vi "TelemetryPRO-2_XCAN.vi"() -> ()   [LabVIEW 2017]
uses:
  <vilib>/Platform/TimedLoop/XDataNode/timing_clust.ctl
  <vilib>/Platform/TimedLoop/XDataNode/nitl_modes.ctl
  <vilib>/Platform/TimedLoop/XDataNode/wakeup.ctl
  <vilib>/nican/nican.llb/ncNetAttr.ctl
  <vilib>/Utility/file.llb/Read From Spreadsheet File (string).vi
  <vilib>/xnet/xnet.llb/XNET Create Session (Frame Input Stream).vi
  <vilib>/xnet/xnet.llb/XNET Read (Frame CAN).vi
  <vilib>/Utility/file.llb/Write To Spreadsheet File (string).vi
  <vilib>/Platform/TimedLoop/XDataNode/XDataNode.xnode
  <resource>/objmgr/xnet.rc
  <vilib>/Platform/TimedLoop/XDataNode/XDNodeRunTimeDep.lvlib
panel:
  out "GasPedal Heartbeat":dbl format="%.2f"
  out "Brake Force":u16(slide) scale=0.0..1500.0
  out "Brake Force":u16
  out "BP_rear":i16
  out "BP_front":i16
  out "Front / Rear Brake Pressure":cluster{u16, u16}
  out "Negative Torque Demand":u8
  out "Raw Negative Torque":u8
  out "BrakeForce":u8
  out "Cones3 2":T1(array[cluster])
  out "Cones2 2":T1(array[cluster])
  out "Cones1 2":T1(array[cluster])
  out "(hi.lo) 3":u64 format="%064b"
  out "Cones3":T1(array[cluster])
  out "(hi.lo) 2":u64 format="%064b"
  out "Cones2":T1(array[cluster])
  in  "ConeType":cluster{"Col":dbl, "X":dbl, "Y":dbl}
  out "(hi.lo)":u64 format="%064b"
  out "Cones1":T1(array[cluster])
  out "IGBT Temperature":T2(graph)
  out "XY Graph 4":cluster{"X":dbl, "Y":dbl}[](graph)
  out "Array":u8[](array[numeric])
  out "Numeric 2":u8
  out "SlipControl_Enabled":bool
  out "AMK_AV":bool
  out "Torque 2":bool
  out "BreakPoint":u8
  out "Slope":u16
  out "Damper Travel FR [mm]":dbl
  out "Damper Travel RR [mm]":dbl
  out "Damper Travel FL [mm]":dbl
  in  "Wheel Travel FR":dbl=1000.0
  in  "Wheel Travel FL Offset":dbl=1000.0
  in  "Wheel Travel RR Offset":dbl=1000.0
  out "Damper Travel RL [mm]":dbl
  in  "Wheel Travel RL Offset":dbl=1000.0
  out "HV Cell Voltage":u16(graph)
  out "accY 2":dbl
  out "accZ 2":dbl
  out "TorqRaw 2":u16
  in  "Brake Min 3":dbl=426.0
  out "BPRV":bool
  out "BPFV":bool
  out "BPFV":bool
  out "BPFSV":bool
  out "STA2":bool
  out "STA1":bool
  out "TPS2V":bool
  out "TPS1V":bool
  out "Apps2":dbl
  out "Apps1":dbl
  out "APPS1":u8(slide) scale=0.0..100.0
  out "APPS2":u8(slide) scale=0.0..100.0
  out "Brake Pedal Fore Supply":dbl
  out "Brake Pedal Force":dbl
  in  "CAN1 Enable 2":bool
  in  "CAN0 Enable 2":bool
  out "Status LEDs Red":bool[](array[boolean])
  out "Status LEDs Green":bool[](array[boolean])
  out "Numeric":dbl
  out "TCU speed":cluster{dbl, "AccelXRaw":dbl, dbl}(graph)
  out "AccelYRaw":dbl
  out "AccelXRaw":dbl
  in  "Acc Y offset":dbl
  in  "Acc X offset 2":dbl
  in  "OffsetFilter":dbl=0.01
  out "IsStopped":bool
  out "Acc Z 2":dbl
  out "Acc X 2":dbl
  out "Roll 2":dbl
  out "Acc Y 2":dbl
  out "Yaw 2":dbl
  in  "Acc Z offset":dbl
  out "Vel_acc":dbl=-0.0098098
  in  "New Lap":bool
  out "Energy":dbl[](array[numeric])
  out "Wheel Travel FL":u16
  out "Wheel Travel FR":u16
  out "Wheel Travel RL":u16
  out "Wheel Travel RR":u16
  out "Acc X":dbl
  out "Roll":dbl
  out "Yaw":dbl
  out "Acc Y":dbl
  out "Acc Z":dbl
  out "accY":dbl
  out "accZ":dbl
  out "Intensity Graph":dbl[][](graph)
  in  "Rollrate offset":dbl
  out "XY Graph 2":cluster{dbl[], dbl[]}(graph)
  out "Derate":bool[](array[boolean])
  out "Torq_sum":dbl
  in  "Play":bool
  in  "Timestep":u32
  in  "stop":bool
  in  "start":bool
  in  "pause":bool
  in  "Progress":i32(slide) min=0 step=60 scale=-1.0..61354011.0 scale format="%.0p"
  out "Time Stamp":string="2\r\n60"
  out "Charge Voltage":dbl
  out "Charge Curr":dbl
  in  "Tab Control":T3(tab)
  in  "Rows to read":i32=60
  in  "Data Path":path=path "D:/__BME-FRT/2016/2016-05-19/2016_05_19_tokol_endurance_00005_00001.csv"
  in  "CAN1 Enable":bool
  in  "CAN0 Enable":bool
  in  "Data Source":u16(ring) items=["Wi-Fi", "CAN-USB", "Log Analysis", "XCAN-USB"]
  in  "Port":u16=8998
  in  "Exit":bool
  in  "Log Path":path=path "D:/__BME-FRT/2016/test.txt"
  in  "Log Enable":bool
  out "WiFi Error":errorcluster
  in  "Length":u16=10
  out "CAN0 Error":errorcluster
  out "CAN1 Error":errorcluster
  out "Log Error":errorcluster
  out "CAN Message":u8[][](array[numeric])=[[2, 1, 128, 63, 0, 0, 129, 162, 129, 155], [2, 17, 23, 61, 0, 1, 0, 0, 0, 0], [3, 64, 252, 0, 0, 0, 27, 55, 27, 0], [2, 16, 115, 16, 37, 0, 203, 0, 0, 0], [4, 17, 23, 61, 0, 1, 0, 0, 0, 0], [2, 0, 128, 44, 0, 0, 136, 1, 7, 207], [2, 1, 128, 63, 0, 0, 129, 162, 129, 155], [2, 17, 23, 61, 0, 1, 0, 0, 0, 0], [4, 34, 0, 33, 0, 30, 0, 0, 0, 0], [4, 80, 148, 60, 128, 0, 0, 0, 0, 0], [1, 116, 84, 128, 0, 0, 190, 127, 8, 37], [2, 16, 116, 15, 111, 0, 203, 0, 0, 0], [1, 120, 211, 127, 0, 0, 193, 158, 8, 215], [1, 180, 84, 128, 0, 0, 223, 126, 2, 100], [1, 124, 0, 0, 0, 0, 189, 126, 8, 75], [1, 184, 62, 128, 2, 15, 59, 127, 2, 219], [4, 17, 23, 61, 0, 1, 0, 0, 0, 0], [1, 188, 0, 0, 0, 0, 136, 158, 2, 110], [2, 0, 128, 44, 0, 0, 136, 1, 7, 207], [2, 1, 128, 63, 0, 0, 129, 162, 129, 155], [2, 17, 23, 61, 0, 1, 0, 0, 0, 0], [3, 64, 252, 0, 0, 0, 27, 55, 27, 0], [4, 48, 10, 15, 219, 0, 96, 0, 0, 0], [3, 49, 128, 255, 0, 0, 0, 0, 0, 0], [2, 16, 117, 0, 0, 0, 203, 0, 0, 0], [4, 17, 23, 61, 0, 1, 0, 0, 0, 0], [2, 0, 128, 44, 0, 0, 136, 1, 7, 207], [2, 1, 128, 63, 0, 0, 129, 162, 129, 155], [2, 17, 23, 61, 0, 1, 0, 0, 0, 0], [3, 32, 112, 255, 0, 0, 0, 0, 0, 0], [4, 34, 0, 30, 0, 31, 0, 0, 0, 0], [1, 116, 87, 128, 0, 0, 184, 127, 9, 218], [1, 120, 203, 127, 1, 37, 194, 158, 9, 222], [2, 16, 118, 0, 0, 0, 205, 0, 0, 0], [1, 124, 0, 0, 0, 0, 176, 126, 9, 211], [1, 180, 90, 128, 0, 0, 215, 126, 3, 116], [1, 184, 50, 128, 3, 19, 44, 127, 3, 114], [4, 17, 23, 61, 0, 1, 0, 0, 0, 0], [1, 188, 0, 0, 0, 0, 147, 158, 3, 235], [2, 0, 128, 43, 0, 0, 136, 1, 7, 207], [2, 1, 128, 63, 0, 0, 129, 162, 129, 155], [2, 17, 23, 61, 0, 1, 0, 0, 0, 0], [3, 64, 252, 0, 0, 0, 38, 55, 38, 0], [2, 16, 119, 0, 0, 0, 202, 0, 0, 0], [4, 17, 23, 61, 0, 1, 0, 0, 0, 0], [2, 0, 128, 43, 0, 0, 136, 2, 7, 207], [2, 1, 128, 63, 0, 0, 129, 162, 129, 155], [2, 17, 23, 61, 0, 1, 0, 0, 0, 0], [4, 34, 0, 20, 0, 26, 0, 0, 0, 0], [1, 116, 78, 128, 0, 0, 179, 127, 10, 75], [1, 120, 206, 127, 2, 57, 194, 158, 10, 132], [2, 16, 120, 16, 37, 0, 200, 0, 210, 0], [1, 180, 90, 128, 0, 0, 206, 126, 4, 188], [1, 124, 0, 0, 0, 0, 157, 126, 10, 65], [1, 184, 39, 128, 4, 3, 33, 127, 4, 7], [4, 17, 23, 61, 0, 1, 0, 0, 0, 0], [1, 188, 0, 0, 0, 0, 153, 158, 4, 183], [2, 0, 128, 43, 0, 0, 136, 2, 7, 207], [2, 1, 128, 63, 0, 0, 129, 162, 129, 155], [2, 17, 23, 61, 0, 1, 0, 0, 0, 0]] format="%02x"
  out "CAN ID":u16[](array[numeric])=[513, 529, 832, 528, 1041, 512, 513, 529, 1058, 1104, 372, 528, 376, 436, 380, 440, 1041, 444, 512, 513, 529, 832, 1072, 817, 528, 1041, 512, 513, 529, 800, 1058, 372, 376, 528, 380, 436, 440, 1041, 444, 512, 513, 529, 832, 528, 1041, 512, 513, 529, 1058, 372, 376, 528, 436, 380, 440, 1041, 444, 512, 513, 529] format="%x"
  out "CAN Message 2":u8[][](array[numeric])=[[2, 1, 128, 63, 0, 0, 129, 162, 129, 155], [2, 17, 23, 61, 0, 1, 0, 0, 0, 0], [3, 64, 252, 0, 0, 0, 27, 55, 27, 0], [2, 16, 115, 16, 37, 0, 203, 0, 0, 0], [4, 17, 23, 61, 0, 1, 0, 0, 0, 0], [2, 0, 128, 44, 0, 0, 136, 1, 7, 207], [2, 1, 128, 63, 0, 0, 129, 162, 129, 155], [2, 17, 23, 61, 0, 1, 0, 0, 0, 0], [4, 34, 0, 33, 0, 30, 0, 0, 0, 0], [4, 80, 148, 60, 128, 0, 0, 0, 0, 0], [1, 116, 84, 128, 0, 0, 190, 127, 8, 37], [2, 16, 116, 15, 111, 0, 203, 0, 0, 0], [1, 120, 211, 127, 0, 0, 193, 158, 8, 215], [1, 180, 84, 128, 0, 0, 223, 126, 2, 100], [1, 124, 0, 0, 0, 0, 189, 126, 8, 75], [1, 184, 62, 128, 2, 15, 59, 127, 2, 219], [4, 17, 23, 61, 0, 1, 0, 0, 0, 0], [1, 188, 0, 0, 0, 0, 136, 158, 2, 110], [2, 0, 128, 44, 0, 0, 136, 1, 7, 207], [2, 1, 128, 63, 0, 0, 129, 162, 129, 155], [2, 17, 23, 61, 0, 1, 0, 0, 0, 0], [3, 64, 252, 0, 0, 0, 27, 55, 27, 0], [4, 48, 10, 15, 219, 0, 96, 0, 0, 0], [3, 49, 128, 255, 0, 0, 0, 0, 0, 0], [2, 16, 117, 0, 0, 0, 203, 0, 0, 0], [4, 17, 23, 61, 0, 1, 0, 0, 0, 0], [2, 0, 128, 44, 0, 0, 136, 1, 7, 207], [2, 1, 128, 63, 0, 0, 129, 162, 129, 155], [2, 17, 23, 61, 0, 1, 0, 0, 0, 0], [3, 32, 112, 255, 0, 0, 0, 0, 0, 0], [4, 34, 0, 30, 0, 31, 0, 0, 0, 0], [1, 116, 87, 128, 0, 0, 184, 127, 9, 218], [1, 120, 203, 127, 1, 37, 194, 158, 9, 222], [2, 16, 118, 0, 0, 0, 205, 0, 0, 0], [1, 124, 0, 0, 0, 0, 176, 126, 9, 211], [1, 180, 90, 128, 0, 0, 215, 126, 3, 116], [1, 184, 50, 128, 3, 19, 44, 127, 3, 114], [4, 17, 23, 61, 0, 1, 0, 0, 0, 0], [1, 188, 0, 0, 0, 0, 147, 158, 3, 235], [2, 0, 128, 43, 0, 0, 136, 1, 7, 207], [2, 1, 128, 63, 0, 0, 129, 162, 129, 155], [2, 17, 23, 61, 0, 1, 0, 0, 0, 0], [3, 64, 252, 0, 0, 0, 38, 55, 38, 0], [2, 16, 119, 0, 0, 0, 202, 0, 0, 0], [4, 17, 23, 61, 0, 1, 0, 0, 0, 0], [2, 0, 128, 43, 0, 0, 136, 2, 7, 207], [2, 1, 128, 63, 0, 0, 129, 162, 129, 155], [2, 17, 23, 61, 0, 1, 0, 0, 0, 0], [4, 34, 0, 20, 0, 26, 0, 0, 0, 0], [1, 116, 78, 128, 0, 0, 179, 127, 10, 75], [1, 120, 206, 127, 2, 57, 194, 158, 10, 132], [2, 16, 120, 16, 37, 0, 200, 0, 210, 0], [1, 180, 90, 128, 0, 0, 206, 126, 4, 188], [1, 124, 0, 0, 0, 0, 157, 126, 10, 65], [1, 184, 39, 128, 4, 3, 33, 127, 4, 7], [4, 17, 23, 61, 0, 1, 0, 0, 0, 0], [1, 188, 0, 0, 0, 0, 153, 158, 4, 183], [2, 0, 128, 43, 0, 0, 136, 2, 7, 207], [2, 1, 128, 63, 0, 0, 129, 162, 129, 155], [2, 17, 23, 61, 0, 1, 0, 0, 0, 0]] format="%02x"
  out "CAN ID 2":u16[](array[numeric])=[513, 529, 832, 528, 1041, 512, 513, 529, 1058, 1104, 372, 528, 376, 436, 380, 440, 1041, 444, 512, 513, 529, 832, 1072, 817, 528, 1041, 512, 513, 529, 800, 1058, 372, 376, 528, 380, 436, 440, 1041, 444, 512, 513, 529, 832, 528, 1041, 512, 513, 529, 1058, 372, 376, 528, 436, 380, 440, 1041, 444, 512, 513, 529] format="%x"
  out "CAN Message 3":u8[][](array[numeric])=[[2, 1, 128, 63, 0, 0, 129, 162, 129, 155], [2, 17, 23, 61, 0, 1, 0, 0, 0, 0], [3, 64, 252, 0, 0, 0, 27, 55, 27, 0], [2, 16, 115, 16, 37, 0, 203, 0, 0, 0], [4, 17, 23, 61, 0, 1, 0, 0, 0, 0], [2, 0, 128, 44, 0, 0, 136, 1, 7, 207], [2, 1, 128, 63, 0, 0, 129, 162, 129, 155], [2, 17, 23, 61, 0, 1, 0, 0, 0, 0], [4, 34, 0, 33, 0, 30, 0, 0, 0, 0], [4, 80, 148, 60, 128, 0, 0, 0, 0, 0], [1, 116, 84, 128, 0, 0, 190, 127, 8, 37], [2, 16, 116, 15, 111, 0, 203, 0, 0, 0], [1, 120, 211, 127, 0, 0, 193, 158, 8, 215], [1, 180, 84, 128, 0, 0, 223, 126, 2, 100], [1, 124, 0, 0, 0, 0, 189, 126, 8, 75], [1, 184, 62, 128, 2, 15, 59, 127, 2, 219], [4, 17, 23, 61, 0, 1, 0, 0, 0, 0], [1, 188, 0, 0, 0, 0, 136, 158, 2, 110], [2, 0, 128, 44, 0, 0, 136, 1, 7, 207], [2, 1, 128, 63, 0, 0, 129, 162, 129, 155], [2, 17, 23, 61, 0, 1, 0, 0, 0, 0], [3, 64, 252, 0, 0, 0, 27, 55, 27, 0], [4, 48, 10, 15, 219, 0, 96, 0, 0, 0], [3, 49, 128, 255, 0, 0, 0, 0, 0, 0], [2, 16, 117, 0, 0, 0, 203, 0, 0, 0], [4, 17, 23, 61, 0, 1, 0, 0, 0, 0], [2, 0, 128, 44, 0, 0, 136, 1, 7, 207], [2, 1, 128, 63, 0, 0, 129, 162, 129, 155], [2, 17, 23, 61, 0, 1, 0, 0, 0, 0], [3, 32, 112, 255, 0, 0, 0, 0, 0, 0], [4, 34, 0, 30, 0, 31, 0, 0, 0, 0], [1, 116, 87, 128, 0, 0, 184, 127, 9, 218], [1, 120, 203, 127, 1, 37, 194, 158, 9, 222], [2, 16, 118, 0, 0, 0, 205, 0, 0, 0], [1, 124, 0, 0, 0, 0, 176, 126, 9, 211], [1, 180, 90, 128, 0, 0, 215, 126, 3, 116], [1, 184, 50, 128, 3, 19, 44, 127, 3, 114], [4, 17, 23, 61, 0, 1, 0, 0, 0, 0], [1, 188, 0, 0, 0, 0, 147, 158, 3, 235], [2, 0, 128, 43, 0, 0, 136, 1, 7, 207], [2, 1, 128, 63, 0, 0, 129, 162, 129, 155], [2, 17, 23, 61, 0, 1, 0, 0, 0, 0], [3, 64, 252, 0, 0, 0, 38, 55, 38, 0], [2, 16, 119, 0, 0, 0, 202, 0, 0, 0], [4, 17, 23, 61, 0, 1, 0, 0, 0, 0], [2, 0, 128, 43, 0, 0, 136, 2, 7, 207], [2, 1, 128, 63, 0, 0, 129, 162, 129, 155], [2, 17, 23, 61, 0, 1, 0, 0, 0, 0], [4, 34, 0, 20, 0, 26, 0, 0, 0, 0], [1, 116, 78, 128, 0, 0, 179, 127, 10, 75], [1, 120, 206, 127, 2, 57, 194, 158, 10, 132], [2, 16, 120, 16, 37, 0, 200, 0, 210, 0], [1, 180, 90, 128, 0, 0, 206, 126, 4, 188], [1, 124, 0, 0, 0, 0, 157, 126, 10, 65], [1, 184, 39, 128, 4, 3, 33, 127, 4, 7], [4, 17, 23, 61, 0, 1, 0, 0, 0, 0], [1, 188, 0, 0, 0, 0, 153, 158, 4, 183], [2, 0, 128, 43, 0, 0, 136, 2, 7, 207], [2, 1, 128, 63, 0, 0, 129, 162, 129, 155], [2, 17, 23, 61, 0, 1, 0, 0, 0, 0]] format="%02x"
  out "CAN ID 3":u16[](array[numeric])=[513, 529, 832, 528, 1041, 512, 513, 529, 1058, 1104, 372, 528, 376, 436, 380, 440, 1041, 444, 512, 513, 529, 832, 1072, 817, 528, 1041, 512, 513, 529, 800, 1058, 372, 376, 528, 380, 436, 440, 1041, 444, 512, 513, 529, 832, 528, 1041, 512, 513, 529, 1058, 372, 376, 528, 436, 380, 440, 1041, 444, 512, 513, 529] format="%x"
  out "STA2":i16
  out "STA1":i16
  out "Max Power":u8
  out "TPS1_Raw":u16
  out "BPS1_Raw":u16
  out "K_Brake":dbl
  out "PD Error Info":u8
  out "Velocity [km/h]":dbl(knob) scale=0.0..120.0
  out "CAN Missing Message":u8[](array[numeric])
  out "Rear 2":dbl
  out "Front 2":dbl
  out "TCU FR":dbl(graph)
  out "TCU RR":dbl(graph)
  out "TCU FL":dbl(graph)
  out "Rear":dbl
  out "Front":dbl
  out "Torque":dbl(slide) scale=0.0..100.0
  out "Brake Encoder":dbl(slide) scale=0.0..2000.0
  out "FL":dbl(slide) scale=0.0..2330.0
  in  "Torque Min":dbl
  in  "Torque Max":dbl=1000.0
  in  "Brake Min":dbl
  in  "Brake Max":dbl=1000.0
  out "FL 2":dbl(slide)
  out "FR":dbl(slide) scale=0.0..2330.0
  out "FR 2":dbl(slide)
  out "RL":dbl(slide) scale=0.0..2330.0
  out "RL 2":dbl(slide)
  out "RR":dbl(slide) scale=0.0..2330.0
  out "RR 2":dbl(slide)
  out "Sensor Check":bool[](array[boolean])
  out "Brake Front":dbl(slide)=-0.5082592121982211 scale=0.0..100.0
  out "Brake Rear":dbl(slide)=-0.9529860228716646 scale=0.0..100.0
  in  "Brake Min 2":dbl=460.0
  in  "Brake Max 2":dbl=2000.0
  out "TorqRaw":u16
  out "BrakeRaw":u16
  out "BrakeRaw 2":u16
  out "Boolean":bool
  out "Boolean 2":bool
  out "Boolean 3":bool
  out "Boolean 4":bool
  out "Dial":dbl(knob)=3.0 scale=1.0..12.0
  out "Dial 2":dbl(knob)=11.0 scale=1.0..12.0
  out "Dial 3":dbl(knob)=9.0 scale=1.0..12.0
  out "Dial 4":dbl(knob)=1.0 scale=1.0..12.0
  out "Dial 5":dbl(knob)=1.0 scale=1.0..12.0
  out "Selector":u8
  out "Torque %":u8
  out "Speed RPM":i16
  out "LR Bias":dbl
  out "Regen %":u8
  out "BTC":u8
  out "TCU RR Status":bool[](array[boolean])
  out "TCU RL Status":bool[](array[boolean])
  out "TCU FR Status":bool[](array[boolean])
  out "TCU FL Status":bool[](array[boolean])
  out "Torque [Nm]":dbl(knob) scale=-500.0..1250.0
  out "XY Graph":cluster{dbl[], dbl[]}[](graph)
  out "TCU RL":dbl(graph)
  out "K_Throttle":dbl
  out "BPS2_Raw":u16
  out "BPF_Raw":u16
  out "BPR_Raw":u16
  out "TPS2_Raw":u16
  out "STA2_Raw":u16
  out "STA1_Raw":u16
  out "OFF":bool=TRUE
  out "START":bool
  out "ON":bool
  in  "Steering Null":dbl=1919.0
  in  "Steering Min":dbl=174.0
  in  "Steering Max":dbl=3565.0
  out "Steering Angle":dbl(slide)=-0.10285714285714287 scale=90.0..-90.0
  out "SteeringRaw":u16
  out "TCU Version":u16
  out "Safety Mode Enabled":bool
  out "Keylock Enable":bool
  out "PPS1":i16
  out "PPS2":i16
  out "Logging":bool
  out "Force based":bool
  out "Pressure based":bool
  out "Slip_TCU":cluster{dbl, dbl, dbl, dbl}(graph)
  out "TCU_acc":cluster{dbl[], dbl[]}[](graph)
  out "Slip":cluster{dbl, dbl, dbl, dbl}(graph)
  out "TCU_ay":dbl
  out "TCU_v":dbl
  out "TCU_ax":dbl
  out "TCU_yaw":dbl
  out "TCU_slipFL":dbl
  out "TCU_slipFR":dbl
  out "TCU_slipRL":dbl
  out "TCU_slipRR":dbl
  out "FL Velocity":dbl
  out "FL Torque Pos":dbl
  out "FL Torque Neg":dbl
  out "FR Velocity":dbl
  out "FR Torque Pos":dbl
  out "FR Torque Neg":dbl
  out "RL Velocity":dbl
  out "RL Torque Pos":dbl
  out "RL Torque Neg":dbl
  out "RR Velocity":dbl
  out "RR Torque Pos":dbl
  out "RR Torque Neg":dbl
  out "MCU RR":cluster{dbl, dbl}(graph)={-0.487060546875, 0.57037353515625}
  out "MCU RL":cluster{dbl, dbl}(graph)={0.743408203125, -0.384521484375}
  out "MCU FR":cluster{dbl, dbl}(graph)={-0.25634765625, -0.205078125}
  out "MCU FL":cluster{dbl, dbl}(graph)={-0.16021728515625, 0.50628662109375}
  out "Actual Velocity\nFL [RPM]":i16
  out "Id FL [A]":dbl
  out "Iq FL [A]":dbl
  out "T Motor FL [°C]":dbl
  out "Error Info FL":u16
  out "Actual Velocity\nFR [RPM]":i16
  out "Id FR [A]":dbl
  out "Iq FR [A]":dbl
  out "Actual Velocity\nRL [RPM]":i16
  out "Id RL [A]":dbl
  out "Iq RL [A]":dbl
  out "Actual Velocity \nRR [RPM]":i16
  out "Id RR [A]":dbl
  out "Iq RR [A]":dbl
  out "Error Info FR":u16
  out "T Motor FR [°C]":dbl
  out "Error Info RL":u16
  out "T Motor RL [°C]":dbl
  out "Error Info RR":u16
  out "T Motor RR [°C]":dbl
  out "Status FL":bool[](array[boolean])
  out "Status FR":bool[](array[boolean])
  out "Status RL":bool[](array[boolean])
  out "Status RR":bool[](array[boolean])
  out "T Inv. FL [°C]":dbl
  out "T Inv. FR [°C]":dbl
  out "T Inv. RR [°C]":dbl
  out "T Inv. RL [°C]":dbl
  out "IGBT FL TEMP":i16
  out "IGBT FR TEMP":dbl
  out "IGBT RL TEMP":dbl
  out "IGBT RR TEMP":dbl
  out "MCU SC Endline":bool
  out "HVD Interlock":bool
  out "Motor4 Interlock":bool
  out "Motor3 Interlock":bool
  out "Motor2 Interlock":bool
  out "Motor1 Interlock":bool
  out "SC LKS":bool
  out "SC RKS":bool
  out "SC MCU":bool
  out "SC 12V":bool
  out "SC IMD":bool
  out "SC AMS":bool
  out "SC AIR-":bool
  out "SC AIR+":bool
  out "SC BOTS &\nINS & CKS":bool
  out "SC Motor 3":bool
  out "SC Motor 1":bool
  out "SC Motor 4":bool
  out "SC Motor 2":bool
  out "HVDet":bool
  out "AIR-":bool
  out "AIR+":bool
  out "BOTS & INS & CKS":bool
  out "MCU Interlocks":bool
  out "LKS & RKS":bool
  out "HV_ACC in menu":bool
  out "AMS Relay":bool
  out "IMD Relay":bool
  out "SC Endline":bool
  out "Radiator Cooling":bool
  out "Battery Low":bool
  out "BMS IC Wake":bool
  out "BMS IC Fault":bool
  out "48V Out 5":bool
  out "Battery Full":bool
  out "48V Out 3":bool
  out "48V Out 4":bool
  out "Undervoltage 3":bool
  out "Overtemp. 3":bool
  out "Logging Status":bool
  out "Radio CS":bool
  out "12V Out 2":bool
  out "12V Out 3":bool
  out "SC State":bool
  out "12V Out 1":bool
  out "Main Switch":bool
  out "MP Switch":bool
  out "12V Out 5":bool
  out "12V Out 4":bool
  out "48V Out 2":bool
  out "48V Out 1":bool
  out "Discharge":bool[](array[boolean])
  out "LV Temp":dbl[](array[numeric])
  out "LV Battery":cluster{"CellSlide":u16, "CellVoltage":u16}[](array[cluster])=[{"CellSlide"=0, "CellVoltage"=0}, {"CellSlide"=0, "CellVoltage"=0}, {"CellSlide"=0, "CellVoltage"=0}, {"CellSlide"=0, "CellVoltage"=0}, {"CellSlide"=0, "CellVoltage"=0}, {"CellSlide"=0, "CellVoltage"=0}, {"CellSlide"=0, "CellVoltage"=0}, {"CellSlide"=0, "CellVoltage"=0}, {"CellSlide"=0, "CellVoltage"=0}, {"CellSlide"=2800, "CellVoltage"=0}, {"CellSlide"=0, "CellVoltage"=0}, {"CellSlide"=0, "CellVoltage"=0}, {"CellSlide"=0, "CellVoltage"=0}, {"CellSlide"=0, "CellVoltage"=0}] {"CellSlide" scale=2800.0..4200.0}
  out "LV Temp":dbl
  out "LV Max":u16
  out "LV Min":u16
  out "LV Cell Voltages":T4(graph)
  out "Overtemp Errors":u16
  out "Undervoltage Errrors":u16
  out "LV Current":cluster{dbl, dbl}(graph)
  out "LV Voltage [V]":dbl format="%#.2g"
  out "12V Current [A]":dbl format="%#.1g"
  out "48V Current [A]":dbl format="%#.1g"
  in  "LV Max Limit":u16=4150
  in  "LV Min Limit":u16=3700
  in  "Enable LV alert":bool
  out "Temp Max 2":dbl
  out "Cell Min 2":u16
  out "HVDet":bool
  out "Stack 1":cluster{"CellSlide":u16, "CellVoltage":u16}[](array[cluster]) {"CellSlide" scale=2800.0..4200.0}
  out "Temp 1":dbl[](array[numeric])
  out "Cell Min":u16
  out "Cell Max":u16
  out "Temp Max":dbl
  out "HV Before":dbl
  out "HV After":dbl
  out "HV Current":dbl
  out "SoC [mAh]":dbl
  out "Stack 2":cluster{"CellSlide":u16, "CellVoltage":u16}[](array[cluster]) {"CellSlide" scale=2800.0..4200.0}
  out "Stack 3":cluster{"CellSlide":u16, "CellVoltage":u16}[](array[cluster]) {"CellSlide" scale=2800.0..4200.0}
  out "Stack 4":cluster{"CellSlide":u16, "CellVoltage":u16}[](array[cluster])=[{"CellSlide"=0, "CellVoltage"=0}, {"CellSlide"=0, "CellVoltage"=0}, {"CellSlide"=0, "CellVoltage"=0}, {"CellSlide"=0, "CellVoltage"=0}, {"CellSlide"=0, "CellVoltage"=0}, {"CellSlide"=0, "CellVoltage"=0}, {"CellSlide"=0, "CellVoltage"=0}, {"CellSlide"=0, "CellVoltage"=0}, {"CellSlide"=0, "CellVoltage"=0}, {"CellSlide"=0, "CellVoltage"=0}, {"CellSlide"=0, "CellVoltage"=0}, {"CellSlide"=0, "CellVoltage"=0}, {"CellSlide"=0, "CellVoltage"=0}, {"CellSlide"=0, "CellVoltage"=0}, {"CellSlide"=0, "CellVoltage"=0}, {"CellSlide"=0, "CellVoltage"=0}, {"CellSlide"=0, "CellVoltage"=0}, {"CellSlide"=0, "CellVoltage"=0}, {"CellSlide"=0, "CellVoltage"=0}, {"CellSlide"=0, "CellVoltage"=0}, {"CellSlide"=0, "CellVoltage"=0}, {"CellSlide"=0, "CellVoltage"=0}, {"CellSlide"=2800, "CellVoltage"=0}, {"CellSlide"=2800, "CellVoltage"=0}] {"CellSlide" scale=2800.0..4200.0}
  out "Stack 5":cluster{"CellSlide":u16, "CellVoltage":u16}[](array[cluster])=[{"CellSlide"=2800, "CellVoltage"=0}, {"CellSlide"=0, "CellVoltage"=0}, {"CellSlide"=0, "CellVoltage"=0}, {"CellSlide"=0, "CellVoltage"=0}, {"CellSlide"=0, "CellVoltage"=0}, {"CellSlide"=0, "CellVoltage"=0}, {"CellSlide"=0, "CellVoltage"=0}, {"CellSlide"=0, "CellVoltage"=0}, {"CellSlide"=0, "CellVoltage"=0}, {"CellSlide"=0, "CellVoltage"=0}, {"CellSlide"=0, "CellVoltage"=0}, {"CellSlide"=0, "CellVoltage"=0}, {"CellSlide"=0, "CellVoltage"=0}, {"CellSlide"=0, "CellVoltage"=0}, {"CellSlide"=0, "CellVoltage"=0}, {"CellSlide"=0, "CellVoltage"=0}, {"CellSlide"=0, "CellVoltage"=0}, {"CellSlide"=0, "CellVoltage"=0}, {"CellSlide"=0, "CellVoltage"=0}, {"CellSlide"=0, "CellVoltage"=0}, {"CellSlide"=0, "CellVoltage"=0}, {"CellSlide"=0, "CellVoltage"=0}, {"CellSlide"=0, "CellVoltage"=0}, {"CellSlide"=0, "CellVoltage"=0}] {"CellSlide" scale=2800.0..4200.0}
  out "Stack 6":cluster{"CellSlide":u16, "CellVoltage":u16}[](array[cluster]) {"CellSlide" scale=2800.0..4200.0}
  out "Temp 2":dbl[](array[numeric])
  out "Temp 3":dbl[](array[numeric])
  out "Temp 4":dbl[](array[numeric])
  out "Temp 5":dbl[](array[numeric])
  out "Temp 6":dbl[](array[numeric])
  out "TSAL State":bool
  out "PC State":bool
  out "12V State":bool
  out "AMS error":bool
  out "IMD error":bool
  out "AMS Relay 2":bool
  out "IMD Relay":bool
  out "AIR+":bool
  out "AIR-":bool
  out "UV":bool
  out "OV":bool
  out "OT":bool
  out "TS-OV":bool
  out "Place of Error":u16
  out "Value":u16
  out "TSAL Green":bool
  out "TSAL Red":bool
  out "MCU HVDET":bool
  out "TSAL Error":bool
  out "TS-OC":bool
  out "PC":bool
  in  "Enable HV alert":bool
  in  "HV Max Limit":u16=4150
  in  "HV Min Limit":u16=3700
  out "Charger state":string
  out "?":T5(graph)
  out "Angular Speed":T6(graph)
  out "Pedal Signals":cluster{u16, "BrakeRaw":u16}(graph)
  out "Brake Pressure":T7(graph)
  out "XY Graph 3":cluster{dbl[], dbl[]}[](graph)
  out "HV Cell":cluster{"Cell Max":u16, "Cell Min":u16}(graph)
  out "Current":dbl(graph)
  out "Electric Power":cluster{dbl, dbl}(graph)
  out "HV Voltage":cluster{"HV Before":dbl, "HV After":dbl}(graph)={"HV Before"=594.9, "HV After"=0.1}
  out "HV Cell Temperature":cluster{dbl, dbl}(graph)
  out "Motor Temperature":cluster{dbl, dbl, dbl, dbl}(graph)={1.3, 1.3, 1.6, 1.5}
  out "Inverter Temperature":cluster{dbl, dbl, dbl, dbl}(graph)={1.3, 1.3, 1.6, 1.5}
  out "Radiator Temperature":cluster{dbl, dbl, dbl, dbl}(graph)={1.3, 1.3, 1.6, 1.5}
  out "Dash Heartbeat":dbl
  out "Overvoltage":bool
  out "MODE":bool
  out "XLAT":bool
  out "BLANK":bool
  out "MCU S SC Endl":u16
  out "SD CS":bool
  out "Radio CS":bool
  out "XBee CS":bool
  out "TSAL":bool
  out "Logging":bool
  out "OFF":bool
  out "START":bool
  out "24V rear DC/DC":bool
  out "OFF Button":bool
  out "START Button":bool
  out "ON Button":bool
  out "Power B Current":u32
  out "Power A Current":u32
  out "CAN2 Term.":bool
  out "CAN1 Term.":bool
  out "MCU TSAL":bool
  out "MCU SC Endline 2":bool
  out "MCU FL 4":bool
  out "MCU FL 3":bool
  out "MCU FL 2":bool
  out "Brake Heartbeat":bool
  out "MCU RF 4":bool
  out "MCU RF 3":bool
  out "MCU RF 2":bool
  out "MCU RF 1":bool
  out "MCU EF2 B":bool
  out "MCU EF2 A":bool
  out "MCU EF B":bool
  out "MCU EF A":bool
  out "24V Power B":bool
  out "Braking":bool
  out "STA2 ADC Null":u16
  out "STA1 ADC Null":u16
  out "Battery Low 2":bool
  out "BMS IC Awake":bool
  out "BMS IC Error":bool
  out "48V Out 5 2":bool
  out "Battery Full 2":bool
  out "48V Out 3 2":bool
  out "48V Out 4 2":bool
  out "Undervoltage 4":bool
  out "Overtemp. 4":bool
  out "Logging Status":bool
  out "Radio CS":bool
  out "12V Out 2 2":bool
  out "12V Out 3 2":bool
  out "SC State 2":bool
  out "12V Out 1 2":bool
  out "Main Switch 2":bool
  out "MP Switch 2":bool
  out "12V Out 5 2":bool
  out "12V Out 4 2":bool
  out "48V Out 2 2":bool
  out "48V Out 1 2":bool
  out "ON":bool
  out "24V front DC/DC":bool
  out "MCU Interlock":bool
  out "TCU Power":bool
  out "RTDS":bool
  out "LKS & RKS":bool
  out "Brake Light":bool
  out "STA2 ADC 90":u16
  out "STA1 ADC 90":u16
  out "BSE2 ADC Max":u16
  out "BSE2 ADC Min":u16
  out "BSE1 ADC Max":u16
  out "BSE1 ADC Min":u16
  out "APPS2 ADC Max":u16
  out "APPS2 ADC Min":u16
  out "APPS1 ADC Max":u16
  out "APPS1 ADC Min":u16
  out "MCU EF":bool
  out "MCU RF":bool
  out "Radiator Left IN":dbl
  out "Radiator Right OUT":dbl
  out "Radiator Right IN":dbl
  out "Radiator Left OUT":dbl
  out "TSAL State 2":bool
  out "PC State 2":bool
  out "Driver Protection":bool
  out "12V Current [mA]":dbl
  out "48V Current [mA]":dbl
  out "Pedal Heartbeat":dbl
  out "Message Arrived 14":bool
  out "Message Arrived 13":bool
  out "Message Arrived 12":bool
  out "Message Arrived 11":bool
  out "Other messages arrived":bool
  out "Message Arrived 2":bool
  out "Message Arrived":bool
  out "RR TargetVelo OverTresh":bool
  out "RR TorqueLimNeg UnderTresh":bool
  out "RR TorqueLimNeg OverTresh":bool
  out "RR TorqueLimPos UnderTresh":bool
  out "RR TorqueLimPos OverTresh":bool
  out "RR TargetVelo UnderTresh":bool
  out "RL TargetVelo OverTresh":bool
  out "RL TorqueLimNeg UnderTresh":bool
  out "RL TorqueLimNeg OverTresh":bool
  out "RL TorqueLimPos UnderTresh":bool
  out "RL TorqueLimPos OverTresh":bool
  out "RL TargetVelo UnderTresh":bool
  out "FR TargetVelo OverTresh":bool
  out "FR TorqueLimNeg UnderTresh":bool
  out "FR TorqueLimNeg OverTresh":bool
  out "FR TorqueLimPos UnderTresh":bool
  out "FR TorqueLimPos OverTresh":bool
  out "FR TargetVelo UnderTresh":bool
  out "FL TargetVelo OverTresh":bool
  out "FL TorqueLimNeg UnderTresh":bool
  out "FL TorqueLimNeg OverTresh":bool
  out "FL TorqueLimPos UnderTresh":bool
  out "FL TorqueLimPos OverTresh":bool
  out "FL TargetVelo UnderTresh":bool
  out "Error Throttle Plausability":bool
  out "Error Throttle Validity 2":bool
  out "Error Throttle Validity 1":bool
  out "Error Throttle Position 2":bool
  out "Error Throttle Position 1":bool
  out "Error Rot Switch 5":bool
  out "Error Rot Switch 4":bool
  out "Error Rot Switch 3":bool
  out "Error Rot Switch 2":bool
  out "Error Rot Switch 1":bool
  out "Error Pedalbox Heartbeat":bool
  out "Error Steering Heartbeat":bool
  out "Error Brake Plausability":bool
  out "Error Brake Validity 2":bool
  out "Error Brake Validity  1":bool
  out "Error Brake Position 2":bool
  out "Error Brake Position 1":bool
  out "Error_Button_4":bool
  out "Error_Button_3":bool
  out "Error_Button_2":bool
  out "Error_Button_1":bool
  out "Error Steering Plausability":bool
  out "Error Steering Validity 2":bool
  out "Error Steering Validity 1":bool
  out "Error Steering Angle 2":bool
  out "Error Steering Angle 1":bool
  out "Error Cell Temperature":bool
  out "Error Cell Voltage Sensor":bool
  out "Error Cell Voltage":bool
  out "Error HV Accu. Current":bool
  out "Error HV Accu. Voltage":bool
  out "Error Actual Velocity RR":bool
  out "Error Actual Velocity RL":bool
  out "Error Actual Velocity FR":bool
  out "Error Actual Velocity FL":bool
  out "Error_SteeringControl_Heartbeat_raw":bool
  out "Error_Pedalbox_Heartbeat_raw":bool
  out "Error_SteeringAngleValidity_2_raw":bool
  out "Error_SteeringAngleValidity_1_raw":bool
  out "Error_ThrottleValidity_2_raw":bool
  out "Error_ThrottleValidity_1_raw":bool
  out "Error_BrakeValidity_2_raw":bool
  out "Error_BrakeValidity_1_raw":bool
  out "Error_LVCellTemperature":bool
  out "Error_LVCellVoltage":bool
  out "Error BrPressure Rear Validity_raw":bool
  out "Error BrPressure Front Validity_raw":bool
  out "Error BrPressure Rear 2":bool
  out "Error BrPressure Front":bool
  out "Error BrPressure Rear Validity":bool
  out "Error BrPressure Front Validity":bool
  out "CriticalHVCell Heartbeat":bool
  out "CriticalHVCell Heartbeat raw":bool
  out "Error_BrakeValidity_1_raw  2":bool
  out "Error_BrakeValidity_2_raw 2":bool
  out "Error_ThrottleValidity_1_raw 2":bool
  out "Error_ThrottleValidity_2_raw 2":bool
  out "Error_SteeringAngleValidity_1_raw 2":bool
  out "Error_SteeringAngleValidity_2_raw 2":bool
  out "SensorBox_Rear_RangeCheck":bool
  out "Sensorbox_Plausibility_Check":bool
  out "SensorBox_Front_RangeCheck":bool
  out "Fx_Bias":u8
  out "PowerLimiter Approx":dbl
  out "Hardcoremode ON":bool
  out "Smooth_Transition_Enabled":bool
  out "Drop":u8
  out "Torque_Derate":bool
  out "Torque_Coeff":bool
  out "Throttle_Constant":bool
  out "Power Limiter Enabled":bool
  out "Yaw Rear":dbl(graph)
  out "Yaw Front":dbl(graph)
  out "Slip":dbl(graph)
  out "Characteristics Approx":u8
  out "Tune":dbl
  out "Wheel Travel":cluster{"y_":dbl, "y_":dbl, "y_":dbl, "y_":dbl}(graph)
  out "Fz_FR":i32
  out "Fz_RL":i32
  out "Fz_FL":i32
  out "Fz_RR":i32
  out "YawControlSelector":i32
  out "Weight":i32
  out "P tag":dbl
  out "Yaw_Control_ON":bool
  out "Fx_Divide_ON":bool
  out "Power_Control":bool
  out "M_COG_Limit":dbl format="%.2f"
  out "M_COG":i32
  out "LaunchControl_Mu":dbl
  out "Brake_Threshold":u8
  out "TC_Param":u8
  out "Rear_Reduction":u8
  out "LaunchControl_Active":bool
  out "Target pos [°]":ext
  out "ASSI":T8(ring)
  out "EBS":T9(ring)
  out "AMI":T10(ring)
  out "ASMS":u8
  out "RES EBS":bool
  out "RES GO":bool
  out "RES BUTTON":bool
  out "Steering Angle":T11(graph)
  out "Actual pos [°]":ext
  out "Voltage enabled":bool
  out "Fault present":bool
  out "Operation enable":bool
  out "Switched on":bool
  out "Ready to switch on":bool
  out "Warning present":bool
  out "Switch on disabled":bool
  out "In operational NMT state":bool
  out "Target reached":bool
  out "Following error":bool
  out "Setpoint ack":bool
  out "Position referenced to home position":bool
  out "Actual pos [°] Maxon":ext
  in  "Reset":bool
  in  "Laptrigger":bool
  out "Motor Temp":cluster{i32[], dbl[]}[](graph)
  out "Inverter Temp":cluster{i32[], dbl[]}[](graph)
  out "Lap                    Laptime                        SoC                 Current Avg |                             Motor Temperatures                            |                            Inverter Temperatures":T12(array[cluster]) {"Laptime" format="%<%M:%S%2u>T"}
  out "Voltage Limit":dbl
  out "Current Limit":dbl
  # "SlipControl"
  # "HV    LV BPSD IMD AMS  FL    FR    RL   RR"
  # "SystemReady : 1 ha van 24V és felállt a belsõ rendszer\nError : 1 ha valamilyen error van\nWarn : 1 ha warning van\nQuitDcOn : DcOn visszajelzõje, hogy ténylegesen engedélyezte-e a HV-t, és hogy van is HV\nDcOn : TCU küldi CAN-en, hogy engedélyezze a HV bemenetet, CAN-en beolvasott értéket írja itt ki\nQuitInverterOn : az inverterek tényleges állapota, 1 ha aktívak, azaz a fizikai engedélyezõ jelek is aktívak\nInverterOn : TCU küldi, inverter engedélyezõ jel, azt küldi amit CAN-rõl beolvasott\nDerating : valamilyen derating állapotban van"
  # "Wi-Fi"
  # "CAN-USB"
  # "Log Analysis"
  # "TPS1"
  # "STA1"
  # "TPS2"
  # "STA1"
  # "STA2"
  # "STA2"
  # "BPS1"
  # "Throttle Bias"
  # "STA1 raw"
  # "BPS2"
  # "BPF"
  # "Regen Bias"
  # "STA2 raw"
  # "BPR"
  # "InverterOn"
  # "InverterOn"
  # "InverterOn"
  # "InverterOn"
  # "DcOn"
  # "DcOn"
  # "DcOn"
  # "DcOn"
  # "Enable"
  # "Enable"
  # "Enable"
  # "Enable"
  # "ErrorReset"
  # "ErrorReset"
  # "ErrorReset"
  # "ErrorReset"
  # "SysReady"
  # "SysReady"
  # "SysReady"
  # "SysReady"
  # "Error"
  # "Error"
  # "Error"
  # "Error"
  # "Warn"
  # "Warn"
  # "Warn"
  # "Warn"
  # "QuitDcOn"
  # "QuitDcOn"
  # "QuitDcOn"
  # "QuitDcOn"
  # "DcOn"
  # "DcOn"
  # "DcOn"
  # "DcOn"
  # "QuitInvOn"
  # "QuitInvOn"
  # "QuitInvOn"
  # "QuitInvOn"
  # "InverterOn"
  # "InverterOn"
  # "InverterOn"
  # "InverterOn"
  # "Derating"
  # "Derating"
  # "Derating"
  # "Derating"
  # "HV Accumulator ECU"
  # "Pedalbox"
  # "LV Sys ECU"
  # "MCU Power ECU"
  # "MCU Support ECU"
  # "Dashboard"
  # "APPS Error"
  # "BPPS Error"
  # "Steering Error"
  # "HV Accumulator Error"
  # "Rotary Switch Error"
  # "MCU Error"
  # "Button Error"
  # "Noheartbeat Error"
  # "FR AMK Error"
  # "RL AMK Error"
  # "FL AMK Error"
  # "RR AMK Error"
  # "Sensorbox Error"
  # "LV Accumulator Error"
  # "Brake Pressure Error"
  # "Yaw Control"
  # "Powerlimiter"
  # "Characteristics Approx"
  # "Smooth Transition"
  # "ASSI State"
  # "EBS State"
  # "AMI State"
types:
  T1 = cluster{"Cluster":cluster{"Col":dbl, "X":dbl, "Y":dbl}}[]
  T2 = cluster{"IGBT FL TEMP":i16, "IGBT FR TEMP":dbl, "IGBT RL TEMP":dbl, "IGBT RR TEMP":dbl}
  T3 = enum32{"Config", "Raw Data", "Driver", "TCU", "MCUs", "SC", "LV Accu", "HV Accu", "Dynamics", "Tractive System", "Temperatures", "LV System", "Errors", "Test Settings", "AS", "Lap"}
  T4 = cluster{"[0]":u16, "[1]":u16, "[2]":u16, "[3]":u16, "[4]":u16, "[5]":u16, "[6]":u16, "[7]":u16, "[8]":u16}
  T5 = cluster{"Velocity [km/h]":dbl, "Torque":dbl, dbl, dbl}
  T6 = cluster{"Actual Velocity (RPM)":i16, "Actual Velocity (RPM) 2":i16, "Actual Velocity (RPM) 3":i16, "Actual Velocity (RPM) 4":i16}
  T7 = cluster{"BP_front":i16, "BP_rear":i16, "Brake_Threshold":u8, "TC_Param":u8}
  T8 = enum16{"Invalid", "Off", "Ready", "Driving", "Emergency brake", "Finish", ""}
  T9 = enum16{"Invalid", "Unavailable", "Armed", "Triggered", ""}
  T10 = enum16{"Invalid", "Acceleration", "Skidpad", "Trackdrive", "Braketest", "Inspection", ""}
  T11 = cluster{ext, "Steering Angle":dbl, "Actual pos [°] Maxon":ext}
  T12 = cluster{"SoC":i32, "MotorTemp_FL":dbl, "MotorTemp_FR":dbl, "MotorTemp_RL":dbl, "MotorTemp_RR":dbl, "InverterTemp_FL":dbl, "InverterTemp_FR":dbl, "InverterTemp_RL":dbl, "InverterTemp_RR":dbl, "Laptime":timestamp, "Lap":i32, "Curr Abs Avg":dbl}[]
  T13 = typedef "ncNetAttr.ctl" = cluster{"Start On Open":enum32{"FALSE", "TRUE"}, "Baud Rate":u32, "Read Queue Length":u32, "Write Queue Length":u32, "Standard Comparator":u32, "Standard Mask":u32, "Extended Comparator":u32, "Extended Mask":u32}
  T14 = typedef "xobjhandle.ctl" = u32
  T15 = typedef "XNET Frame CAN.ctl" = cluster{"timestamp":timestamp, "payload":u8[], "identifier":u32, "type":T16, "extended?":bool, "echo?":bool}
  T16 = typedef "XNET Frame Type CAN.ctl" = u8
  T17 = cluster{"ConeType":cluster{"Col":dbl, "X":dbl, "Y":dbl}}[]
  T18 = cluster{"Actual Velocity\nFL [RPM]":i16, "Actual Velocity\nFR [RPM]":i16, "Actual Velocity\nRL [RPM]":i16, "Actual Velocity \nRR [RPM]":i16}
  T19 = cluster{"T Motor FL [°C]":dbl, "T Motor FR [°C]":dbl, "T Motor RL [°C]":dbl, "T Motor RR [°C]":dbl}
  T20 = cluster{"T Inv. FL [°C]":dbl, "T Inv. FR [°C]":dbl, "T Inv. RL [°C]":dbl, "T Inv. RR [°C]":dbl}
  T21 = typedef "XDNodeRunTimeDep.lvlib/timing_clust.ctl" = cluster{"Expected End [f-1]":u64, "Actual End [f-1]":u64, "Finished Late? [f-1]":bool, "Expected End [i-1]":u64, "Actual End [i-1]":u64, "Finished Late? [i-1]":bool, "Expected Start [i]":u64, "Actual Start [i]":u64, "Expected Start [f]":u64, "Actual Start [f]":u64, "Source Name":string, "Structure Name":string, "Period":i64, "Deadline":i64, "Offset":i64, "Start":i64, "Priority":i32, "Timeout":i32, "Mode":T22, "Wakeup Reason":T23, "Error":errorcluster, "Source Type":string, "Secondary Source Type":string, "Global End Time":u64, "Global Start Time":u64, "Frame Duration":u64, "Iteration Duration":u64, "Assigned CPU":i32, "I/O Scan Engine Mode":u32}
  T22 = typedef "XDNodeRunTimeDep.lvlib/nitl_modes.ctl" = enum32{"No Change", "Process missed periods, maintain original phase", "Discard missed periods, maintain original phase", "Process missed periods, ignore original phase", "Discard missed periods, ignore original phase"}
  T23 = typedef "XDNodeRunTimeDep.lvlib/wakeup.ctl" = enum32{"Normal", "Aborted", "Asynchronous wakeup", "Timing source error", "Timed loop error", "Timeout"}
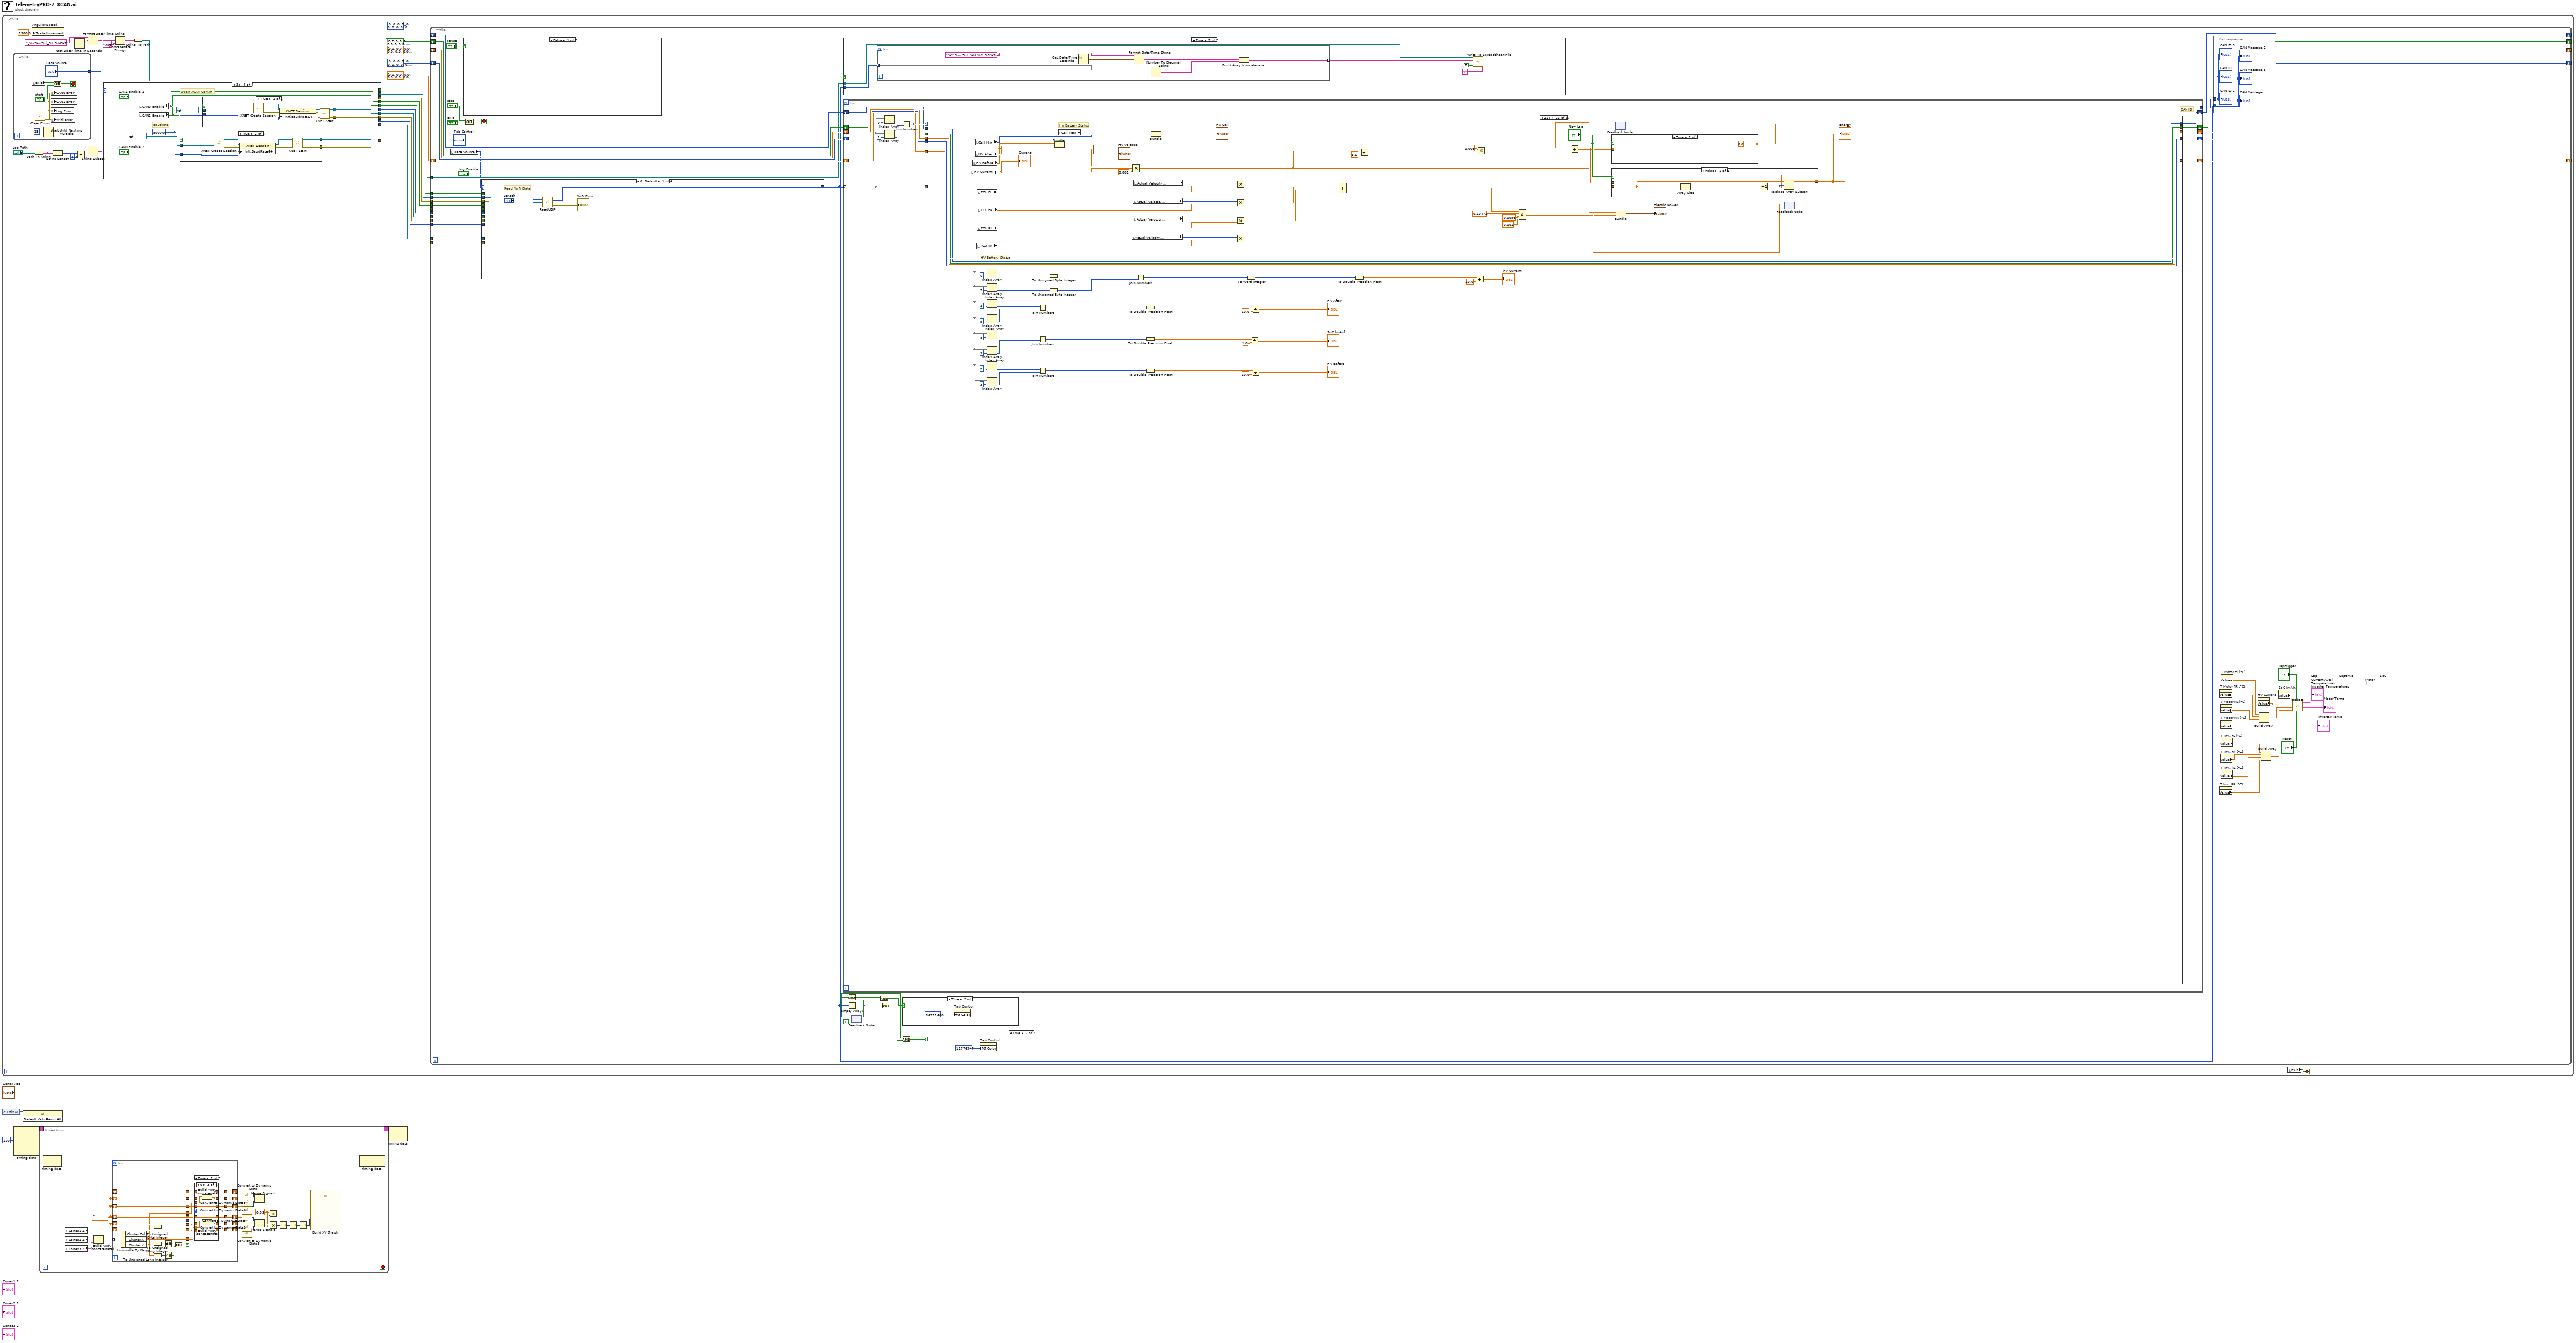
[diagram p0: block diagram]
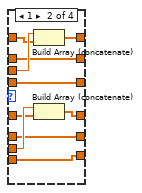
[diagram p4: hidden frame]
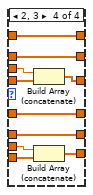
[diagram p5: hidden frame]
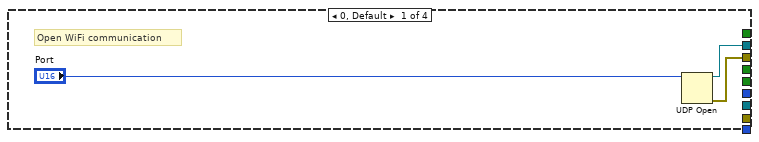
[diagram p6: hidden frame]
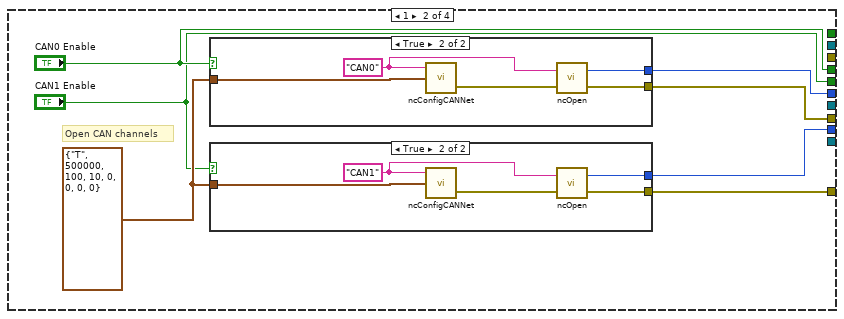
[diagram p7: hidden frame]
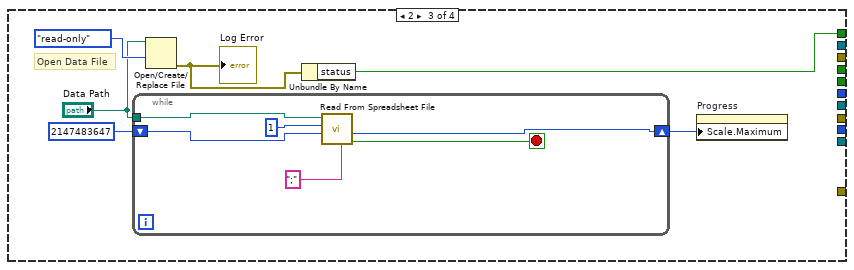
[diagram p10: hidden frame]
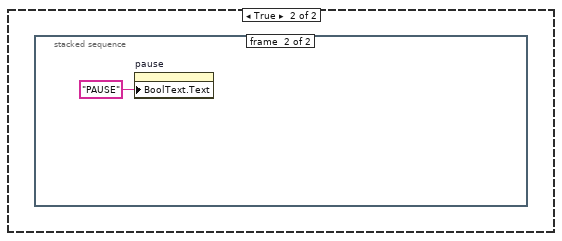
[diagram p13: hidden frame]
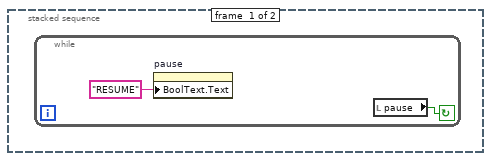
[diagram p14: hidden frame]
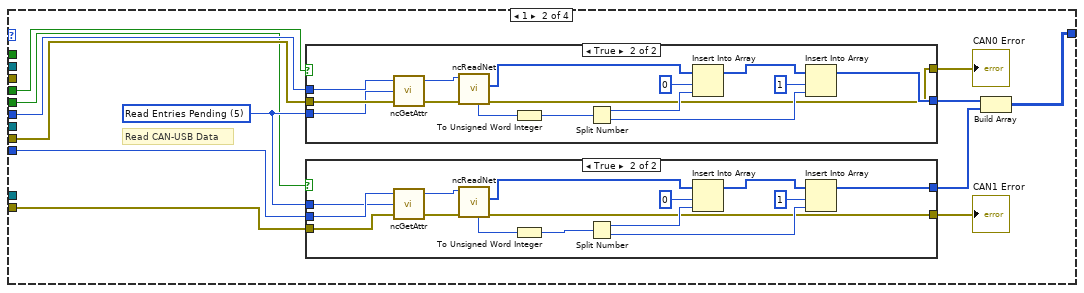
[diagram p17: hidden frame]
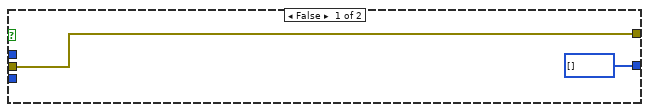
[diagram p18: hidden frame]
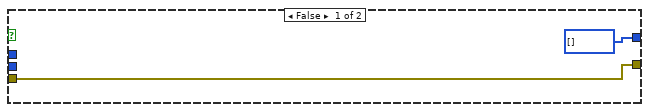
[diagram p19: hidden frame]
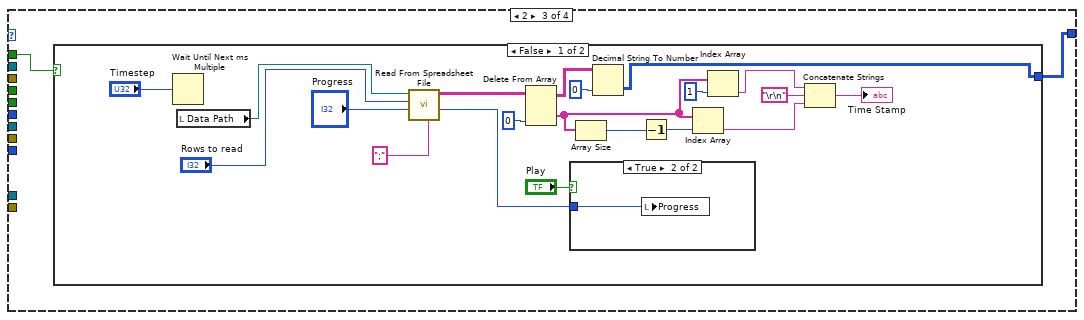
[diagram p20: hidden frame]
diagram:
  n1 = while {
    stop <- w8 stop-if-true
    n2 = while {
      tunnel: ["Data Source"] -> w9
      stop <- w37 stop-if-true
      n3 = local read "Exit"() -> (w38:bool)
      n4 = call <vilib>:"Clear Errors.vi"() -> ("error out"=w36:errorcluster)  [unwired: 6 in, 1 out]
      n5 = Wait Until Next ms Multiple(millisecond multiple=u32 25) -> ()  [unwired: 1 out]
      n6 = local write "CAN0 Error"(w36) -> ()
      n7 = local write "CAN1 Error"(w36) -> ()
      n8 = local write "Log Error"(w36) -> ()
      n9 = local write "WiFi Error"(w36) -> ()
      n10 = Compound Arithmetic op=OR(w38, "start") -> (w37:bool)
    }
    n11 = property on="Angular Speed" class="WFChart (strict)"("YScale.Increment"=1500.0 ("Y Scale.Range:Increment")) -> ()  [unwired: 2 in, 2 out]
    n12 = Path To String(path="Log Path") -> (string=w27:string)
    n13 = String Length(string=w27) -> (length=w26:i32)
    n14 = Get Date/Time In Seconds() -> (seconds since 1Jan1904=w29:timestamp)
    n15 = Subtract(x=w26, y=4) -> (x-y=w24:i32)
    n16 = Format Date/Time String(time format string (%c)="_%Y%m%d_%H%M%S", seconds (now)=w29) -> (date/time string=w20:string)  [unwired: 1 in]
    n17 = String Subset(string=w27, length (rest)=w24) -> (substring=w21:string)  [unwired: 1 in]
    n18 = case shown="3" w9 {
      tunnel: [_ w51 _ _] -> w13
      tunnel: [_ w50 _ w76] -> w14
      tunnel: [_ w49 _ _] -> w16
      tunnel: [_ w48 _ w75] -> w15
      tunnel: [w43 _ _ _] -> w18
      tunnel: [w42 _ _ _] -> w17
      tunnel: [_ "CAN0 Enable" _ w80] -> w12
      tunnel: [_ "CAN1 Enable" _ w79] -> w11
      tunnel: [_ _ w65 _] -> w10
      tunnel: [_ _ _ w78] -> w6
      tunnel: [_ _ _ w77] -> w5
      frame 0, Default {
        # "Open WiFi communication"
        n19 = UDP Open(11:"Port") -> (port=w43:refnum<k16>, 0:w42:errorcluster)  [unwired: 4 in, 1 out]
      }
      frame 1 {
        w47 = T13 {"Start On Open"=enum."TRUE", "Baud Rate"=500000, "Read Queue Length"=100, "Write Queue Length"=10, "Standard Comparator"=0, "Standard Mask"=0, "Extended Comparator"=0, "Extended Mask"=0} ("CAN Network Interface Config")
        # "Open CAN channels"
        n20 = case shown="True" "CAN0 Enable" {
          tunnel: w47 -> [_ w59]
          tunnel: [_ w58] -> w51
          tunnel: [_ w57] -> w50
          frame False {
          }
          frame True {
            w60 = "CAN0" ("ObjName")
            n21 = call <vilib>:"ncConfigCANNet.vi"("CAN Network Interface Config"=w59, "ObjName"=w60) -> ("Error out"=w61:errorcluster)  [unwired: 3 in]
            n22 = call <vilib>:"ncOpen.vi"("Error in"=w61, "ObjName"=w60) -> ("Error out"=w57:errorcluster, "ObjHandle out"=w58:T14)
          }
        }
        n23 = case shown="True" "CAN1 Enable" {
          tunnel: [_ w54] -> w49
          tunnel: [_ w53] -> w48
          tunnel: w47 -> [_ w52]
          frame False {
          }
          frame True {
            w56 = "CAN1" ("ObjName")
            n24 = call <vilib>:"ncConfigCANNet.vi"("CAN Network Interface Config"=w52, "ObjName"=w56) -> ("Error out"=w55:errorcluster)  [unwired: 3 in]
            n25 = call <vilib>:"ncOpen.vi"("Error in"=w55, "ObjName"=w56) -> ("Error out"=w53:errorcluster, "ObjHandle out"=w54:T14)
          }
        }
      }
      frame 2 {
        # "Open Data File"
        n26 = while {
          tunnel: "Data Path" -> [w73]
          shift-right: [w69] -> w63
          shift-left: 2147483647 ("mark after read (chars.)") -> [w70]
          stop <- w71 stop-if-true
          n27 = call-poly <vilib>:"Read From Spreadsheet File.vi"("delimiter (\\t)"=";" ("delimiter (\\t)"), "start of read offset (chars.:0)"=w70, "number of rows (all:-1)"=1, "file path (dialog if empty)"=w73) -> ("EOF?"=w71:bool, "mark after read (chars.)"=w69:i32)  [unwired: 3 in, 3 out]
        }
        n28 = Open/Create/Replace File(file path (use dialog)="Data Path", access (0:read/write)=enum16{"read/write", "read-only", "write-only"}."read-only") -> (error out=w66:errorcluster)  [unwired: 4 in, 2 out]
        "Log Error" <- w66
        n29 = Unbundle By Name(w66) -> ("status"=w65:bool)
        n30 = property on="Progress" class="Slide (strict)"("Scale.Maximum"=w63) -> ()  [unwired: 2 in, 2 out]
      }
      frame 3 {
        w74 = 500000
        # "Open XCAN Comm"
        # "Baudrate"
        n31 = local read "CAN0 Enable"() -> (w80:bool)
        n32 = local read "CAN1 Enable"() -> (w79:bool)
        n33 = case shown="True" w79 {
          tunnel: refnum<k21> "CAN3" ("XNET Interface") -> [_ w90]
          tunnel: w74 -> [_ w89]
          tunnel: [_ w84] -> w75
          tunnel: [_ w83] -> w77
          frame False {
          }
          frame True {
            n34 = call-poly <vilib>:"XNET Create Session.vi"("interface"=w90) -> ("session out"=w88:refnum<k21>, "error out"=w87:errorcluster)  [unwired: 13 in]
            n35 = property class="XNET Session"(reference=w88, error in=w87, "Intf.BaudRate64"=w89) -> (reference out=w86:refnum<k21>, error out=w85:errorcluster)
            n36 = call <vilib>:"XNET Start.vi"("session in"=w86, "error in (no error)"=w85) -> ("session out"=w83:refnum<k21>, "error out"=w84:errorcluster)  [unwired: 12 in]
          }
        }
        n37 = case shown="True" w80 {
          tunnel: w74 -> [_ w98]
          tunnel: refnum<k21> "CAN2" ("XNET Interface") -> [_ w97]
          tunnel: [_ w92] -> w76
          tunnel: [_ w91] -> w78
          frame False {
          }
          frame True {
            n38 = call-poly <vilib>:"XNET Create Session.vi"("interface"=w97) -> ("session out"=w95:refnum<k21>, "error out"=w96:errorcluster)  [unwired: 13 in]
            n39 = property class="XNET Session"(reference=w95, error in=w96, "Intf.BaudRate64"=w98) -> (reference out=w94:refnum<k21>, error out=w93:errorcluster)
            n40 = call <vilib>:"XNET Start.vi"("session in"=w94, "error in (no error)"=w93) -> ("session out"=w91:refnum<k21>, "error out"=w92:errorcluster)  [unwired: 12 in]
          }
        }
      }
    }
    n41 = Concatenate Strings(w21, w20, ".txt" ("string")) -> (w22:string)
    n42 = String To Path(string=w22) -> (path=w30:path)
    n43 = while {
      tunnel: w18 -> [w151]
      tunnel: w17 -> [w152]
      shift-right: [w149] -> _
      shift-left: u16[] [0, 0, 0, 0, 0, 0, 0, 0, 0, 0, 0, 0, 0, 0, 0, 0, 0, 0, 0, 0, 0, 0, 0, 0, 0, 0, 0, 0, 0, 0, 0, 0, 0, 0, 0, 0, 0, 0, 0, 0, 0, 0, 0, 0, 0, 0, 0, 0, 0, 0, 0, 0, 0, 0, 0, 0, 0, 0, 0, 0, 0, 0, 0, 0, 0, 0, 0, 0, 0, 0, 0, 0, 0, 0, 0, 0, 0, 0, 0, 0, 0, 0, 0, 0, 0, 0, 0, 0, 0, 0, 0, 0, 0, 0, 0, 0, 0, 0, 0, 0, 0, 0, 0, 0, 0, 0, 0, 0, 0, 0, 0, 0, 0, 0, 0, 0, 0, 0, 0, 0, 0, 0, 0, 0, 0, 0, 0, 0, 0, 0, 0, 0, 0, 0, 0, 0, 0, 0, 0, 0, 0, 0, 0, 0, 0, 0, 0, 0, 0, 0, 0, 0, 0, 0, 0, 0, 0, 0, 0, 0, 0, 0, 0, 0, 0, 0, 0, 0, 0, 0, 0, 0, 0, 0, 0, 0, 0, 0, 0, 0, 0] -> [w150]
      shift-right: [w148] -> _
      shift-left: dbl[] [0.0, 0.0, 0.0, 0.0, 0.0, 0.0, 0.0, 0.0, 0.0, 0.0, 0.0, 0.0, 0.0, 0.0, 0.0, 0.0, 0.0, 0.0, 0.0, 0.0, 0.0, 0.0, 0.0, 0.0, 0.0, 0.0, 0.0, 0.0, 0.0, 0.0, 0.0, 0.0, 0.0, 0.0, 0.0, 0.0, 0.0, 0.0, 0.0, 0.0, 0.0, 0.0, 0.0, 0.0, 0.0, 0.0, 0.0, 0.0, 0.0, 0.0, 0.0, 0.0, 0.0, 0.0, 0.0, 0.0, 0.0, 0.0, 0.0, 0.0, 0.0, 0.0, 0.0, 0.0, 0.0, 0.0, 0.0, 0.0, 0.0, 0.0, 0.0, 0.0, 0.0, 0.0, 0.0, 0.0, 0.0, 0.0, 0.0, 0.0, 0.0, 0.0, 0.0, 0.0, 0.0, 0.0, 0.0, 0.0, 0.0, 0.0, 0.0, 0.0, 0.0, 0.0, 0.0, 0.0, 0.0, 0.0, 0.0, 0.0, 0.0, 0.0, 0.0, 0.0, 0.0, 0.0, 0.0, 0.0, 0.0, 0.0, 0.0, 0.0, 0.0, 0.0, 0.0, 0.0, 0.0, 0.0, 0.0, 0.0, 0.0, 0.0, 0.0, 0.0, 0.0, 0.0, 0.0, 0.0, 0.0, 0.0, 0.0, 0.0, 0.0, 0.0, 0.0, 0.0, 0.0, 0.0, 0.0, 0.0, 0.0, 0.0, 0.0, 0.0, 0.0, 0.0, 0.0, 0.0, 0.0, 0.0, 0.0, 0.0, 0.0, 0.0, 0.0, 0.0, 0.0, 0.0, 0.0, 0.0, 0.0, 0.0, 0.0, 0.0, 0.0, 0.0, 0.0, 0.0, 0.0, 0.0, 0.0, 0.0, 0.0, 0.0, 0.0, 0.0, 0.0, 0.0, 0.0, 0.0, 0.0] -> [w147]
      shift-right: [w143] -> _
      shift-left: u16[] [0, 0, 0, 0, 0, 0, 0, 0, 0, 0, 0, 0, 0, 0] -> [w144]
      shift-right: [w142] -> _
      shift-left: bool[] [FALSE, FALSE, FALSE, FALSE, FALSE, FALSE, FALSE, FALSE, FALSE, FALSE, FALSE, FALSE, FALSE, FALSE] -> [w145]
      shift-right: [w141] -> _
      shift-left: dbl[] [0.0, 0.0, 0.0, 0.0, 0.0, 0.0, 0.0, 0.0, 0.0, 0.0, 0.0, 0.0, 0.0, 0.0] -> [w146]
      tunnel: w30 -> [w138]
      tunnel: w16 -> [w136]
      tunnel: w15 -> [w135]
      tunnel: w14 -> [w134]
      tunnel: w13 -> [w133]
      tunnel: w12 -> [w118]
      tunnel: w11 -> [w132]
      tunnel: w10 -> [w124]
      tunnel: w6 -> [w117]
      tunnel: w5 -> [w116]
      stop <- w120 stop-if-true
      n44 = local read "Data Source"() -> (w137:u16)
      n45 = case shown="False" "pause" {
        frame False {
        }
        frame True {
          n46 = stacked-sequence {
            frame #0 {
              n47 = while {
                stop <- w154 continue-if-true
                n48 = property on="pause" class="Bool (strict)"("BoolText.Text"="RESUME" ("Boolean Text.Text")) -> ()  [unwired: 2 in, 2 out]
                n49 = local read "pause"() -> (w154:bool)
              }
            }
            frame #1 {
              n50 = property on="pause" class="Bool (strict)"("BoolText.Text"="PAUSE" ("Boolean Text.Text")) -> ()  [unwired: 2 in, 2 out]
            }
          }
        }
      }
      n51 = Compound Arithmetic op=OR("stop", "Exit") -> (w120:bool)
      n52 = case shown="0, Default" w137 {
        tunnel: w152 -> [w160 _ _ _]
        tunnel: w151 -> [w161 _ _ _]
        tunnel: [w159 w169 w210 w235] -> w131
        tunnel: w136 -> [_ w174 _ _]
        tunnel: w135 -> [_ w167 _ w239]
        tunnel: w134 -> [_ w173 _ w238]
        tunnel: w133 -> [_ w172 _ _]
        tunnel: w118 -> [_ w164 _ w241]
        tunnel: w132 -> [_ w163 _ w240]
        tunnel: w124 -> [_ _ w209 _]
        tunnel: w117 -> [_ _ _ w237]
        tunnel: w116 -> [_ _ _ w236]
        frame 0, Default {
          # "Read WiFi Data"
          n53 = call "ReadUDP.vi"("error in (no error)"=w160, "connection ID"=w161, "Message length"="Length") -> ("error out"=→"WiFi Error":errorcluster, "Array"=w159:u8[][])
        }
        frame 1 {
          w166 = u32 5 items=["(reserved)", "Protocol Version", "Software Version", "Object State", "(reserved)", "Read Entries Pending", "Write Entries Pending", "ReadMult Size for Notification", "Listen Only?", "Self Reception?", "Transmit Error Counter", "Receive Error Counter", "Single Shot Transmit?", "Series 2 Filter Mode", "Series 2 Mask", "Series 2 Comparator", "Serial Number", "Form Factor", "Series", "Transceiver Type", "Interface Number", "Series 2 Error/Arb Capture", "Transceiver Mode", "Transceiver External Outputs", "Transceiver External Inputs", "Start Trigger Behavior", "Log Comm Warnings", "User RTSI Frame", "Transmit Mode", "Log Start Trigger?", "Timestamp Format", "Master Timebase Rate", "Virtual Bus Timing", "Write Entries Free", "Timeline Recovery", "Log Bus Errors", "Log Transceiver Faults", "Termination", "LIN Sleep", "LIN Checksum Type", "LIN Response Timeout", "LIN Enable DLC Check", "LIN Log Wakeup", "Baud Rate"] ("AttrId")
          # "Read CAN-USB Data"
          n54 = case shown="True" w164 {
            tunnel: w166 -> [_ w177]
            tunnel: w173 -> [w176 w190]
            tunnel: w172 -> [_ w178]
            tunnel: [u8[] [] ("Data") w180] -> w171
            tunnel: [w176 w179] -> w165
            frame False {
            }
            frame True {
              n55 = call <vilib>:"ncGetAttr.vi"("Error in"=w190, "AttrId"=w177, "ObjHandle in"=w178) -> ("Error out"=w189:errorcluster, "ObjHandle out"=w191:T14)  [unwired: 1 out]
              n56 = call <vilib>:"ncReadNet.vi"("ObjHandle in"=w191, "Error in"=w189) -> ("ArbitrationId"=w182:u32, "Data"=w188:u8[], "Error out"=w179:errorcluster)  [unwired: 2 in, 4 out]
              n57 = To Unsigned Word Integer(number=w182) -> (unsigned 16bit integer=w181:u16)
              n58 = Split Number(x=w181) -> (hi(x)=w184:u8, lo(x)=w183:u8)
              n59 = Insert Into Array(array=w188, index=0, new element=w184) -> (w186:u8[])
              n60 = Insert Into Array(array=w186, index=1, new element=w183) -> (w180:u8[])
            }
          }
          "CAN0 Error" <- w165
          n61 = case shown="True" w163 {
            tunnel: w174 -> [_ w207]
            tunnel: w166 -> [_ w206]
            tunnel: [u8[] [] ("Data") w196] -> w170
            tunnel: [w193 w195] -> w168
            tunnel: w167 -> [w193 w194]
            frame False {
            }
            frame True {
              n62 = call <vilib>:"ncGetAttr.vi"("Error in"=w194, "AttrId"=w206, "ObjHandle in"=w207) -> ("Error out"=w205:errorcluster, "ObjHandle out"=w208:T14)  [unwired: 1 out]
              n63 = call <vilib>:"ncReadNet.vi"("ObjHandle in"=w208, "Error in"=w205) -> ("ArbitrationId"=w204:u32, "Data"=w200:u8[], "Error out"=w195:errorcluster)  [unwired: 2 in, 4 out]
              n64 = To Unsigned Word Integer(number=w204) -> (unsigned 16bit integer=w203:u16)
              n65 = Split Number(x=w203) -> (hi(x)=w199:u8, lo(x)=w197:u8)
              n66 = Insert Into Array(array=w200, index=0, new element=w199) -> (w198:u8[])
              n67 = Insert Into Array(array=w198, index=1, new element=w197) -> (w196:u8[])
            }
          }
          "CAN1 Error" <- w168
          n68 = Build Array(w171, w170) -> (w169:u8[][])
        }
        frame 2 {
          n69 = case shown="False" w209 {
            tunnel: [w224 u8[][] []] -> w210
            frame False {
              n70 = Wait Until Next ms Multiple(millisecond multiple="Timestep") -> ()  [unwired: 1 out]
              n71 = local read "Data Path"() -> (w230:path)
              n72 = call-poly <vilib>:"Read From Spreadsheet File.vi"("delimiter (\\t)"=";" ("delimiter (\\t)"), "start of read offset (chars.:0)"="Progress", "number of rows (all:-1)"="Rows to read", "file path (dialog if empty)"=w230) -> ("mark after read (chars.)"=w221:i32, "all rows"=w228:string[][])  [unwired: 3 in, 3 out]
              n73 = Delete From Array(array=w228, index (col)=0 ("disabled index (col)")) -> (deleted portion=w215:string[], array with subset deleted=w226:string[][])  [unwired: 2 in]
              n74 = case shown="True" "Play" {
                tunnel: w221 -> [_ w231]
                frame False {
                }
                frame True {
                  n75 = local write "Progress"(w231) -> ()
                }
              }
              n76 = Array Size(array=w215) -> (size(s)=w217:i32)
              n77 = Decimal String To Number(string=w226, default (0L)=u8 0 ("default (0 I32)")) -> (number=w224:u8[][])  [unwired: 1 in, 1 out]
              n78 = Decrement(x=w217) -> (x-1=w216:i32)
              n79 = Index Array(array=w215, index=w216) -> (element=w212:string)
              n80 = Index Array(array=w215, index=1) -> (element=w214:string)
              n81 = Concatenate Strings(w214, "\r\n", w212) -> (→"Time Stamp":string)
            }
            frame True {
            }
          }
        }
        frame 3 {
          n82 = case shown="True" w241 {
            tunnel: w237 -> [_ w277]
            tunnel: w238 -> [w262 w276]
            tunnel: [u8[] [] ("Data") w264] -> w243
            tunnel: [w262 w263] -> w234
            frame False {
            }
            frame True {
              n83 = call-poly <vilib>:"XNET Read.vi"("session in"=w277, "number to read (-1)"=1, "error in (no error)"=w276) -> ("data"=w274:T15[], "error out"=w263:errorcluster)  [unwired: 9 in, 2 out]
              n84 = Index Array(array=w274) -> (element=w273:T15)  [unwired: 1 in]
              n85 = Unbundle By Name(w273) -> ("identifier"=w272:u32, "payload"=w270:u8[])
              n86 = To Unsigned Word Integer(number=w272) -> (unsigned 16bit integer=w271:u16)
              n87 = Split Number(x=w271) -> (hi(x)=w268:u8, lo(x)=w266:u8)
              n88 = Insert Into Array(array=w270, index=0, new element=w268) -> (w267:u8[])
              n89 = Insert Into Array(array=w267, index=1, new element=w266) -> (w264:u8[])
            }
          }
          n90 = case shown="True" w240 {
            tunnel: w239 -> [w245 w259]
            tunnel: w236 -> [_ w260]
            tunnel: [w245 w257] -> w233
            tunnel: [u8[] [] ("Data") w246] -> w242
            frame False {
            }
            frame True {
              n91 = call-poly <vilib>:"XNET Read.vi"("session in"=w260, "number to read (-1)"=1, "error in (no error)"=w259) -> ("data"=w256:T15[], "error out"=w257:errorcluster)  [unwired: 9 in, 2 out]
              n92 = Index Array(array=w256) -> (element=w255:T15)  [unwired: 1 in]
              n93 = Unbundle By Name(w255) -> ("payload"=w254:u8[], "identifier"=w252:u32)
              n94 = To Unsigned Word Integer(number=w252) -> (unsigned 16bit integer=w251:u16)
              n95 = Split Number(x=w251) -> (hi(x)=w250:u8, lo(x)=w249:u8)
              n96 = Insert Into Array(array=w254, index=0, new element=w250) -> (w253:u8[])
              n97 = Insert Into Array(array=w253, index=1, new element=w249) -> (w246:u8[])
            }
          }
          n98 = local write "CAN0 Error"(w234) -> ()
          n99 = Build Array(w243, w242) -> (w235:u8[][])
          n100 = local write "CAN1 Error"(w233) -> ()
        }
      }
      n101 = case shown="True" "Log Enable" {
        tunnel: w138 -> [_ w281]
        tunnel: w131 -> [_ w280]
        frame False {
        }
        frame True {
          n102 = for {
            tunnel: w280 -> [w288] mode=indexing
            tunnel: [w286] -> w279 mode=indexing
            n103 = Get Date/Time In Seconds() -> (seconds since 1Jan1904=w284:timestamp)
            n104 = Format Date/Time String(time format string (%c)="%Y.%m.%d. %H:%M:%S%3u", seconds (now)=w284) -> (date/time string=w287:string)  [unwired: 1 in]
            n105 = Number To Decimal String(number=w288) -> (decimal integer string=w285:string[])  [unwired: 1 in]
            n106 = Build Array (concatenate)(w287, w285) -> (w286:string[])
          }
          n107 = call-poly <vilib>:"Write To Spreadsheet File.vi"("delimiter (\\t)"=";" ("delimiter (\\t)"), "append to file? (new file:F)"=TRUE, "2D data"=w279, "file path (dialog if empty)"=w281) -> ()  [unwired: 4 in, 1 out]
        }
      }
      n108 = for {
        tunnel: w131 -> [w301] mode=indexing
        tunnel: [w302] -> w140 mode=indexing
        shift-right: [w292] -> w149
        shift-left: w150 -> [w300]
        shift-right: [w298] -> w148
        shift-left: w147 -> [w299]
        shift-right: [w296] -> w143
        shift-left: w144 -> [w297]
        shift-right: [w291] -> w142
        shift-left: w145 -> [w295]
        shift-right: [w293] -> w141
        shift-left: w146 -> [w294]
        # "CAN ID"
        n109 = Index Array(array=w301, index=0) -> (element=w304:u8)
        n110 = Index Array(array=w301, index=1) -> (element=w303:u8)
        n111 = Join Numbers(hi=w304, lo=w303) -> ((hi.lo)=w302:u16)
        n112 = case shown="214" w302 {
          tunnel: w301 -> [_ w317 w418 w518 w645 w699 w748 w769 w796 w827 w858 w903 w932 w1053 w1075 w1082 w1193 w1262 w1292 w1369 w1449 w1502 w1594 w1624 w1671 w1705 w1748 w1777 w1811 w1892 w1958 w1993 w2064 w2073 w2084 w2145 w2162 w2181 w2249 w2355 w2389 w2400 w2488 w2576 w2642 w2678 w2702 w2720 w2744 w2799 w2855 w2878 w2919 w2926 w2930 w2956 w2973 w3007 w3155 w3173 w3278 w3393 w3487 w3515 w3539 w3566 w3587]
          tunnel: w300 -> [w311 w312 w413 w513 w652 w706 w755 w784 w815 w846 w877 w910 w939 w1060 w1077 w1109 w1224 w1279 w1306 w1373 w1464 w1546 w1613 w1660 w1700 w1736 w1771 w1806 w1842 w1923 w1987 w2022 w2063 w2075 w2080 w2141 w2171 w2227 w2336 w2379 w2387 w2454 w2504 w2622 w2672 w2695 w2703 w2721 w2745 w2812 w2864 w2895 w2914 w2922 w2953 w2965 w2974 w3046 w3164 w3258 w3334 w3482 w3502 w3521 w3556 w3561 w3580]
          tunnel: [w311 w312 w413 w513 w652 w706 w755 w784 w815 w846 w877 w910 w939 w1060 w1077 w1109 w1224 w1279 w1306 w1343 w1464 w1546 w1613 w1660 w1700 w1736 w1771 w1806 w1842 w1923 w1987 w2022 w2063 w2075 w2080 w2141 w2171 w2227 w2336 w2379 w2387 w2454 w2504 w2622 w2672 w2695 w2703 w2721 w2745 w2812 w2864 w2895 w2914 w2922 w2953 w2965 w2974 w3046 w3164 w3258 w3334 w3482 w3502 w3521 w3556 w3561 w3580] -> w292
          tunnel: w299 -> [w310 w316 w412 w512 w651 w705 w754 w783 w814 w845 w876 w909 w938 w1059 w1076 w1108 w1223 w1278 w1305 w1366 w1463 w1545 w1617 w1664 w1699 w1735 w1770 w1805 w1841 w1922 w1986 w2021 w2062 w2074 w2079 w2140 w2175 w2226 w2340 w2383 w2388 w2457 w2503 w2621 w2668 w2699 w2715 w2725 w2749 w2816 w2868 w2888 w2913 w2921 w2952 w2969 w2978 w3050 w3168 w3262 w3337 w3486 w3506 w3520 w3555 w3565 w3579]
          tunnel: [w310 w316 w412 w512 w651 w705 w754 w783 w814 w845 w876 w909 w938 w1059 w1076 w1108 w1223 w1278 w1305 w1320 w1463 w1545 w1617 w1664 w1699 w1735 w1770 w1805 w1841 w1922 w1986 w2021 w2062 w2074 w2079 w2140 w2175 w2226 w2340 w2383 w2388 w2457 w2503 w2621 w2668 w2699 w2715 w2725 w2749 w2816 w2868 w2888 w2913 w2921 w2952 w2969 w2978 w3050 w3168 w3262 w3337 w3486 w3506 w3520 w3555 w3565 w3579] -> w298
          tunnel: w297 -> [w309 w315 w416 w516 w650 w704 w753 w782 w813 w844 w873 w908 w937 w1058 w1080 w1105 w1222 w1277 w1304 w1353 w1460 w1540 w1616 w1663 w1696 w1732 w1767 w1802 w1838 w1919 w1983 w2018 w2032 w2078 w2083 w2144 w2174 w2219 w2339 w2382 w2384 w2456 w2502 w2620 w2671 w2698 w2714 w2724 w2748 w2815 w2867 w2896 w2917 w2925 w2950 w2968 w2977 w3049 w3167 w3261 w3263 w3485 w3505 w3518 w3552 w3564 w3583]
          tunnel: [w309 w315 w416 w516 w650 w704 w753 w782 w813 w844 w873 w908 w937 w1058 w1080 w1105 w1222 w1277 w1304 w1353 w1460 w1540 w1616 w1663 w1696 w1732 w1767 w1802 w1838 w1919 w1983 w2018 w2032 w2078 w2083 w2144 w2174 w2219 w2339 w2382 w2384 w2456 w2502 w2620 w2671 w2698 w2714 w2724 w2748 w2815 w2867 w2880 w2917 w2925 w2950 w2968 w2977 w3049 w3167 w3261 w3263 w3485 w3505 w3518 w3552 w3564 w3583] -> w296
          tunnel: w295 -> [w308 w314 w415 w515 w649 w703 w752 w781 w812 w843 w872 w907 w936 w1057 w1079 w1106 w1221 w1276 w1303 w1351 w1461 w1539 w1615 w1662 w1697 w1733 w1768 w1803 w1839 w1920 w1984 w2019 w2031 w2077 w2082 w2143 w2173 w2218 w2338 w2381 w2385 w2455 w2501 w2619 w2670 w2697 w2713 w2723 w2747 w2814 w2866 w2892 w2916 w2924 w2949 w2967 w2976 w3048 w3166 w3260 w3336 w3484 w3504 w3517 w3553 w3563 w3582]
          tunnel: w294 -> [w307 w313 w414 w514 w648 w702 w751 w780 w811 w842 w871 w906 w935 w1056 w1078 w1107 w1220 w1275 w1302 w1352 w1462 w1544 w1614 w1661 w1698 w1734 w1769 w1804 w1840 w1921 w1985 w2020 w2061 w2076 w2081 w2142 w2172 w2225 w2337 w2380 w2386 w2453 w2500 w2618 w2669 w2696 w2712 w2722 w2746 w2813 w2865 w2889 w2915 w2923 w2951 w2966 w2975 w3047 w3165 w3259 w3335 w3483 w3503 w3519 w3554 w3562 w3581]
          tunnel: [w307 w313 w414 w514 w648 w702 w751 w780 w811 w842 w871 w906 w935 w1056 w1078 w1107 w1220 w1275 w1302 w1352 w1462 w1544 w1614 w1661 w1698 w1734 w1769 w1804 w1840 w1921 w1985 w2020 w2061 w2076 w2081 w2142 w2172 w2225 w2337 w2380 w2386 w2453 w2500 w2618 w2669 w2696 w2712 w2722 w2746 w2813 w2865 w2886 w2915 w2923 w2951 w2966 w2975 w3047 w3165 w3259 w3335 w3483 w3503 w3519 w3554 w3562 w3581] -> w293
          tunnel: [w308 w314 w415 w515 w649 w703 w752 w781 w812 w843 w872 w907 w936 w1057 w1079 w1106 w1221 w1276 w1303 w1351 w1461 w1539 w1615 w1662 w1697 w1733 w1768 w1803 w1839 w1920 w1984 w2019 w2031 w2077 w2082 w2143 w2173 w2218 w2338 w2381 w2385 w2455 w2501 w2619 w2670 w2697 w2713 w2723 w2747 w2814 w2866 w2890 w2916 w2924 w2949 w2967 w2976 w3048 w3166 w3260 w3336 w3484 w3504 w3517 w3553 w3563 w3582] -> w291
          frame 0, Default {
          }
          frame 272 {
            w405 = u64 511 ("y")
            w383 = -1.0 ("y")
            w370 = i16 -8 ("y")
            w369 = u64 511 ("y")
            w368 = u64 1023 ("y")
            w367 = u64 3 ("y")
            n113 = local read "ConeType"() -> (w344:cluster{"Col":dbl, "X":dbl, "Y":dbl})
            n114 = Array Subset(array=w317, index=2, length=8) -> (w347:u8[])
            n115 = Index Array(array=w347, index #1=7 ("index"), index #2=6 ("index"), index #3=5 ("index"), index #4=4 ("index"), index #5=3 ("index"), index #6=2 ("index"), index #7=1 ("index"), index #8=0 ("index")) -> (element #1=w326:u8, element #2=w327:u8, element #3=w328:u8, element #4=w329:u8, element #5=w330:u8, element #6=w331:u8, element #7=w332:u8, element #8=w333:u8)
            n116 = Join Numbers(hi=w326, lo=w327) -> ((hi.lo)=w334:u16)
            n117 = Join Numbers(hi=w328, lo=w329) -> ((hi.lo)=w335:u16)
            n118 = Join Numbers(hi=w330, lo=w331) -> ((hi.lo)=w336:u16)
            n119 = Join Numbers(hi=w332, lo=w333) -> ((hi.lo)=w337:u16)
            n120 = Join Numbers(hi=w334, lo=w335) -> ((hi.lo)=w338:u32)
            n121 = Join Numbers(hi=w336, lo=w337) -> ((hi.lo)=w339:u32)
            n122 = Join Numbers(hi=w338, lo=w339) -> ((hi.lo)=w348:u64)
            "(hi.lo)" <- w348
            n123 = Logical Shift(y=i16 0, x=w348) -> (x << y=w358:u64)
            n124 = Logical Shift(y=i16 -2, x=w348) -> (x << y=w359:u64)
            n125 = Logical Shift(y=i16 -12, x=w348) -> (x << y=w360:u64)
            n126 = Logical Shift(y=i16 -21, x=w348) -> (x << y=w361:u64)
            n127 = Logical Shift(y=i16 -23, x=w348) -> (x << y=w362:u64)
            n128 = Logical Shift(y=i16 -33, x=w348) -> (x << y=w363:u64)
            n129 = Logical Shift(y=i16 -42, x=w348) -> (x << y=w364:u64)
            n130 = Logical Shift(y=i16 -44, x=w348) -> (x << y=w365:u64)
            n131 = Logical Shift(y=i16 -54, x=w348) -> (x << y=w366:u64)
            n132 = And(x=w358, y=w367) -> (x .and. y?=w386:u64)
            n133 = And(x=w359, y=w368) -> (x .and. y?=w388:u64)
            n134 = And(x=w361, y=w367) -> (x .and. y?=w385:u64)
            n135 = And(x=w362, y=w368) -> (x .and. y?=w389:u64)
            n136 = And(x=w364, y=w367) -> (x .and. y?=w384:u64)
            n137 = And(x=w365, y=w368) -> (x .and. y?=w387:u64)
            n138 = And(x=w360, y=w369) -> (x .and. y?=w397:u64)
            n139 = And(x=w363, y=w369) -> (x .and. y?=w393:u64)
            n140 = And(x=w366, y=w369) -> (x .and. y?=w395:u64)
            n141 = Logical Shift(y=w370, x=w397) -> (x << y=w371:u64)
            n142 = Logical Shift(y=w370, x=w393) -> (x << y=w372:u64)
            n143 = Logical Shift(y=w370, x=w395) -> (x << y=w373:u64)
            n144 = To Unsigned Byte Integer(number=w386) -> (unsigned 8bit integer=w411:u8)
            n145 = To Unsigned Word Integer(number=w388) -> (unsigned 16bit integer=w410:u16)
            n146 = Decrement(x=w397) -> (x-1=w377:u64)
            n147 = To Unsigned Byte Integer(number=w385) -> (unsigned 8bit integer=w409:u8)
            n148 = To Unsigned Word Integer(number=w389) -> (unsigned 16bit integer=w408:u16)
            n149 = Decrement(x=w393) -> (x-1=w378:u64)
            n150 = To Unsigned Byte Integer(number=w384) -> (unsigned 8bit integer=w406:u8)
            n151 = To Unsigned Word Integer(number=w387) -> (unsigned 16bit integer=w407:u16)
            n152 = Decrement(x=w395) -> (x-1=w379:u64)
            n153 = Not(x=w377) -> (.not. x?=w400:u64)
            n154 = Not Equal To 0?(x=w371) -> (x != 0?=w375:bool)
            n155 = Not(x=w378) -> (.not. x?=w401:u64)
            n156 = Not Equal To 0?(x=w372) -> (x != 0?=w376:bool)
            n157 = Not(x=w379) -> (.not. x?=w403:u64)
            n158 = Not Equal To 0?(x=w373) -> (x != 0?=w374:bool)
            n159 = And(x=w405, y=w400) -> (x .and. y?=w399:u64)
            n160 = And(x=w405, y=w401) -> (x .and. y?=w402:u64)
            n161 = And(x=w405, y=w403) -> (x .and. y?=w404:u64)
            n162 = To Double Precision Float(number=w393) -> (double precision float=w394:dbl)
            n163 = Multiply(x=w383, y=w399) -> (x*y=w380:dbl)
            n164 = Multiply(x=w383, y=w402) -> (x*y=w382:dbl)
            n165 = Multiply(x=w383, y=w404) -> (x*y=w381:dbl)
            n166 = To Double Precision Float(number=w397) -> (double precision float=w398:dbl)
            n167 = To Double Precision Float(number=w395) -> (double precision float=w396:dbl)
            n168 = Select(t=w380, s=w375, f=w398) -> (s? t:f=w390:dbl)
            n169 = Select(t=w382, s=w376, f=w394) -> (s? t:f=w392:dbl)
            n170 = Select(t=w381, s=w374, f=w396) -> (s? t:f=w391:dbl)
            n171 = Bundle By Name(cluster=w344, "Col"=w411, "X"=w410, "Y"=w390) -> (w340:cluster{"Col":dbl, "X":dbl, "Y":dbl})
            n172 = Bundle By Name(cluster=w344, "Col"=w409, "X"=w408, "Y"=w392) -> (w341:cluster{"Col":dbl, "X":dbl, "Y":dbl})
            n173 = Bundle By Name(cluster=w344, "Col"=w406, "X"=w407, "Y"=w391) -> (w342:cluster{"Col":dbl, "X":dbl, "Y":dbl})
            n174 = Build Cluster Array(w340, w341, w342) -> (→"Cones1":T17)
          }
          frame 273 {
            w505 = u64 511 ("y")
            w483 = -1.0 ("y")
            w470 = i16 -8 ("y")
            w469 = u64 511 ("y")
            w468 = u64 1023 ("y")
            w467 = u64 3 ("y")
            n175 = local read "ConeType"() -> (w417:cluster{"Col":dbl, "X":dbl, "Y":dbl})
            n176 = Array Subset(array=w418, index=2, length=8) -> (w447:u8[])
            n177 = Index Array(array=w447, index #1=7 ("index"), index #2=6 ("index"), index #3=5 ("index"), index #4=4 ("index"), index #5=3 ("index"), index #6=2 ("index"), index #7=1 ("index"), index #8=0 ("index")) -> (element #1=w427:u8, element #2=w428:u8, element #3=w429:u8, element #4=w430:u8, element #5=w431:u8, element #6=w432:u8, element #7=w433:u8, element #8=w434:u8)
            n178 = Join Numbers(hi=w427, lo=w428) -> ((hi.lo)=w435:u16)
            n179 = Join Numbers(hi=w429, lo=w430) -> ((hi.lo)=w436:u16)
            n180 = Join Numbers(hi=w431, lo=w432) -> ((hi.lo)=w437:u16)
            n181 = Join Numbers(hi=w433, lo=w434) -> ((hi.lo)=w438:u16)
            n182 = Join Numbers(hi=w435, lo=w436) -> ((hi.lo)=w439:u32)
            n183 = Join Numbers(hi=w437, lo=w438) -> ((hi.lo)=w440:u32)
            n184 = Join Numbers(hi=w439, lo=w440) -> ((hi.lo)=w448:u64)
            "(hi.lo) 2" <- w448
            n185 = Logical Shift(y=i16 0, x=w448) -> (x << y=w458:u64)
            n186 = Logical Shift(y=i16 -2, x=w448) -> (x << y=w459:u64)
            n187 = Logical Shift(y=i16 -12, x=w448) -> (x << y=w460:u64)
            n188 = Logical Shift(y=i16 -21, x=w448) -> (x << y=w461:u64)
            n189 = Logical Shift(y=i16 -23, x=w448) -> (x << y=w462:u64)
            n190 = Logical Shift(y=i16 -33, x=w448) -> (x << y=w463:u64)
            n191 = Logical Shift(y=i16 -42, x=w448) -> (x << y=w464:u64)
            n192 = Logical Shift(y=i16 -44, x=w448) -> (x << y=w465:u64)
            n193 = Logical Shift(y=i16 -54, x=w448) -> (x << y=w466:u64)
            n194 = And(x=w458, y=w467) -> (x .and. y?=w486:u64)
            n195 = And(x=w459, y=w468) -> (x .and. y?=w488:u64)
            n196 = And(x=w461, y=w467) -> (x .and. y?=w485:u64)
            n197 = And(x=w462, y=w468) -> (x .and. y?=w489:u64)
            n198 = And(x=w464, y=w467) -> (x .and. y?=w484:u64)
            n199 = And(x=w465, y=w468) -> (x .and. y?=w487:u64)
            n200 = And(x=w460, y=w469) -> (x .and. y?=w497:u64)
            n201 = And(x=w463, y=w469) -> (x .and. y?=w493:u64)
            n202 = And(x=w466, y=w469) -> (x .and. y?=w495:u64)
            n203 = Logical Shift(y=w470, x=w497) -> (x << y=w471:u64)
            n204 = Logical Shift(y=w470, x=w493) -> (x << y=w472:u64)
            n205 = Logical Shift(y=w470, x=w495) -> (x << y=w473:u64)
            n206 = To Unsigned Byte Integer(number=w486) -> (unsigned 8bit integer=w511:u8)
            n207 = To Unsigned Word Integer(number=w488) -> (unsigned 16bit integer=w510:u16)
            n208 = Decrement(x=w497) -> (x-1=w477:u64)
            n209 = To Unsigned Byte Integer(number=w485) -> (unsigned 8bit integer=w509:u8)
            n210 = To Unsigned Word Integer(number=w489) -> (unsigned 16bit integer=w508:u16)
            n211 = Decrement(x=w493) -> (x-1=w478:u64)
            n212 = To Unsigned Byte Integer(number=w484) -> (unsigned 8bit integer=w506:u8)
            n213 = To Unsigned Word Integer(number=w487) -> (unsigned 16bit integer=w507:u16)
            n214 = Decrement(x=w495) -> (x-1=w479:u64)
            n215 = Not(x=w477) -> (.not. x?=w500:u64)
            n216 = Not Equal To 0?(x=w471) -> (x != 0?=w475:bool)
            n217 = Not(x=w478) -> (.not. x?=w501:u64)
            n218 = Not Equal To 0?(x=w472) -> (x != 0?=w476:bool)
            n219 = Not(x=w479) -> (.not. x?=w503:u64)
            n220 = Not Equal To 0?(x=w473) -> (x != 0?=w474:bool)
            n221 = And(x=w505, y=w500) -> (x .and. y?=w499:u64)
            n222 = And(x=w505, y=w501) -> (x .and. y?=w502:u64)
            n223 = And(x=w505, y=w503) -> (x .and. y?=w504:u64)
            n224 = To Double Precision Float(number=w493) -> (double precision float=w494:dbl)
            n225 = Multiply(x=w483, y=w499) -> (x*y=w480:dbl)
            n226 = Multiply(x=w483, y=w502) -> (x*y=w482:dbl)
            n227 = Multiply(x=w483, y=w504) -> (x*y=w481:dbl)
            n228 = To Double Precision Float(number=w497) -> (double precision float=w498:dbl)
            n229 = To Double Precision Float(number=w495) -> (double precision float=w496:dbl)
            n230 = Select(t=w480, s=w475, f=w498) -> (s? t:f=w490:dbl)
            n231 = Select(t=w482, s=w476, f=w494) -> (s? t:f=w492:dbl)
            n232 = Select(t=w481, s=w474, f=w496) -> (s? t:f=w491:dbl)
            n233 = Bundle By Name(cluster=w417, "Col"=w511, "X"=w510, "Y"=w490) -> (w441:cluster{"Col":dbl, "X":dbl, "Y":dbl})
            n234 = Bundle By Name(cluster=w417, "Col"=w509, "X"=w508, "Y"=w492) -> (w442:cluster{"Col":dbl, "X":dbl, "Y":dbl})
            n235 = Bundle By Name(cluster=w417, "Col"=w506, "X"=w507, "Y"=w491) -> (w443:cluster{"Col":dbl, "X":dbl, "Y":dbl})
            n236 = Build Cluster Array(w441, w442, w443) -> (→"Cones2":T17)
          }
          frame 274 {
            w605 = u64 511 ("y")
            w583 = -1.0 ("y")
            w570 = i16 -8 ("y")
            w569 = u64 511 ("y")
            w568 = u64 1023 ("y")
            w567 = u64 3 ("y")
            n237 = local read "ConeType"() -> (w517:cluster{"Col":dbl, "X":dbl, "Y":dbl})
            n238 = Array Subset(array=w518, index=2, length=8) -> (w547:u8[])
            n239 = Index Array(array=w547, index #1=7 ("index"), index #2=6 ("index"), index #3=5 ("index"), index #4=4 ("index"), index #5=3 ("index"), index #6=2 ("index"), index #7=1 ("index"), index #8=0 ("index")) -> (element #1=w527:u8, element #2=w528:u8, element #3=w529:u8, element #4=w530:u8, element #5=w531:u8, element #6=w532:u8, element #7=w533:u8, element #8=w534:u8)
            n240 = Join Numbers(hi=w527, lo=w528) -> ((hi.lo)=w535:u16)
            n241 = Join Numbers(hi=w529, lo=w530) -> ((hi.lo)=w536:u16)
            n242 = Join Numbers(hi=w531, lo=w532) -> ((hi.lo)=w537:u16)
            n243 = Join Numbers(hi=w533, lo=w534) -> ((hi.lo)=w538:u16)
            n244 = Join Numbers(hi=w535, lo=w536) -> ((hi.lo)=w539:u32)
            n245 = Join Numbers(hi=w537, lo=w538) -> ((hi.lo)=w540:u32)
            n246 = Join Numbers(hi=w539, lo=w540) -> ((hi.lo)=w548:u64)
            "(hi.lo) 3" <- w548
            n247 = Logical Shift(y=i16 0, x=w548) -> (x << y=w558:u64)
            n248 = Logical Shift(y=i16 -2, x=w548) -> (x << y=w559:u64)
            n249 = Logical Shift(y=i16 -12, x=w548) -> (x << y=w560:u64)
            n250 = Logical Shift(y=i16 -21, x=w548) -> (x << y=w561:u64)
            n251 = Logical Shift(y=i16 -23, x=w548) -> (x << y=w562:u64)
            n252 = Logical Shift(y=i16 -33, x=w548) -> (x << y=w563:u64)
            n253 = Logical Shift(y=i16 -42, x=w548) -> (x << y=w564:u64)
            n254 = Logical Shift(y=i16 -44, x=w548) -> (x << y=w565:u64)
            n255 = Logical Shift(y=i16 -54, x=w548) -> (x << y=w566:u64)
            n256 = And(x=w558, y=w567) -> (x .and. y?=w586:u64)
            n257 = And(x=w559, y=w568) -> (x .and. y?=w588:u64)
            n258 = And(x=w561, y=w567) -> (x .and. y?=w585:u64)
            n259 = And(x=w562, y=w568) -> (x .and. y?=w589:u64)
            n260 = And(x=w564, y=w567) -> (x .and. y?=w584:u64)
            n261 = And(x=w565, y=w568) -> (x .and. y?=w587:u64)
            n262 = And(x=w560, y=w569) -> (x .and. y?=w597:u64)
            n263 = And(x=w563, y=w569) -> (x .and. y?=w593:u64)
            n264 = And(x=w566, y=w569) -> (x .and. y?=w595:u64)
            n265 = Logical Shift(y=w570, x=w597) -> (x << y=w571:u64)
            n266 = Logical Shift(y=w570, x=w593) -> (x << y=w572:u64)
            n267 = Logical Shift(y=w570, x=w595) -> (x << y=w573:u64)
            n268 = To Unsigned Byte Integer(number=w586) -> (unsigned 8bit integer=w611:u8)
            n269 = To Unsigned Word Integer(number=w588) -> (unsigned 16bit integer=w610:u16)
            n270 = Decrement(x=w597) -> (x-1=w577:u64)
            n271 = To Unsigned Byte Integer(number=w585) -> (unsigned 8bit integer=w609:u8)
            n272 = To Unsigned Word Integer(number=w589) -> (unsigned 16bit integer=w608:u16)
            n273 = Decrement(x=w593) -> (x-1=w578:u64)
            n274 = To Unsigned Byte Integer(number=w584) -> (unsigned 8bit integer=w606:u8)
            n275 = To Unsigned Word Integer(number=w587) -> (unsigned 16bit integer=w607:u16)
            n276 = Decrement(x=w595) -> (x-1=w579:u64)
            n277 = Not(x=w577) -> (.not. x?=w600:u64)
            n278 = Not Equal To 0?(x=w571) -> (x != 0?=w575:bool)
            n279 = Not(x=w578) -> (.not. x?=w601:u64)
            n280 = Not Equal To 0?(x=w572) -> (x != 0?=w576:bool)
            n281 = Not(x=w579) -> (.not. x?=w603:u64)
            n282 = Not Equal To 0?(x=w573) -> (x != 0?=w574:bool)
            n283 = And(x=w605, y=w600) -> (x .and. y?=w599:u64)
            n284 = And(x=w605, y=w601) -> (x .and. y?=w602:u64)
            n285 = And(x=w605, y=w603) -> (x .and. y?=w604:u64)
            n286 = To Double Precision Float(number=w593) -> (double precision float=w594:dbl)
            n287 = Multiply(x=w583, y=w599) -> (x*y=w580:dbl)
            n288 = Multiply(x=w583, y=w602) -> (x*y=w582:dbl)
            n289 = Multiply(x=w583, y=w604) -> (x*y=w581:dbl)
            n290 = To Double Precision Float(number=w597) -> (double precision float=w598:dbl)
            n291 = To Double Precision Float(number=w595) -> (double precision float=w596:dbl)
            n292 = Select(t=w580, s=w575, f=w598) -> (s? t:f=w590:dbl)
            n293 = Select(t=w582, s=w576, f=w594) -> (s? t:f=w592:dbl)
            n294 = Select(t=w581, s=w574, f=w596) -> (s? t:f=w591:dbl)
            n295 = Bundle By Name(cluster=w517, "Col"=w611, "X"=w610, "Y"=w590) -> (w541:cluster{"Col":dbl, "X":dbl, "Y":dbl})
            n296 = Bundle By Name(cluster=w517, "Col"=w609, "X"=w608, "Y"=w592) -> (w542:cluster{"Col":dbl, "X":dbl, "Y":dbl})
            n297 = Bundle By Name(cluster=w517, "Col"=w606, "X"=w607, "Y"=w591) -> (w543:cluster{"Col":dbl, "X":dbl, "Y":dbl})
            n298 = Build Cluster Array(w541, w542, w543) -> (→"Cones3":T17)
          }
          frame 372 {
            w640 = i16 -32768
            # "Acceleration Y & Yaw"
            n299 = local read "IsStopped"() -> (w628:bool)
            n300 = Index Array(array=w645, index=7) -> (element=w644:u8)
            n301 = Index Array(array=w645, index=6) -> (element=w641:u8)
            n302 = Index Array(array=w645, index=3) -> (element=w643:u8)
            n303 = Index Array(array=w645, index=2) -> (element=w642:u8)
            n304 = case shown="True" w628 {
              frame False {
              }
              frame True {
                n305 = feedback #1() -> (w657:dbl)  [unwired: 1 in]
                n306 = local read "OffsetFilter"() -> (w655:dbl)
                n307 = local read "Acc Y"() -> (w658:dbl)
                n308 = formula code="y_=a*x+(1-a)*y;"("x"=w658, "y"=w657, "a"=w655) -> ("y_"=w656:dbl)
                n309 = feedback-in #1(w656) -> ()
                n310 = local write "Acc Y offset"(w656) -> ()
              }
            }
            n311 = Join Numbers(hi=w644, lo=w641) -> ((hi.lo)=w638:u16)
            n312 = Join Numbers(hi=w643, lo=w642) -> ((hi.lo)=w636:u16)
            n313 = local read "Actual Velocity \nRR [RPM]"() -> (w621:i16)
            n314 = local read "Actual Velocity\nFR [RPM]"() -> (w620:i16)
            n315 = local read "Actual Velocity\nRL [RPM]"() -> (w622:i16)
            n316 = local read "Actual Velocity\nFL [RPM]"() -> (w617:i16)
            n317 = To Word Integer(number=w638) -> (16bit integer=w639:i16)
            n318 = To Word Integer(number=w636) -> (16bit integer=w637:i16)
            n319 = Subtract(x=w639, y=w640) -> (x-y=w635:i16)
            n320 = Subtract(x=w637, y=w640) -> (x-y=w634:i16)
            n321 = Build Array(w617, w620, w621, w622) -> (w623:i16[])
            n322 = To Double Precision Float(number=w617) -> (double precision float=w618:dbl)
            n323 = Array Max & Min(array=w623) -> (min value=w619:i16)  [unwired: 3 out]
            n324 = To Double Precision Float(number=w635) -> (double precision float=w633:dbl)
            n325 = To Double Precision Float(number=w634) -> (double precision float=w632:dbl)
            n326 = Divide(x=w618, y=148.96908) -> (x/y=w613:dbl)
            n327 = To Double Precision Float(number=w619) -> (double precision float=w615:dbl)
            n328 = Multiply(x=w632, y=0.005) -> (x*y=→"Yaw" →"Yaw Rear":dbl)
            n329 = Multiply(x=w633, y=0.0001274) -> (x*y=→"Acc Y":dbl)
            n330 = Multiply(x=w613, y=0.227) -> (x*y=w612:dbl)
            n331 = Divide(x=w615, y=677.4732) -> ()  [unwired: 1 out]
            n332 = Subtract(x=w612, y=w615) -> (x-y=w614:dbl)
            n333 = Divide(x=w614, y=w612) -> (x/y=→"Slip":dbl)
          }
          frame 376 {
            w694 = i16 -32768
            # "Acceleration X & Roll"
            n334 = local read "IsStopped"() -> (w660:bool)
            n335 = Index Array(array=w699, index=7) -> (element=w698:u8)
            n336 = Index Array(array=w699, index=6) -> (element=w695:u8)
            n337 = Index Array(array=w699, index=3) -> (element=w697:u8)
            n338 = Index Array(array=w699, index=2) -> (element=w696:u8)
            n339 = case shown="True" w660 {
              frame False {
              }
              frame True {
                n340 = feedback #2() -> (w711:dbl)  [unwired: 1 in]
                n341 = local read "OffsetFilter"() -> (w709:dbl)
                n342 = local read "Roll"() -> (w712:dbl)
                n343 = formula code="y_=a*x+(1-a)*y;"("x"=w712, "y"=w711, "a"=w709) -> ("y_"=w710:dbl)
                n344 = feedback-in #2(w710) -> ()
                n345 = local write "Rollrate offset"(w710) -> ()
              }
            }
            n346 = Join Numbers(hi=w698, lo=w695) -> ((hi.lo)=w692:u16)
            n347 = Join Numbers(hi=w697, lo=w696) -> ((hi.lo)=w690:u16)
            n348 = feedback #3() -> (w665:dbl)  [unwired: 1 in]
            n349 = feedback #4() -> (w682:dbl[])  [unwired: 1 in]
            n350 = feedback #5() -> (w668:dbl)  [unwired: 1 in]
            n351 = feedback #6() -> (w675:dbl[])  [unwired: 1 in]
            n352 = local read "Acc Y"() -> (w663:dbl)
            n353 = local read "Acc Z"() -> (w667:dbl)
            n354 = formula code="y_=a*x+(1-a)*y;"("x"=w663, "y"=w665, "a"=0.02 ("input variable")) -> ("y_"=w662:dbl)
            "accY" <- w662
            n355 = feedback-in #3(w662) -> ()
            n356 = formula code="y_=a*x+(1-a)*y;"("x"=w667, "y"=w668, "a"=0.02 ("input variable")) -> ("y_"=w661:dbl)
            "accZ" <- w661
            n357 = feedback-in #5(w661) -> ()
            n358 = To Word Integer(number=w692) -> (16bit integer=w693:i16)
            n359 = To Word Integer(number=w690) -> (16bit integer=w691:i16)
            n360 = Subtract(x=w693, y=w694) -> (x-y=w689:i16)
            n361 = Subtract(x=w691, y=w694) -> (x-y=w688:i16)
            n362 = To Double Precision Float(number=w689) -> (double precision float=w687:dbl)
            n363 = To Double Precision Float(number=w688) -> (double precision float=w686:dbl)
            n364 = Build Array (concatenate)(w675, w661) -> (w676:dbl[])
            n365 = Build Array (concatenate)(w682, w662) -> (w680:dbl[])
            n366 = Build Array(w662) -> (w673:dbl[])
            n367 = Build Array(w661) -> (w672:dbl[])
            n368 = Multiply(x=w686, y=0.005) -> (x*y=→"Roll":dbl)
            n369 = Multiply(x=w687, y=0.0001274) -> (x*y=→"Acc X":dbl)
            n370 = Array Size(array=w680) -> (size(s)=w679:i32)
            n371 = Bundle(w673, w672) -> (w669:cluster{dbl[], dbl[]})  [unwired: 1 in]
            n372 = Less?(x=w679, y=1000) -> (x < y?=w677:bool)
            n373 = case shown="False" w677 {
              tunnel: [w713 w722] -> w674
              tunnel: w676 -> [w714 w722]
              tunnel: [w717 w721] -> w681
              tunnel: w680 -> [w720 w721]
              frame False {
                n374 = Delete From Array(array=w720, length=1, index=0) -> (array with subset deleted=w717:dbl[])  [unwired: 1 out]
                n375 = Delete From Array(array=w714, length=1, index=0) -> (array with subset deleted=w713:dbl[])  [unwired: 1 out]
              }
              frame True {
              }
            }
            n376 = feedback-in #4(w681) -> ()
            n377 = feedback-in #6(w674) -> ()
            n378 = Bundle(w681, w674) -> (w670:cluster{dbl[], dbl[]})  [unwired: 1 in]
            n379 = Build Array(w669, w670) -> (→"XY Graph":cluster{dbl[], dbl[]}[])
          }
          frame 380 {
            w727 = u16 200 ("y")
            # "Acceleration Z"
            n380 = local read "AccelXRaw"() -> (w732:dbl)
            n381 = local read "IsStopped"() -> (w733:bool)
            n382 = local read "BrakeRaw"() -> (w728:u16)
            n383 = local read "TorqRaw"() -> (w729:u16)
            n384 = Index Array(array=w748, index=7) -> (element=w747:u8)
            n385 = Index Array(array=w748, index=6) -> (element=w746:u8)
            n386 = case shown="True" w733 {
              frame False {
              }
              frame True {
                n387 = feedback #7() -> (w760:dbl)  [unwired: 1 in]
                n388 = local read "OffsetFilter"() -> (w758:dbl)
                n389 = local read "Acc Z"() -> (w761:dbl)
                n390 = formula code="y_=a*x+(1-a)*y;"("x"=w761, "y"=w760, "a"=w758) -> ("y_"=w759:dbl)
                n391 = feedback-in #7(w759) -> ()
                n392 = local write "Acc Z offset"(w759) -> ()
              }
            }
            n393 = Less?(x=w729, y=w727) -> (x < y?=w725:bool)
            n394 = Less?(x=w728, y=w727) -> (x < y?=w726:bool)
            n395 = Join Numbers(hi=w747, lo=w746) -> ((hi.lo)=w743:u16)
            n396 = Multiply(x=0.01, y=w732) -> (x*y=w738:dbl)
            n397 = local read "Velocity [km/h]"() -> (w735:dbl)
            n398 = And(x=w725, y=w726) -> (x .and. y?=w724:bool)
            n399 = To Word Integer(number=w743) -> (16bit integer=w744:i16)
            n400 = Divide(x=w735, y=3.6) -> (x/y=w723:dbl)
            n401 = Subtract(x=w744, y=i16 -32768) -> (x-y=w742:i16)
            n402 = feedback #8(w723) -> (w739:dbl)
            n403 = Add(x=w739, y=w738) -> (x+y=w731:dbl)
            n404 = case shown="False" w724 {
              tunnel: w731 -> [w756 _]
              tunnel: [w756 w757] -> w730
              tunnel: w723 -> [_ w757]
              frame False {
              }
              frame True {
              }
            }
            "Vel_acc" <- w730
            n405 = feedback-in #8(w730) -> ()
            n406 = To Double Precision Float(number=w742) -> (double precision float=w741:dbl)
            n407 = Multiply(x=w741, y=0.0001274) -> (x*y=→"Acc Z":dbl)
          }
          frame 389 {
            # "TCU FL"
            n408 = Index Array(array=w769, index=7) -> (element=w790:u8)
            n409 = Index Array(array=w769, index=6) -> (element=w789:u8)
            n410 = Index Array(array=w769, index=9) -> (element=w786:u8)
            n411 = Index Array(array=w769, index=8) -> (element=w785:u8)
            n412 = Index Array(array=w769, index=5) -> (element=w768:u8)
            n413 = Index Array(array=w769, index=4) -> (element=w767:u8)
            n414 = Index Array(array=w769, index=3) -> (element=w774:u8)
            n415 = Join Numbers(hi=w790, lo=w789) -> ((hi.lo)=w776:u16)
            n416 = Join Numbers(hi=w786, lo=w785) -> ((hi.lo)=w778:u16)
            n417 = Join Numbers(hi=w768, lo=w767) -> ((hi.lo)=w766:u16)
            n418 = Number To Boolean Array(number=w774) -> (Boolean array=→"TCU FL Status":bool[])
            n419 = To Word Integer(number=w776) -> (16bit integer=w779:i16)
            n420 = To Word Integer(number=w778) -> (16bit integer=w777:i16)
            n421 = To Word Integer(number=w766) -> (16bit integer=w765:i16)
            n422 = To Double Precision Float(number=w765) -> (double precision float=→"FL Velocity":dbl)
            n423 = To Double Precision Float(number=w779) -> (double precision float=w763:dbl)
            "FL" <- w763
            "FL Torque Pos" <- w763
            n424 = To Double Precision Float(number=w777) -> (double precision float=w762:dbl)
            "FL 2" <- w762
            "FL Torque Neg" <- w762
            n425 = Add(x=w763, y=w762) -> (x+y=→"TCU FL":dbl)
          }
          frame 390 {
            # "TCU FR"
            n426 = Index Array(array=w796, index=7) -> (element=w821:u8)
            n427 = Index Array(array=w796, index=6) -> (element=w820:u8)
            n428 = Index Array(array=w796, index=9) -> (element=w817:u8)
            n429 = Index Array(array=w796, index=8) -> (element=w816:u8)
            n430 = Index Array(array=w796, index=5) -> (element=w800:u8)
            n431 = Index Array(array=w796, index=4) -> (element=w799:u8)
            n432 = Index Array(array=w796, index=3) -> (element=w805:u8)
            n433 = Join Numbers(hi=w821, lo=w820) -> ((hi.lo)=w809:u16)
            n434 = Join Numbers(hi=w817, lo=w816) -> ((hi.lo)=w807:u16)
            n435 = Join Numbers(hi=w800, lo=w799) -> ((hi.lo)=w798:u16)
            n436 = Number To Boolean Array(number=w805) -> (Boolean array=→"TCU FR Status":bool[])
            n437 = To Word Integer(number=w809) -> (16bit integer=w810:i16)
            n438 = To Word Integer(number=w807) -> (16bit integer=w808:i16)
            n439 = To Word Integer(number=w798) -> (16bit integer=w797:i16)
            n440 = To Double Precision Float(number=w797) -> (double precision float=→"FR Velocity":dbl)
            n441 = To Double Precision Float(number=w810) -> (double precision float=w794:dbl)
            "FR" <- w794
            "FR Torque Pos" <- w794
            n442 = To Double Precision Float(number=w808) -> (double precision float=w793:dbl)
            "FR 2" <- w793
            "FR Torque Neg" <- w793
            n443 = Add(x=w794, y=w793) -> (x+y=→"TCU FR":dbl)
          }
          frame 393 {
            # "TCU RL"
            n444 = Index Array(array=w827, index=7) -> (element=w852:u8)
            n445 = Index Array(array=w827, index=6) -> (element=w851:u8)
            n446 = Index Array(array=w827, index=9) -> (element=w848:u8)
            n447 = Index Array(array=w827, index=8) -> (element=w847:u8)
            n448 = Index Array(array=w827, index=5) -> (element=w831:u8)
            n449 = Index Array(array=w827, index=4) -> (element=w830:u8)
            n450 = Index Array(array=w827, index=3) -> (element=w836:u8)
            n451 = Join Numbers(hi=w852, lo=w851) -> ((hi.lo)=w839:u16)
            n452 = Join Numbers(hi=w848, lo=w847) -> ((hi.lo)=w838:u16)
            n453 = Join Numbers(hi=w831, lo=w830) -> ((hi.lo)=w829:u16)
            n454 = Number To Boolean Array(number=w836) -> (Boolean array=→"TCU RL Status":bool[])
            n455 = To Word Integer(number=w839) -> (16bit integer=w841:i16)
            n456 = To Word Integer(number=w838) -> (16bit integer=w840:i16)
            n457 = To Word Integer(number=w829) -> (16bit integer=w828:i16)
            n458 = To Double Precision Float(number=w828) -> (double precision float=→"RL Velocity":dbl)
            n459 = To Double Precision Float(number=w841) -> (double precision float=w825:dbl)
            "RL" <- w825
            "RL Torque Pos" <- w825
            n460 = To Double Precision Float(number=w840) -> (double precision float=w824:dbl)
            "RL 2" <- w824
            "RL Torque Neg" <- w824
            n461 = Add(x=w825, y=w824) -> (x+y=→"TCU RL":dbl)
          }
          frame 394 {
            # "TCU RR"
            n462 = Index Array(array=w858, index=7) -> (element=w883:u8)
            n463 = Index Array(array=w858, index=6) -> (element=w882:u8)
            n464 = Index Array(array=w858, index=9) -> (element=w879:u8)
            n465 = Index Array(array=w858, index=8) -> (element=w878:u8)
            n466 = Index Array(array=w858, index=5) -> (element=w862:u8)
            n467 = Index Array(array=w858, index=4) -> (element=w861:u8)
            n468 = Index Array(array=w858, index=3) -> (element=w867:u8)
            n469 = Join Numbers(hi=w883, lo=w882) -> ((hi.lo)=w869:u16)
            n470 = Join Numbers(hi=w879, lo=w878) -> ((hi.lo)=w875:u16)
            n471 = Join Numbers(hi=w862, lo=w861) -> ((hi.lo)=w860:u16)
            n472 = Number To Boolean Array(number=w867) -> (Boolean array=→"TCU RR Status":bool[])
            n473 = To Word Integer(number=w869) -> (16bit integer=w870:i16)
            n474 = To Word Integer(number=w875) -> (16bit integer=w874:i16)
            n475 = To Word Integer(number=w860) -> (16bit integer=w859:i16)
            n476 = To Double Precision Float(number=w859) -> (double precision float=→"RR Velocity":dbl)
            n477 = To Double Precision Float(number=w870) -> (double precision float=w856:dbl)
            "RR" <- w856
            "RR Torque Pos" <- w856
            n478 = To Double Precision Float(number=w874) -> (double precision float=w855:dbl)
            "RR 2" <- w855
            "RR Torque Neg" <- w855
            n479 = Add(x=w856, y=w855) -> (x+y=→"TCU RR":dbl)
          }
          frame 436 {
            w898 = i16 -32768
            # "Acceleration Y & Yaw"
            n480 = Index Array(array=w903, index=7) -> (element=w902:u8)
            n481 = Index Array(array=w903, index=6) -> (element=w899:u8)
            n482 = Index Array(array=w903, index=3) -> (element=w901:u8)
            n483 = Index Array(array=w903, index=2) -> (element=w900:u8)
            n484 = Join Numbers(hi=w902, lo=w899) -> ((hi.lo)=w896:u16)
            n485 = Join Numbers(hi=w901, lo=w900) -> ((hi.lo)=w894:u16)
            n486 = To Word Integer(number=w896) -> (16bit integer=w897:i16)
            n487 = To Word Integer(number=w894) -> (16bit integer=w895:i16)
            n488 = Subtract(x=w897, y=w898) -> (x-y=w893:i16)
            n489 = Subtract(x=w895, y=w898) -> (x-y=w892:i16)
            n490 = To Double Precision Float(number=w893) -> (double precision float=w891:dbl)
            n491 = To Double Precision Float(number=w892) -> (double precision float=w890:dbl)
            n492 = Multiply(x=w890, y=0.005) -> (x*y=→"Yaw 2" →"Yaw Front":dbl)
            n493 = Multiply(x=w891, y=0.0001274) -> (x*y=→"Acc Y 2":dbl)
          }
          frame 440 {
            w927 = i16 -32768
            # "Acceleration X & Roll"
            n494 = local read "Data Source"() -> (w914:u16)
            n495 = local read "IsStopped"() -> (w915:bool)
            n496 = Index Array(array=w932, index=7) -> (element=w931:u8)
            n497 = Index Array(array=w932, index=6) -> (element=w928:u8)
            n498 = Index Array(array=w932, index=3) -> (element=w930:u8)
            n499 = Index Array(array=w932, index=2) -> (element=w929:u8)
            n500 = case shown="True" w915 {
              frame False {
              }
              frame True {
                n501 = feedback #9() -> (w1042:dbl)  [unwired: 1 in]
                n502 = local read "OffsetFilter"() -> (w1040:dbl)
                n503 = local read "Acc X 2"() -> (w1043:dbl)
                n504 = formula code="y_=a*x+(1-a)*y;"("x"=w1043, "y"=w1042, "a"=w1040) -> ("y_"=w1041:dbl)
                n505 = feedback-in #9(w1041) -> ()
                n506 = local write "Acc X offset 2"(w1041) -> ()
              }
            }
            n507 = case shown="2" w914 {
              frame 0, Default {
              }
              frame 2 {
                (unwired) cluster{dbl, u32}[] [{-1.5, 255}, {0.0, 61192}, {1.5, 16711680}] ("Z Scale.Marker Values[]")
                w945 = 500 ("dimension size")
                n508 = feedback #10() -> (w975:dbl)  [unwired: 1 in]
                n509 = feedback #11(0.0) -> (w967:dbl)
                n510 = Greater?(x=w967, y=200.0) -> (0:w971:bool)
                n511 = local read "Acc Z 2"() -> (w949:dbl)
                n512 = local read "Roll 2"() -> (w973:dbl)
                n513 = Initialize Array(-100.0 ("element"), w945, w945) -> (w944:dbl[][])
                n514 = formula code="y_=a*x+(1-a)*y;"("x"=w973, "y"=w975, "a"=0.5 ("input variable")) -> ("y_"=w972:dbl)
                n515 = feedback-in #10(w972) -> ()
                n516 = feedback #12(dbl[] []) -> (w989:dbl[])
                n517 = feedback #13(dbl[] []) -> (w988:dbl[])
                n518 = feedback #14(dbl[] []) -> (w950:dbl[])
                n519 = local read "Velocity [km/h]"() -> (w981:dbl)
                n520 = Build Array (concatenate)(w950, w949) -> (w942:dbl[])
                n521 = feedback-in #14(w942) -> ()
                n522 = Divide(x=w981, y=3.6) -> (x/y=w983:dbl)
                n523 = Subtract(x=w972, y="Rollrate offset") -> (x-y=w974:dbl)
                n524 = feedback #15() -> (w994:dbl)  [unwired: 1 in]
                n525 = feedback #16() -> (w992:dbl)  [unwired: 1 in]
                n526 = Divide(x=w974, y=180.0 ("Yaw")) -> (x/y=w980:dbl)
                n527 = feedback #17() -> (w995:dbl)  [unwired: 1 in]
                n528 = Multiply(x=3.141592653589793, y=w980) -> (x*y=w978:dbl)
                n529 = formula code="ve=v*cos(phi);\nvn=v*sin(phi);\nse=sx+ve*ts;\nsn=sy+vn*ts;\nphi_=phi+yaw*ts;"("phi"=w992, "yaw"=w978, "ts"=0.01 ("input variable"), "sx"=w995, "sy"=w994, "v"=w983) -> ("se"=w990:dbl, "sn"=w987:dbl, "phi_"=w993:dbl)  [unwired: 4 out]
                n530 = feedback-in #15(w987) -> ()
                n531 = feedback-in #16(w993) -> ()
                n532 = feedback-in #17(w990) -> ()
                n533 = Build Array (concatenate)(w989, w990) -> (w965:dbl[])
                n534 = feedback-in #12(w965) -> ()
                n535 = Build Array (concatenate)(w988, w987) -> (w964:dbl[])
                n536 = feedback-in #13(w964) -> ()
                n537 = Bundle(w965, w964) -> (→"XY Graph 2":cluster{dbl[], dbl[]})  [unwired: 1 in]
                n538 = feedback #18() -> (w958:dbl)  [unwired: 1 in]
                n539 = feedback #19() -> (w954:dbl)  [unwired: 1 in]
                n540 = feedback #20() -> (w956:dbl)  [unwired: 1 in]
                n541 = case shown="True" w971 {
                  tunnel: w965 -> [_ w1039]
                  tunnel: w964 -> [_ w1038]
                  tunnel: [w1004 0.0] -> w969
                  tunnel: w967 -> [w1005 _]
                  tunnel: [w1003 w1019] -> w959
                  tunnel: [w1001 w1018] -> w955
                  tunnel: [w1002 w1017] -> w957
                  tunnel: w958 -> [w1003 _]
                  tunnel: w956 -> [w1002 _]
                  tunnel: w954 -> [w1001 _]
                  tunnel: w942 -> [_ w1006]
                  frame False {
                    n542 = Increment(x=w1005) -> (x+1=w1004:dbl)
                  }
                  frame True {
                    n543 = Array Max & Min(array=w1006) -> (max value=w1016:dbl, min value=w1015:dbl)  [unwired: 2 out]
                    n544 = Array Max & Min(array=w1039) -> (max value=w1033:dbl, min value=w1034:dbl)  [unwired: 2 out]
                    n545 = Array Max & Min(array=w1038) -> (max value=w1025:dbl, min value=w1024:dbl)  [unwired: 2 out]
                    n546 = Add(x=w1033, y=w1034) -> (x+y=w1032:dbl)
                    n547 = Subtract(x=w1033, y=w1034) -> (x-y=w1037:dbl)
                    n548 = Subtract(x=w1025, y=w1024) -> (x-y=w1036:dbl)
                    n549 = Add(x=w1025, y=w1024) -> (x+y=w1026:dbl)
                    n550 = Bundle(w1016, u32 16711680) -> (w1014:cluster{dbl, u32})  [unwired: 1 in]
                    n551 = Bundle(w1015, u32 255) -> (w1012:cluster{dbl, u32})  [unwired: 1 in]
                    n552 = Build Array(w1037, w1036) -> (w1035:dbl[])
                    n553 = Divide(x=w1032, y=2.0) -> (x/y=w1029:dbl)
                    n554 = Divide(x=w1026, y=2.0) -> (x/y=w1022:dbl)
                    n555 = Bundle("y"=0.0, u32 6618880) -> (w1013:cluster{"y":dbl, u32})  [unwired: 1 in]
                    n556 = Build Array(w1012, w1013, w1014) -> (w1007:cluster{"y":dbl, u32}[])
                    n557 = Array Max & Min(array=w1035) -> (max value=w1017:dbl)  [unwired: 3 out]
                    n558 = property on="Intensity Graph" class="IntGraph (strict)"("ZScale.MarkerVals[]"=w1007) -> ()  [unwired: 2 in, 2 out]
                    n559 = Divide(x=w1017, y=2.0) -> (x/y=w1021:dbl)
                    n560 = Add(x=w1029, y=w1021) -> (x+y=w1028:dbl)
                    n561 = Add(x=w1022, y=w1021) -> (x+y=w1023:dbl)
                    n562 = Subtract(x=w1029, y=w1021) -> (x-y=w1019:dbl)
                    n563 = Subtract(x=w1022, y=w1021) -> (x-y=w1018:dbl)
                    n564 = property on="XY Graph 2" class="XYGraph (strict)"("XScale.Maximum"=w1028) -> ()  [unwired: 2 in, 2 out]
                    n565 = property on="XY Graph 2" class="XYGraph (strict)"("XScale.Minimum"=w1019) -> ()  [unwired: 2 in, 2 out]
                    n566 = property on="XY Graph 2" class="XYGraph (strict)"("YScale.Maximum"=w1023) -> ()  [unwired: 2 in, 2 out]
                    n567 = property on="XY Graph 2" class="XYGraph (strict)"("YScale.Minimum"=w1018) -> ()  [unwired: 2 in, 2 out]
                  }
                }
                n568 = feedback-in #11(w969) -> ()
                n569 = feedback-in #18(w959) -> ()
                n570 = feedback-in #19(w955) -> ()
                n571 = feedback-in #20(w957) -> ()
                n572 = Subtract(x=w965, y=w959) -> (x-y=w963:dbl[])
                n573 = Subtract(x=w964, y=w955) -> (x-y=w962:dbl[])
                n574 = Divide(x=w957, y=500.0) -> (x/y=w960:dbl)
                n575 = Divide(x=w963, y=w960) -> (x/y=w953:dbl[])
                n576 = Divide(x=w962, y=w960) -> (x/y=w952:dbl[])
                n577 = Round To Nearest(number=w953) -> (nearest integer value=w948:dbl[])
                n578 = Round To Nearest(number=w952) -> (nearest integer value=w947:dbl[])
                n579 = for {
                  tunnel: w948 -> [w1000] mode=indexing
                  tunnel: w947 -> [w999] mode=indexing
                  tunnel: w942 -> [w998] mode=indexing
                  shift-right: [w996] -> w943
                  shift-left: w944 -> [w997]
                  n580 = Replace Array Subset(array=w997, new element=w998, index (row)=w1000, index (col)=w999) -> (w996:dbl[][])
                }
                "Intensity Graph" <- w943
              }
            }
            n581 = Join Numbers(hi=w931, lo=w928) -> ((hi.lo)=w925:u16)
            n582 = Join Numbers(hi=w930, lo=w929) -> ((hi.lo)=w923:u16)
            n583 = To Word Integer(number=w925) -> (16bit integer=w926:i16)
            n584 = To Word Integer(number=w923) -> (16bit integer=w924:i16)
            n585 = Subtract(x=w926, y=w927) -> (x-y=w922:i16)
            n586 = Subtract(x=w924, y=w927) -> (x-y=w921:i16)
            n587 = To Double Precision Float(number=w922) -> (double precision float=w920:dbl)
            n588 = To Double Precision Float(number=w921) -> (double precision float=w919:dbl)
            n589 = Multiply(x=w919, y=0.005) -> (x*y=→"Roll 2":dbl)
            n590 = Multiply(x=w920, y=0.0001274) -> (x*y=→"Acc X 2":dbl)
          }
          frame 444 {
            # "Acceleration Z"
            n591 = Index Array(array=w1053, index=7) -> (element=w1052:u8)
            n592 = Index Array(array=w1053, index=6) -> (element=w1051:u8)
            n593 = Join Numbers(hi=w1052, lo=w1051) -> ((hi.lo)=w1048:u16)
            n594 = To Word Integer(number=w1048) -> (16bit integer=w1049:i16)
            n595 = Subtract(x=w1049, y=i16 -32768) -> (x-y=w1047:i16)
            n596 = To Double Precision Float(number=w1047) -> (double precision float=w1046:dbl)
            n597 = Multiply(x=w1046, y=0.0001274) -> (x*y=→"Acc Z 2":dbl)
          }
          frame 402 {
            n598 = Index Array(array=w1075, index=2) -> (element=w1064:u8)
            n599 = Number To Boolean Array(number=w1064) -> (Boolean array=w1073:bool[])
            n600 = Index Array(array=w1073, index #1=7 ("index"), index #2=6 ("index"), index #3=5 ("index"), index #4=4 ("index"), index #5=3 ("index"), index #6=2 ("index"), index #7=1 ("index"), index #8=0 ("index")) -> (element #6=→"RES BUTTON":bool, element #7=→"RES GO":bool, element #8=→"RES EBS":bool)  [unwired: 5 out]
          }
          frame 512 {
            # "Torque signal"
            # "Pedalbox Throttle Steering"
            n601 = local read "TCU Version"() -> (w1101:u16)
            n602 = Index Array(array=w1082, index=6) -> (element=w1089:u8)
            n603 = Index Array(array=w1082, index=7) -> (element=w1088:u8)
            n604 = Index Array(array=w1082, index=4) -> (element=w1103:u8)
            n605 = Index Array(array=w1082, index=5) -> (element=w1102:u8)
            n606 = Index Array(array=w1082, index=2) -> (element=w1095:u8)
            n607 = Index Array(array=w1082, index=3) -> (element=w1094:u8)
            n608 = formula code="out = (in1 << 8) | in2;"("in1"=w1089, "in2"=w1088) -> ("out"=→"STA1":dbl)
            n609 = formula code="out = (in1 << 8) | in2;"("in1"=w1103, "in2"=w1102) -> ("out"=→"TPS2_Raw":dbl)
            n610 = formula code="out = (in1 << 8) | in2;"("in1"=w1095, "in2"=w1094) -> ("out"=→"TorqRaw 2" →"TPS1_Raw":dbl)
            n611 = Subtract(x=w1101, y=u16 2016) -> (x-y=w1099:u16)
            n612 = Subtract(x="Torque Max", y="Torque Min") -> (x-y=w1114:dbl)
            n613 = Join Numbers(hi=w1103, lo=w1102) -> ((hi.lo)=w1104:u16)
            n614 = Subtract(x=w1104, y="Torque Min") -> (x-y=w1115:dbl)
            n615 = Index Array(array=w1082, index=8) -> (element=w1084:u8)
            n616 = Index Array(array=w1082, index=9) -> (element=w1083:u8)
            n617 = case shown="1" w1099 {
              tunnel: w1082 -> [w1122 w1145]
              tunnel: [i16 0 ("STA1") w1140] -> _
              tunnel: [i16 0 ("STA1") w1135] -> _
              tunnel: [w1119 w1136] -> _
              tunnel: [w1118 i16 0 ("STA1")] -> w1098
              frame 0, Default {
                # "TCU 2016"
                n618 = Index Array(array=w1122, index=8) -> (element=w1125:u8)
                n619 = Index Array(array=w1122, index=9) -> (element=w1126:u8)
                n620 = Join Numbers(hi=w1125, lo=w1126) -> ((hi.lo)=w1118:u16)
                n621 = Subtract(x="Steering Max", y="Steering Min") -> (x-y=w1132:dbl)
                n622 = Subtract(x=w1118, y="Steering Null") -> (x-y=w1127:dbl)
                n623 = Divide(x=w1127, y=w1132) -> (x/y=w1128:dbl)
                n624 = Multiply(x=360.0, y=w1128) -> (x*y=w1119:dbl)
              }
              frame 1 {
                # "TCU 2017"
                n625 = Index Array(array=w1145, index=6) -> (element=w1151:u8)
                n626 = Index Array(array=w1145, index=7) -> (element=w1148:u8)
                n627 = Index Array(array=w1145, index=8) -> (element=w1144:u8)
                n628 = Index Array(array=w1145, index=9) -> (element=w1143:u8)
                n629 = Join Numbers(hi=w1144, lo=w1143) -> ((hi.lo)=w1141:u16)
                n630 = And(x=w1151, y=u8 127) -> (x .and. y?=w1150:u8)
                n631 = Subtract(x=w1141, y=i16 3600) -> (x-y=w1135:u16)
                n632 = Join Numbers(hi=w1150, lo=w1148) -> ((hi.lo)=w1149:u16)
                n633 = Subtract(x=w1149, y=i16 3600) -> (x-y=w1140:u16)
                n634 = To Word Integer(number=w1135) -> (16bit integer=w1138:i16)
                n635 = To Double Precision Float(number=w1138) -> (double precision float=w1137:dbl)
                n636 = Divide(x=w1137, y=10.0) -> (x/y=w1136:dbl)
              }
            }
            "SteeringRaw" <- w1098
            n637 = formula code="out = (in1 << 8) | in2;"("in1"=w1084, "in2"=w1083) -> ("out"=→"STA2":dbl)
            n638 = Divide(x=w1115, y=w1114) -> (x/y=w1111:dbl)
            n639 = Multiply(x=100.0, y=w1111) -> ()  [unwired: 1 out]
          }
          frame 513 {
            w1197 = 16.375 ("y")
            # "Pedalbox Brake"
            n640 = local read "Brake_Threshold"() -> (w1161:u8)
            n641 = local read "TC_Param"() -> (w1160:u8)
            n642 = Subtract(x="Brake Max", y="Brake Min") -> (x-y=w1227:dbl)
            n643 = Index Array(array=w1193, index=2) -> (element=w1188:u8)
            n644 = Index Array(array=w1193, index=4) -> (element=w1192:u8)
            n645 = Index Array(array=w1193, index=6) -> (element=w1218:u8)
            n646 = Index Array(array=w1193, index=8) -> (element=w1208:u8)
            n647 = Subtract(x="Brake Max 2", y="Brake Min 2") -> (x-y=w1216:dbl)
            n648 = Subtract(x="Brake Max 2", y="Brake Min 2") -> (x-y=w1206:dbl)
            n649 = Index Array(array=w1193, index=3) -> (element=w1186:u8)
            n650 = Index Array(array=w1193, index=5) -> (element=w1231:u8)
            n651 = Index Array(array=w1193, index=7) -> (element=w1211:u8)
            n652 = Index Array(array=w1193, index=9) -> (element=w1201:u8)
            n653 = feedback #21() -> (w1180:dbl[])  [unwired: 1 in]
            n654 = feedback #22() -> (w1173:dbl[])  [unwired: 1 in]
            n655 = And(x=w1188, y=u8 15) -> (x .and. y?=w1187:u8)
            n656 = And(x=w1192, y=u8 15) -> (x .and. y?=w1191:u8)
            n657 = And(x=w1218, y=u8 15) -> (x .and. y?=w1212:u8)
            n658 = And(x=w1208, y=u8 15) -> (x .and. y?=w1202:u8)
            n659 = Join Numbers(hi=w1187, lo=w1186) -> ((hi.lo)=→"BPS1_Raw":u16)
            n660 = feedback #23() -> (w1166:dbl)  [unwired: 1 in]
            n661 = Join Numbers(hi=w1191, lo=w1231) -> ((hi.lo)=w1184:u16)
            "BPS2_Raw" <- w1184
            n662 = Join Numbers(hi=w1212, lo=w1211) -> ((hi.lo)=w1182:u16)
            "BPR_Raw" <- w1182
            n663 = Join Numbers(hi=w1202, lo=w1201) -> ((hi.lo)=w1181:u16)
            "BrakeRaw 2" <- w1181
            "BPF_Raw" <- w1181
            n664 = feedback #24() -> (w1168:dbl)  [unwired: 1 in]
            n665 = Subtract(x=w1184, y="Brake Min") -> (x-y=w1228:dbl)
            n666 = Subtract(x=w1182, y="Brake Min 2") -> (x-y=w1196:dbl)
            n667 = Subtract(x=w1181, y="Brake Min 2") -> (x-y=w1183:dbl)
            n668 = local read "BP_front"() -> (w1157:i16)
            n669 = local read "BP_rear"() -> (w1156:i16)
            n670 = Divide(x=w1228, y=w1227) -> (x/y=w1226:dbl)
            n671 = Divide(x=w1196, y=w1216) -> (x/y=w1215:dbl)
            n672 = Divide(x=w1183, y=w1206) -> (x/y=w1205:dbl)
            n673 = Divide(x=w1196, y=w1197) -> ()  [unwired: 1 out]
            n674 = Divide(x=w1183, y=w1197) -> ()  [unwired: 1 out]
            n675 = Multiply(x=100.0, y=w1226) -> ()  [unwired: 1 out]
            n676 = formula code="y_=a*x+(1-a)*y;"("x"=w1157, "y"=w1166, "a"=0.02 ("input variable")) -> ("y_"=w1164:dbl)
            n677 = feedback-in #23(w1164) -> ()
            n678 = formula code="y_=a*x+(1-a)*y;"("x"=w1156, "y"=w1168, "a"=0.02 ("input variable")) -> ("y_"=w1163:dbl)
            "accZ 2" <- w1163
            n679 = feedback-in #24(w1163) -> ()
            n680 = Bundle("BP_front"=w1157, "BP_rear"=w1156, "Brake_Threshold"=w1161, "TC_Param"=w1160) -> (→"Brake Pressure":T7)  [unwired: 1 in]
            n681 = Multiply(x=100.0, y=w1215) -> (x*y=→"Brake Front":dbl)
            n682 = Multiply(x=100.0, y=w1205) -> (x*y=→"Brake Rear":dbl)
            n683 = Build Array (concatenate)(w1180, w1164) -> (w1178:dbl[])
            n684 = Build Array(w1164) -> (w1171:dbl[])
            n685 = Array Size(array=w1178) -> (size(s)=w1177:i32)
            n686 = Build Array (concatenate)(w1173, w1163) -> (w1174:dbl[])
            n687 = Build Array(w1163) -> (w1170:dbl[])
            n688 = Bundle(w1171, w1170) -> (w1158:cluster{dbl[], dbl[]})  [unwired: 1 in]
            n689 = Less?(x=w1177, y=1000) -> (x < y?=w1175:bool)
            n690 = case shown="False" w1175 {
              tunnel: [w1234 w1243] -> w1172
              tunnel: w1174 -> [w1235 w1243]
              tunnel: [w1238 w1242] -> w1179
              tunnel: w1178 -> [w1241 w1242]
              frame False {
                n691 = Delete From Array(array=w1241, length=1, index=0) -> (array with subset deleted=w1238:dbl[])  [unwired: 1 out]
                n692 = Delete From Array(array=w1235, length=1, index=0) -> (array with subset deleted=w1234:dbl[])  [unwired: 1 out]
              }
              frame True {
              }
            }
            n693 = feedback-in #21(w1179) -> ()
            n694 = feedback-in #22(w1172) -> ()
            n695 = Bundle(w1179, w1172) -> (w1169:cluster{dbl[], dbl[]})  [unwired: 1 in]
            n696 = Build Array(w1158, w1169) -> (→"XY Graph 3":cluster{dbl[], dbl[]}[])
          }
          frame 1026 {
            # "Pedalbox Brake"
            n697 = local read "BPS1_Raw"() -> (w1258:u16)
            n698 = local read "BPS2_Raw"() -> (w1257:u16)
            n699 = Index Array(array=w1262, index=2) -> (element=w1254:u8)
            n700 = Index Array(array=w1262, index=4) -> (element=w1248:u8)
            n701 = Index Array(array=w1262, index=6) -> (element=w1245:u8)
            n702 = Index Array(array=w1262, index=8) -> (element=w1251:u8)
            n703 = Index Array(array=w1262, index=3) -> (element=w1272:u8)
            n704 = Index Array(array=w1262, index=5) -> (element=w1265:u8)
            n705 = Index Array(array=w1262, index=7) -> (element=w1268:u8)
            n706 = Index Array(array=w1262, index=9) -> (element=w1271:u8)
            n707 = And(x=w1254, y=u8 15) -> (x .and. y?=w1253:u8)
            n708 = And(x=w1248, y=u8 15) -> (x .and. y?=w1247:u8)
            n709 = And(x=w1245, y=u8 15) -> (x .and. y?=w1244:u8)
            n710 = And(x=w1251, y=u8 15) -> (x .and. y?=w1250:u8)
            n711 = Join Numbers(hi=w1253, lo=w1272) -> ((hi.lo)=w1261:u16)
            n712 = Join Numbers(hi=w1247, lo=w1265) -> ((hi.lo)=w1260:u16)
            n713 = Join Numbers(hi=w1244, lo=w1268) -> ((hi.lo)=w1256:u16)
            n714 = Join Numbers(hi=w1250, lo=w1271) -> ((hi.lo)=w1259:u16)
            n715 = Bundle(w1261, w1260, "BPS1_Raw"=w1258, "BPS2_Raw"=w1257, w1256, w1259) -> ()  [unwired: 1 in, 1 out]
          }
          frame 1027 {
            # "Pedalbox Brake"
            n716 = Index Array(array=w1292, index=6) -> (element=w1290:u8)
            n717 = Index Array(array=w1292, index=7) -> (element=w1299:u8)
            n718 = Index Array(array=w1292, index=4) -> (element=w1287:u8)
            n719 = Index Array(array=w1292, index=5) -> (element=w1307:u8)
            n720 = Index Array(array=w1292, index=8) -> (element=w1284:u8)
            n721 = Index Array(array=w1292, index=9) -> (element=w1296:u8)
            n722 = Index Array(array=w1292, index=2) -> (element=w1281:u8)
            n723 = Index Array(array=w1292, index=3) -> (element=w1295:u8)
            n724 = And(x=w1290, y=u8 15) -> (x .and. y?=w1289:u8)
            n725 = And(x=w1287, y=u8 15) -> (x .and. y?=w1286:u8)
            n726 = And(x=w1284, y=u8 15) -> (x .and. y?=w1283:u8)
            n727 = And(x=w1281, y=u8 15) -> (x .and. y?=w1280:u8)
            n728 = Join Numbers(hi=w1289, lo=w1299) -> ()  [unwired: 1 out]
            n729 = Join Numbers(hi=w1286, lo=w1307) -> ()  [unwired: 1 out]
            n730 = Join Numbers(hi=w1283, lo=w1296) -> ()  [unwired: 1 out]
            n731 = Join Numbers(hi=w1280, lo=w1295) -> ()  [unwired: 1 out]
          }
          frame 528 {
            # "HV Cell Values"
            # "HV Accumulator"
            n732 = Index Array(array=w1369, index=5) -> (element=w1368:u8)
            n733 = Index Array(array=w1369, index=6) -> (element=w1367:u8)
            n734 = Index Array(array=w1369, index=3) -> (element=w1349:u8)
            n735 = Join Numbers(hi=w1368, lo=w1367) -> ((hi.lo)=w1345:u16)
            n736 = Index Array(array=w1369, index=4) -> (element=w1375:u8)
            n737 = And(x=w1349, y=u8 127) -> (x .and. y?=w1347:u8)
            n738 = Join Numbers(hi=w1347, lo=w1375) -> ((hi.lo)=w1374:u16)
            n739 = Index Array(array=w1369, index=2) -> (element=w1350:u8)
            n740 = Divide(x=w1345, y=10.0) -> (x/y=w1346:dbl)
            n741 = Replace Array Subset(array=w1373, new element=w1374, index=w1350) -> (w1343:u16[])
            n742 = Replace Array Subset(array=w1366, new element=w1346, index=w1350) -> (w1320:dbl[])
            n743 = Array Subset(array=w1320, index=0, length=28) -> (→"Temp 1":dbl[])
            n744 = Array Subset(array=w1320, index=84, length=28) -> (→"Temp 4":dbl[])
            n745 = Array Subset(array=w1320, index=56, length=28) -> (→"Temp 3":dbl[])
            n746 = Array Subset(array=w1320, index=28, length=28) -> (→"Temp 2":dbl[])
            n747 = Array Subset(array=w1320, index=0, length=180) -> (w1323:dbl[])
            n748 = Array Subset(array=w1320, index=140, length=28) -> (→"Temp 6":dbl[])
            n749 = Array Subset(array=w1320, index=112, length=28) -> (→"Temp 5":dbl[])
            n750 = call "Stack.vi"("Array"=w1343) -> ("Min"=w1310:u16, "Max"=w1312:u16, "appended array"=w1342:u16[], "appended array 2"=w1339:u16[], "appended array 3"=w1338:u16[], "appended array 4"=w1337:u16[], "appended array 5"=w1340:u16[], "appended array 6"=w1341:u16[])  [unwired: 11 in]
            "Cell Min" <- w1310
            "Cell Max" <- w1312
            "HV Cell Voltage" <- w1310
            n751 = Greater?(x=w1312, y="HV Max Limit") -> (0:w1318:bool)
            n752 = Greater?(x="HV Min Limit", y=w1310) -> (0:w1316:bool)
            n753 = Or(x=w1318, y=w1316) -> (x .or. y?=w1315:bool)
            n754 = And(x=w1315, y="Enable HV alert") -> (x .and. y?=w1313:bool)
            n755 = call "alert.vi"("Turn on"=w1313) -> ()  [unwired: 3 in, 1 out]
            n756 = for {
              tunnel: [w1390] -> w1372 mode=indexing
              tunnel: w1342 -> [w1389] mode=indexing
              tunnel: w1339 -> [w1387] mode=indexing
              tunnel: [w1388] -> w1336 mode=indexing
              tunnel: w1338 -> [w1386] mode=indexing
              tunnel: [w1385] -> w1335 mode=indexing
              tunnel: w1337 -> [w1384] mode=indexing
              tunnel: w1340 -> [w1383] mode=indexing
              tunnel: w1341 -> [w1382] mode=indexing
              tunnel: [w1381] -> w1334 mode=indexing
              tunnel: [w1380] -> w1333 mode=indexing
              tunnel: [w1379] -> w1332 mode=indexing
              n757 = Bundle(w1389, w1389) -> (w1390:cluster{u16, u16})  [unwired: 1 in]
              n758 = Bundle(w1387, w1387) -> (w1388:cluster{u16, u16})  [unwired: 1 in]
              n759 = Bundle(w1386, w1386) -> (w1385:cluster{u16, u16})  [unwired: 1 in]
              n760 = Bundle(w1384, w1384) -> (w1381:cluster{u16, u16})  [unwired: 1 in]
              n761 = Bundle(w1383, w1383) -> (w1380:cluster{u16, u16})  [unwired: 1 in]
              n762 = Bundle(w1382, w1382) -> (w1379:cluster{u16, u16})  [unwired: 1 in]
            }
            "Stack 1" <- w1372
            "Stack 2" <- w1336
            "Stack 3" <- w1335
            "Stack 4" <- w1334
            "Stack 5" <- w1333
            "Stack 6" <- w1332
            n763 = Array Max & Min(array=w1323) -> (max value=w1325:dbl, min value=w1326:dbl)  [unwired: 2 out]
            "Temp Max" <- w1325
            n764 = Bundle(w1325, w1326) -> (→"HV Cell Temperature":cluster{dbl, dbl})  [unwired: 1 in]
          }
          frame 532 {
            # "HV Battery Status"
            # "HV Battery Status"
            n765 = local read "HV Current"() -> (w1424:dbl)
            "Current" <- w1424
            n766 = local read "HV Before"() -> (w1425:dbl)
            n767 = local read "Cell Min"() -> (w1420:u16)
            n768 = local read "HV After"() -> (w1426:dbl)
            n769 = local read "TCU RR"() -> (w1408:dbl)
            n770 = local read "TCU FL"() -> (w1415:dbl)
            n771 = local read "TCU FR"() -> (w1412:dbl)
            n772 = local read "TCU RL"() -> (w1410:dbl)
            n773 = Index Array(array=w1449, index=6) -> (element=w1431:u8)
            n774 = Index Array(array=w1449, index=7) -> (element=w1430:u8)
            n775 = Index Array(array=w1449, index=4) -> (element=w1457:u8)
            n776 = Index Array(array=w1449, index=5) -> (element=w1456:u8)
            n777 = Index Array(array=w1449, index=8) -> (element=w1451:u8)
            n778 = Index Array(array=w1449, index=9) -> (element=w1450:u8)
            n779 = Index Array(array=w1449, index=2) -> (element=w1466:u8)
            n780 = Index Array(array=w1449, index=3) -> (element=w1465:u8)
            n781 = Join Numbers(hi=w1457, lo=w1456) -> ((hi.lo)=w1443:u16)
            n782 = Join Numbers(hi=w1451, lo=w1450) -> ((hi.lo)=w1438:u16)
            n783 = Join Numbers(hi=w1466, lo=w1465) -> ((hi.lo)=w1446:u16)
            n784 = To Unsigned Byte Integer(number=w1431) -> (unsigned 8bit integer=w1432:u8)
            n785 = To Unsigned Byte Integer(number=w1430) -> (unsigned 8bit integer=w1433:u8)
            n786 = Bundle("HV Before"=w1425, "HV After"=w1426) -> (→"HV Voltage":cluster{"HV Before":dbl, "HV After":dbl})  [unwired: 1 in]
            n787 = local read "Cell Max"() -> (w1421:u16)
            n788 = local read "Actual Velocity \nRR [RPM]"() -> (w1409:i16)
            n789 = Compound Arithmetic op=MULTIPLY(w1425, w1424, 0.001 ("value")) -> (w1401:dbl)
            n790 = local read "Actual Velocity\nFR [RPM]"() -> (w1413:i16)
            n791 = local read "Actual Velocity\nRL [RPM]"() -> (w1411:i16)
            n792 = local read "Actual Velocity\nFL [RPM]"() -> (w1414:i16)
            n793 = Join Numbers(hi=w1432, lo=w1433) -> ((hi.lo)=w1429:u16)
            n794 = To Double Precision Float(number=w1443) -> (double precision float=w1444:dbl)
            n795 = To Double Precision Float(number=w1438) -> (double precision float=w1439:dbl)
            n796 = To Double Precision Float(number=w1446) -> (double precision float=w1447:dbl)
            n797 = Bundle("Cell Max"=w1421, "Cell Min"=w1420) -> (→"HV Cell":cluster{"Cell Max":u16, "Cell Min":u16})  [unwired: 1 in]
            n798 = Multiply(x=w1414, y=w1415) -> (x*y=w1419:dbl)
            n799 = Multiply(x=w1413, y=w1412) -> (x*y=w1418:dbl)
            n800 = Multiply(x=w1411, y=w1410) -> (x*y=w1417:dbl)
            n801 = Multiply(x=w1409, y=w1408) -> (x*y=w1416:dbl)
            n802 = To Word Integer(number=w1429) -> (16bit integer=w1428:i16)
            n803 = Divide(x=w1439, y=1.0) -> (x/y=→"SoC [mAh]":dbl)
            n804 = Divide(x=w1444, y=10.0) -> (x/y=→"HV After":dbl)
            n805 = Divide(x=w1447, y=10.0) -> (x/y=→"HV Before":dbl)
            n806 = Compound Arithmetic op=ADD(w1419, w1418, w1417, w1416) -> (w1407:dbl)
            n807 = To Double Precision Float(number=w1428) -> (double precision float=w1441:dbl)
            n808 = Divide(x=w1401, y=3.6) -> (x/y=w1393:dbl)
            n809 = Divide(x=w1441, y=10.0) -> (x/y=→"HV Current":dbl)
            n810 = Multiply(x=0.005, y=w1393) -> (x*y=w1402:dbl)
            n811 = Compound Arithmetic op=MULTIPLY(w1407, 0.10472 ("x"), 0.0098 ("y"), 0.001 ("value")) -> (w1391:dbl)
            n812 = feedback #25() -> (w1397:dbl)  [unwired: 1 in]
            n813 = Add(x=w1397, y=w1402) -> (x+y=w1395:dbl)
            n814 = case shown="True" "New Lap" {
              tunnel: w1395 -> [w1469 _]
              tunnel: [w1469 0.0] -> w1394
              frame False {
              }
              frame True {
              }
            }
            n815 = feedback-in #25(w1394) -> ()
            n816 = Bundle(w1401, w1391) -> (→"Electric Power":cluster{dbl, dbl})  [unwired: 1 in]
            n817 = feedback #26() -> (w1398:dbl[])  [unwired: 1 in]
            n818 = case shown="False" "New Lap" {
              tunnel: w1395 -> [w1473 w1478]
              tunnel: [w1472 w1477] -> w1399
              tunnel: w1398 -> [w1471 w1476]
              frame False {
                n819 = Array Size(array=w1471) -> (size(s)=w1475:i32)
                n820 = Decrement(x=w1475) -> (x-1=w1474:i32)
                n821 = Replace Array Subset(array=w1471, new element=w1473, index=w1474) -> (w1472:dbl[])
              }
              frame True {
                n822 = Build Array (concatenate)(w1476, w1478) -> (w1477:dbl[])
              }
            }
            "Energy" <- w1399
            n823 = feedback-in #26(w1399) -> ()
          }
          frame 530 {
            # "ilyen nincs 18ban"
            # "ilyen nincs 18ban"
            # "ilyen nincs 18-ban"
            # "HV Accumulator Status"
            # "Accumulator Status"
            n824 = Index Array(array=w1502, index=3) -> (element=w1538:u8)
            n825 = Index Array(array=w1502, index=4) -> (element=w1528:u8)
            n826 = Index Array(array=w1502, index=5) -> (element=w1534:u8)
            n827 = Number To Boolean Array(number=w1538) -> (Boolean array=w1543:bool[])
            n828 = Number To Boolean Array(number=w1528) -> (Boolean array=w1527:bool[])
            n829 = Number To Boolean Array(number=w1534) -> (Boolean array=w1533:bool[])
            n830 = Index Array(array=w1543, index #1=7 ("index"), index #2=6 ("index"), index #3=5 ("index"), index #4=4 ("index"), index #5=3 ("index"), index #6=2 ("index"), index #7=1 ("index"), index #8=0 ("index")) -> (element #1=→"AMS error":bool, element #2=→"IMD error":bool, element #3=→"HVDet" →"HVDet":bool, element #4=→"AIR+" →"SC AIR+" →"AIR+":bool, element #5=→"AIR-" →"SC AIR-" →"AIR-":bool, element #6=→"SC Endline":bool, element #7=→"PC State" →"PC State 2":bool, element #8=→"TSAL State" →"TSAL State 2":bool)
            n831 = Index Array(array=w1527, index #1=7 ("index"), index #2=6 ("index"), index #3=5 ("index"), index #4=4 ("index"), index #5=3 ("index"), index #6=2 ("index"), index #7=1 ("index"), index #8=0 ("index")) -> (element #1=→"12V State" →"Driver Protection" →"SC 12V":bool, element #2=→"HV_ACC in menu":bool, element #3=→"TSAL Green":bool, element #4=→"AMS Relay" →"SC AMS" →"AMS Relay 2":bool, element #5=→"IMD Relay" →"SC IMD" →"IMD Relay":bool, element #6=→"TSAL Red":bool, element #7=w1483:bool, element #8=→"MCU HVDET":bool)
            n832 = Index Array(array=w1533, index #1=7 ("index"), index #2=6 ("index"), index #3=5 ("index"), index #4=4 ("index"), index #5=3 ("index"), index #6=2 ("index"), index #7=1 ("index"), index #8=0 ("index")) -> (element #1=→"TS-OC":bool, element #2=→"PC":bool, element #5=→"TS-OV":bool, element #6=→"OT":bool, element #7=→"OV":bool, element #8=→"UV":bool)  [unwired: 2 out]
            n833 = Not(x=w1483) -> (.not. x?=→"TSAL Error":bool)
            n834 = Index Array(array=w1502, index=7) -> (element=w1518:u8)
            n835 = Index Array(array=w1502, index=8) -> (element=w1517:u8)
            n836 = Index Array(array=w1502, index=6) -> (element=→"Place of Error":u8)
            n837 = Join Numbers(hi=w1518, lo=w1517) -> ((hi.lo)=→"Value":u16)
          }
          frame 560 {
            n838 = local read "BrakeRaw"() -> (w1576:u16)
            n839 = local read "BPFV"() -> (w1561:bool)
            n840 = local read "BPFSV"() -> (w1560:bool)
            n841 = Index Array(array=w1594, index=4) -> (element=w1567:u8)
            n842 = Index Array(array=w1594, index=2) -> (element=w1579:u8)
            n843 = Index Array(array=w1594, index=6) -> (element=w1585:u8)
            n844 = Index Array(array=w1594, index=8) -> (element=w1574:u8)
            n845 = Index Array(array=w1594, index=9) -> (element=w1593:u8)
            n846 = And(x=w1567, y=u8 15) -> (x .and. y?=w1568:u8)
            n847 = And(x=w1579, y=u8 15) -> (x .and. y?=w1582:u8)
            n848 = And(x=w1585, y=u8 15) -> (x .and. y?=w1584:u8)
            n849 = And(x=w1574, y=u8 15) -> (x .and. y?=w1573:u8)
            n850 = And(x=w1567, y=u8 240) -> (x .and. y?=w1570:u8)
            n851 = And(x=w1579, y=u8 240) -> (x .and. y?=w1580:u8)
            n852 = Join Numbers(hi=w1573, lo=w1593) -> ((hi.lo)=w1549:u16)
            "STA2_Raw" <- w1549
            n853 = Index Array(array=w1594, index=5) -> (element=w1603:u8)
            n854 = Index Array(array=w1594, index=7) -> (element=w1598:u8)
            n855 = Index Array(array=w1594, index=3) -> (element=w1610:u8)
            n856 = To Unsigned Byte Integer(number=w1568) -> (unsigned 8bit integer=w1604:u8)
            n857 = To Unsigned Byte Integer(number=w1582) -> (unsigned 8bit integer=w1609:u8)
            n858 = To Unsigned Byte Integer(number=w1584) -> (unsigned 8bit integer=w1599:u8)
            n859 = Number To Boolean Array(number=w1570) -> (Boolean array=w1587:bool[])
            n860 = Number To Boolean Array(number=w1580) -> (Boolean array=w1592:bool[])
            n861 = Join Numbers(hi=w1599, lo=w1598) -> ((hi.lo)=w1572:u16)
            n862 = Join Numbers(hi=w1604, lo=w1603) -> ((hi.lo)=→"APPS2" →"Apps2":u16)
            n863 = Join Numbers(hi=w1609, lo=w1610) -> ((hi.lo)=w1577:u16)
            "APPS1" <- w1577
            "Apps1" <- w1577
            "TorqRaw" <- w1577
            n864 = Index Array(array=w1587, index #1=7, index #2=6) -> (element #1=w1563:bool, element #2=w1562:bool)
            "STA1" <- w1563
            "STA2" <- w1562
            n865 = Index Array(array=w1592, index #1=6, index #2=7) -> (element #1=w1565:bool, element #2=w1564:bool)
            "TPS1V" <- w1565
            "TPS2V" <- w1564
            n866 = To Double Precision Float(number=w1572) -> (double precision float=w1548:dbl)
            "STA1_Raw" <- w1548
            n867 = local read "BPFV"() -> (w1559:bool)
            n868 = local read "BPRV"() -> (w1558:bool)
            n869 = Subtract(x=w1548, y=w1549) -> (x-y=w1557:dbl)
            n870 = Build Array(w1565, w1564, w1563, w1562, w1561, w1560, w1559, w1558) -> (→"Sensor Check":bool[])
            n871 = To Double Precision Float(number=w1577) -> (double precision float=w1607:dbl)
            n872 = Bundle(w1577, "BrakeRaw"=w1576) -> (→"Pedal Signals":cluster{u16, "BrakeRaw":u16})  [unwired: 1 in]
            n873 = feedback-in #27(w1557) -> ()
            n874 = feedback #27() -> (w1556:dbl)  [unwired: 1 in]
            n875 = feedback #28() -> (w1555:dbl)  [unwired: 1 in]
            n876 = feedback-in #28(w1556) -> ()
            n877 = feedback #29() -> (w1554:dbl)  [unwired: 1 in]
            n878 = feedback-in #29(w1555) -> ()
            n879 = feedback #30() -> (w1553:dbl)  [unwired: 1 in]
            n880 = feedback-in #30(w1554) -> ()
            n881 = Compound Arithmetic op=ADD(w1557, w1556, w1555, w1554, w1553) -> (w1552:dbl)
            n882 = Multiply(x=0.1, y=w1607) -> (x*y=→"Torque":dbl)
            n883 = Divide(x=w1552, y=10.0) -> (x/y=→"Steering Angle":dbl)
          }
          frame 561 {
            w1652 = 0
            w1655 = 4
            w1643 = 5
            w1642 = 6
            w1639 = 7
            n884 = Index Array(array=w1624, index=w1655) -> (element=w1654:u8)
            n885 = Index Array(array=w1624, index=w1639) -> ()  [unwired: 1 out]
            n886 = Index Array(array=w1624, index=w1642) -> (element=w1645:u8)
            n887 = Index Array(array=w1624, index=2) -> (element=w1636:u8)
            n888 = Index Array(array=w1624, index=6) -> (element=w1618:u8)
            n889 = Index Array(array=w1624, index=8) -> (element=w1619:u8)
            n890 = Index Array(array=w1624, index=3) -> (element=w1658:u8)
            n891 = Index Array(array=w1624, index=7) -> (element=w1630:u8)
            n892 = Index Array(array=w1624, index=9) -> (element=w1625:u8)
            n893 = Split Number(x=w1636) -> (lo(x)=w1657:u8)  [unwired: 1 out]
            n894 = Split Number(x=w1654) -> (lo(x)=w1653:u8)  [unwired: 1 out]
            n895 = And(x=w1636, y=u8 15) -> (x .and. y?=w1635:u8)
            n896 = And(x=w1618, y=u8 15) -> (x .and. y?=w1631:u8)
            n897 = And(x=w1619, y=u8 15) -> (x .and. y?=w1626:u8)
            n898 = Number To Boolean Array(number=w1636) -> (Boolean array=w1667:bool[])
            n899 = Number To Boolean Array(number=w1619) -> (Boolean array=w1640:bool[])
            n900 = Number To Boolean Array(number=w1645) -> (Boolean array=w1644:bool[])
            n901 = Index Array(array=w1640, index=w1639) -> (element=→"BPRV":bool)
            n902 = Index Array(array=w1644, index=w1639) -> (element=→"BPFV":bool)
            n903 = Join Numbers(hi=w1652, lo=w1657) -> ((hi.lo)=w1656:u64)
            n904 = Join Numbers(hi=w1652, lo=w1653) -> ((hi.lo)=w1651:u64)
            n905 = Join Numbers(hi=w1631, lo=w1630) -> ((hi.lo)=w1623:u16)
            "BP_front" <- w1623
            n906 = Join Numbers(hi=w1626, lo=w1625) -> ((hi.lo)=w1622:u16)
            "BP_rear" <- w1622
            n907 = Index Array(array=w1667, index #1=w1639, index #2=w1642, index #3=w1643, index #4=w1655) -> (element #1=→"Brake Heartbeat":bool, element #2=→"BPFV":bool, element #3=→"BPFSV":bool, element #4=→"Braking":bool)
            n908 = Join Numbers(hi=w1635, lo=w1658) -> ((hi.lo)=→"Brake Encoder" →"Brake Pedal Force" →"BrakeRaw":u16)
            n909 = To Unsigned Byte Integer(number=w1656) -> ()  [unwired: 1 out]
            n910 = Index Array(array=w1624, index=w1643) -> (element=w1649:u8)
            n911 = Bundle(w1623, w1622) -> (→"Front / Rear Brake Pressure":cluster{u16, u16})  [unwired: 1 in]
            n912 = To Unsigned Byte Integer(number=w1651) -> (unsigned 8bit integer=w1650:u8)
            n913 = Join Numbers(hi=w1650, lo=w1649) -> ((hi.lo)=→"Brake Pedal Fore Supply":u16)
          }
          frame 644 {
            # "MCU FL"
            n914 = Index Array(array=w1671, index=5) -> (element=w1702:u8)
            n915 = Index Array(array=w1671, index=4) -> (element=w1701:u8)
            n916 = Index Array(array=w1671, index=7) -> (element=w1687:u8)
            n917 = Index Array(array=w1671, index=6) -> (element=w1686:u8)
            n918 = Index Array(array=w1671, index=9) -> (element=w1693:u8)
            n919 = Index Array(array=w1671, index=8) -> (element=w1692:u8)
            n920 = Index Array(array=w1671, index=3) -> (element=w1670:u8)
            n921 = Join Numbers(hi=w1702, lo=w1701) -> ((hi.lo)=w1691:u16)
            n922 = Join Numbers(hi=w1687, lo=w1686) -> ((hi.lo)=w1679:u16)
            n923 = Join Numbers(hi=w1693, lo=w1692) -> ((hi.lo)=w1677:u16)
            n924 = Number To Boolean Array(number=w1670) -> (Boolean array=→"Status FL":bool[])
            n925 = To Word Integer(number=w1691) -> (16bit integer=→"Actual Velocity\nFL [RPM]":i16)
            n926 = To Word Integer(number=w1679) -> (16bit integer=w1678:i16)
            n927 = To Word Integer(number=w1677) -> (16bit integer=w1676:i16)
            n928 = Multiply(x=w1678, y=105.0) -> (x*y=w1685:dbl)
            n929 = Multiply(x=w1676, y=105.0) -> (x*y=w1680:dbl)
            n930 = Divide(x=w1685, y=16384.0) -> (x/y=w1675:dbl)
            "Id FL [A]" <- w1675
            n931 = Divide(x=w1680, y=16384.0) -> (x/y=w1674:dbl)
            "Iq FL [A]" <- w1674
            n932 = Bundle(w1675, w1674) -> (→"MCU FL":cluster{dbl, dbl})  [unwired: 1 in]
          }
          frame 645 {
            # "MCU FR"
            n933 = Index Array(array=w1705, index=5) -> (element=w1738:u8)
            n934 = Index Array(array=w1705, index=4) -> (element=w1737:u8)
            n935 = Index Array(array=w1705, index=7) -> (element=w1723:u8)
            n936 = Index Array(array=w1705, index=6) -> (element=w1722:u8)
            n937 = Index Array(array=w1705, index=3) -> (element=w1707:u8)
            n938 = Index Array(array=w1705, index=9) -> (element=w1729:u8)
            n939 = Index Array(array=w1705, index=8) -> (element=w1728:u8)
            n940 = Join Numbers(hi=w1738, lo=w1737) -> ((hi.lo)=w1727:u16)
            n941 = Join Numbers(hi=w1723, lo=w1722) -> ((hi.lo)=w1715:u16)
            n942 = Join Numbers(hi=w1729, lo=w1728) -> ((hi.lo)=w1713:u16)
            n943 = Number To Boolean Array(number=w1707) -> (Boolean array=→"Status FR":bool[])
            n944 = To Word Integer(number=w1727) -> (16bit integer=→"Actual Velocity\nFR [RPM]":i16)
            n945 = To Word Integer(number=w1715) -> (16bit integer=w1714:i16)
            n946 = To Word Integer(number=w1713) -> (16bit integer=w1712:i16)
            n947 = Multiply(x=w1714, y=105.0) -> (x*y=w1721:dbl)
            n948 = Multiply(x=w1712, y=105.0) -> (x*y=w1716:dbl)
            n949 = Divide(x=w1721, y=16384.0) -> (x/y=w1711:dbl)
            "Id FR [A]" <- w1711
            n950 = Divide(x=w1716, y=16384.0) -> (x/y=w1710:dbl)
            "Iq FR [A]" <- w1710
            n951 = Bundle(w1711, w1710) -> (→"MCU FR":cluster{dbl, dbl})  [unwired: 1 in]
          }
          frame 646 {
            # "MCU FL"
            n952 = Index Array(array=w1748, index=5) -> (element=w1759:u8)
            n953 = Index Array(array=w1748, index=4) -> (element=w1758:u8)
            n954 = Index Array(array=w1748, index=7) -> (element=w1764:u8)
            n955 = Index Array(array=w1748, index=6) -> (element=w1763:u8)
            n956 = Index Array(array=w1748, index=9) -> (element=w1745:u8)
            n957 = Index Array(array=w1748, index=8) -> (element=w1744:u8)
            n958 = Index Array(array=w1748, index=3) -> (element=w1773:u8)
            n959 = Index Array(array=w1748, index=2) -> (element=w1772:u8)
            n960 = Join Numbers(hi=w1759, lo=w1758) -> ((hi.lo)=w1757:u16)
            n961 = Join Numbers(hi=w1764, lo=w1763) -> ((hi.lo)=w1750:u16)
            n962 = Join Numbers(hi=w1745, lo=w1744) -> ((hi.lo)=w1743:u16)
            n963 = Join Numbers(hi=w1773, lo=w1772) -> ((hi.lo)=w1762:u16)
            n964 = To Word Integer(number=w1757) -> (16bit integer=w1752:i16)
            n965 = To Unsigned Word Integer(number=w1750) -> (unsigned 16bit integer=→"Error Info FL":u16)
            n966 = To Word Integer(number=w1762) -> (16bit integer=w1755:i16)
            n967 = Divide(x=w1743, y=10.0) -> (x/y=→"IGBT FL TEMP":dbl)
            n968 = Divide(x=w1752, y=10.0) -> (x/y=→"T Inv. FL [°C]":dbl)
            n969 = Divide(x=w1755, y=10.0) -> (x/y=→"T Motor FL [°C]":dbl)
          }
          frame 647 {
            # "MCU FR"
            n970 = Index Array(array=w1777, index=5) -> (element=w1794:u8)
            n971 = Index Array(array=w1777, index=4) -> (element=w1793:u8)
            n972 = Index Array(array=w1777, index=7) -> (element=w1799:u8)
            n973 = Index Array(array=w1777, index=6) -> (element=w1798:u8)
            n974 = Index Array(array=w1777, index=9) -> (element=w1781:u8)
            n975 = Index Array(array=w1777, index=8) -> (element=w1780:u8)
            n976 = Index Array(array=w1777, index=3) -> (element=w1808:u8)
            n977 = Index Array(array=w1777, index=2) -> (element=w1807:u8)
            n978 = Join Numbers(hi=w1794, lo=w1793) -> ((hi.lo)=w1792:u16)
            n979 = Join Numbers(hi=w1799, lo=w1798) -> ((hi.lo)=w1785:u16)
            n980 = Join Numbers(hi=w1781, lo=w1780) -> ((hi.lo)=w1779:u16)
            n981 = Join Numbers(hi=w1808, lo=w1807) -> ((hi.lo)=w1797:u16)
            n982 = To Word Integer(number=w1792) -> (16bit integer=w1787:i16)
            n983 = To Unsigned Word Integer(number=w1785) -> (unsigned 16bit integer=→"Error Info FR":u16)
            n984 = To Word Integer(number=w1797) -> (16bit integer=w1790:i16)
            n985 = Divide(x=w1779, y=10.0) -> (x/y=→"IGBT FR TEMP":dbl)
            n986 = Divide(x=w1787, y=10.0) -> (x/y=→"T Inv. FR [°C]":dbl)
            n987 = Divide(x=w1790, y=10.0) -> (x/y=→"T Motor FR [°C]":dbl)
          }
          frame 648 {
            # "MCU RL"
            n988 = Index Array(array=w1811, index=5) -> (element=w1844:u8)
            n989 = Index Array(array=w1811, index=4) -> (element=w1843:u8)
            n990 = Index Array(array=w1811, index=7) -> (element=w1829:u8)
            n991 = Index Array(array=w1811, index=6) -> (element=w1828:u8)
            n992 = Index Array(array=w1811, index=3) -> (element=w1813:u8)
            n993 = Index Array(array=w1811, index=9) -> (element=w1835:u8)
            n994 = Index Array(array=w1811, index=8) -> (element=w1834:u8)
            n995 = Join Numbers(hi=w1844, lo=w1843) -> ((hi.lo)=w1833:u16)
            n996 = Join Numbers(hi=w1829, lo=w1828) -> ((hi.lo)=w1821:u16)
            n997 = Join Numbers(hi=w1835, lo=w1834) -> ((hi.lo)=w1819:u16)
            n998 = Number To Boolean Array(number=w1813) -> (Boolean array=→"Status RL":bool[])
            n999 = To Word Integer(number=w1833) -> (16bit integer=→"Actual Velocity\nRL [RPM]":i16)
            n1000 = To Word Integer(number=w1821) -> (16bit integer=w1820:i16)
            n1001 = To Word Integer(number=w1819) -> (16bit integer=w1818:i16)
            n1002 = Multiply(x=w1820, y=105.0) -> (x*y=w1827:dbl)
            n1003 = Multiply(x=w1818, y=105.0) -> (x*y=w1822:dbl)
            n1004 = Divide(x=w1827, y=16384.0) -> (x/y=w1816:dbl)
            "Id RL [A]" <- w1816
            n1005 = Divide(x=w1822, y=16384.0) -> (x/y=w1815:dbl)
            "Iq RL [A]" <- w1815
            n1006 = Bundle(w1816, w1815) -> (→"MCU RL":cluster{dbl, dbl})  [unwired: 1 in]
          }
          frame 649 {
            w1848 = 3.6 ("y")
            # "MCU RR"
            n1007 = local read "TCU_v"() -> (w1849:dbl)
            n1008 = local read "Id RR [A]"() -> (w1883:dbl)
            n1009 = local read "Id FL [A]"() -> (w1886:dbl)
            n1010 = local read "Id FR [A]"() -> (w1885:dbl)
            n1011 = local read "Id RL [A]"() -> (w1884:dbl)
            n1012 = local read "Vel_acc"() -> (w1876:dbl)
            n1013 = local read "Vel_acc"() -> (w1867:dbl)
            n1014 = flat-sequence {
              frame #0 {
                w1930 = i16 10 ("y")
                w1952 = 15.6 ("y")
                n1015 = local read "Torq_sum"() -> (w1950:dbl)
                n1016 = Multiply(x=w1950, y=w1952) -> (x*y=→"Torque [Nm]":dbl)
                n1017 = local read "Actual Velocity \nRR [RPM]"() -> (w1931:i16)
                n1018 = local read "Actual Velocity\nRL [RPM]"() -> (w1932:i16)
                n1019 = local read "Actual Velocity\nFR [RPM]"() -> (w1933:i16)
                n1020 = local read "Actual Velocity\nFL [RPM]"() -> (w1934:i16)
                n1021 = Less?(x=w1932, y=w1930) -> (x < y?=w1936:bool)
                n1022 = Less?(x=w1931, y=w1930) -> (x < y?=w1935:bool)
                n1023 = Less?(x=w1934, y=w1930) -> (x < y?=w1938:bool)
                n1024 = Less?(x=w1933, y=w1930) -> (x < y?=w1937:bool)
                n1025 = To Double Precision Float(number=w1932) -> (double precision float=w1945:dbl)
                n1026 = To Double Precision Float(number=w1931) -> (double precision float=w1944:dbl)
                n1027 = Add(x=w1945, y=w1944) -> (x+y=w1947:dbl)
                n1028 = feedback #31() -> (w1942:dbl)  [unwired: 1 in]
                n1029 = local read "START"() -> (w1928:bool)
                n1030 = Compound Arithmetic op=AND(w1928, w1938, w1937, w1936, w1935) -> (→"IsStopped":bool)
                n1031 = Divide(x=w1947, y=2.0) -> (x/y=w1941:dbl)
                n1032 = formula code="y_=a*x+(1-a)*y;"("x"=w1941, "y"=w1942, "a"=0.1 ("input variable")) -> ("y_"=w1940:dbl)
                n1033 = feedback-in #31(w1940) -> ()
                n1034 = Multiply(x=w1940, y=0.104719755) -> (x*y=w1955:dbl)
                n1035 = Multiply(x=w1955, y=0.227) -> (x*y=w1949:dbl)
                n1036 = Divide(x=w1949, y=w1952) -> (x/y=w1948:dbl)
                n1037 = Multiply(x=w1948, y=3.6) -> (x*y=→"Velocity [km/h]":dbl)
              }
            }
            n1038 = Multiply(x=w1848, y=w1849) -> (x*y=w1847:dbl)
            n1039 = Index Array(array=w1892, index=5) -> (element=w1925:u8)
            n1040 = Index Array(array=w1892, index=4) -> (element=w1924:u8)
            n1041 = Index Array(array=w1892, index=7) -> (element=w1910:u8)
            n1042 = Index Array(array=w1892, index=6) -> (element=w1909:u8)
            n1043 = Index Array(array=w1892, index=3) -> (element=w1894:u8)
            n1044 = Index Array(array=w1892, index=9) -> (element=w1916:u8)
            n1045 = Index Array(array=w1892, index=8) -> (element=w1915:u8)
            n1046 = Divide(x=w1867, y=0.227) -> (x/y=w1865:dbl)
            n1047 = Multiply(x=w1876, y=w1848) -> (x*y=w1877:dbl)
            n1048 = Join Numbers(hi=w1925, lo=w1924) -> ((hi.lo)=w1914:u16)
            n1049 = Join Numbers(hi=w1910, lo=w1909) -> ((hi.lo)=w1902:u16)
            n1050 = Join Numbers(hi=w1916, lo=w1915) -> ((hi.lo)=w1900:u16)
            n1051 = Build Array(w1886, w1885, w1884, w1883) -> (w1882:dbl[])
            n1052 = local read "Velocity [km/h]"() -> (w1879:dbl)
            n1053 = Number To Boolean Array(number=w1894) -> (Boolean array=→"Status RR":bool[])
            n1054 = local read "Actual Velocity \nRR [RPM]"() -> (w1888:i16)
            n1055 = local read "Actual Velocity \nRR [RPM]"() -> (w1875:i16)
            n1056 = local read "Actual Velocity\nFR [RPM]"() -> (w1890:i16)
            n1057 = local read "Actual Velocity\nRL [RPM]"() -> (w1889:i16)
            n1058 = local read "Actual Velocity\nFR [RPM]"() -> (w1873:i16)
            n1059 = local read "Actual Velocity\nRL [RPM]"() -> (w1874:i16)
            n1060 = local read "Actual Velocity\nFL [RPM]"() -> (w1891:i16)
            n1061 = local read "Actual Velocity\nFL [RPM]"() -> (w1872:i16)
            n1062 = To Word Integer(number=w1914) -> (16bit integer=→"Actual Velocity \nRR [RPM]":i16)
            n1063 = To Word Integer(number=w1902) -> (16bit integer=w1901:i16)
            n1064 = To Word Integer(number=w1900) -> (16bit integer=w1899:i16)
            n1065 = call "Curr2Torq.vi"("Current"=w1882) -> ("Torque"=w1881:dbl[])
            n1066 = Bundle("Actual Velocity\nFL [RPM]"=w1891, "Actual Velocity\nFR [RPM]"=w1890, "Actual Velocity\nRL [RPM]"=w1889, "Actual Velocity \nRR [RPM]"=w1888) -> (→"Angular Speed":T18)  [unwired: 1 in]
            n1067 = Add Array Elements(numeric array=w1881) -> (sum=w1880:dbl)
            "Torq_sum" <- w1880
            n1068 = To Double Precision Float(number=w1872) -> (double precision float=w1871:dbl)
            n1069 = To Double Precision Float(number=w1873) -> (double precision float=w1870:dbl)
            n1070 = To Double Precision Float(number=w1874) -> (double precision float=w1869:dbl)
            n1071 = To Double Precision Float(number=w1875) -> (double precision float=w1868:dbl)
            n1072 = Multiply(x=w1901, y=105.0) -> (x*y=w1908:dbl)
            n1073 = Multiply(x=w1899, y=105.0) -> (x*y=w1903:dbl)
            n1074 = Multiply(x=15.6, y=w1865) -> (x*y=w1851:dbl)
            n1075 = Divide(x=w1908, y=16384.0) -> (x/y=w1898:dbl)
            "Id RR [A]" <- w1898
            n1076 = Divide(x=w1903, y=16384.0) -> (x/y=w1897:dbl)
            "Iq RR [A]" <- w1897
            n1077 = Multiply(x=30.0, y=w1851) -> (x*y=w1863:dbl)
            n1078 = Bundle("Velocity [km/h]"=w1879, "Torque"=w1880, w1877, w1847) -> (→"?":T5)  [unwired: 1 in]
            n1079 = Divide(x=w1863, y=3.141592653589793) -> (x/y=w1857:dbl)
            n1080 = Subtract(x=w1871, y=w1857) -> (x-y=w1861:dbl)
            n1081 = Subtract(x=w1870, y=w1857) -> (x-y=w1860:dbl)
            n1082 = Subtract(x=w1869, y=w1857) -> (x-y=w1859:dbl)
            n1083 = Subtract(x=w1868, y=w1857) -> (x-y=w1858:dbl)
            n1084 = Divide(x=w1861, y=w1857) -> (x/y=w1856:dbl)
            n1085 = Divide(x=w1860, y=w1857) -> (x/y=w1855:dbl)
            n1086 = Divide(x=w1859, y=w1857) -> (x/y=w1854:dbl)
            n1087 = Divide(x=w1858, y=w1857) -> (x/y=w1853:dbl)
            n1088 = Bundle(w1898, w1897) -> (→"MCU RR":cluster{dbl, dbl})  [unwired: 1 in]
            n1089 = Bundle(w1856, w1855, w1854, w1853) -> (→"Slip":cluster{dbl, dbl, dbl, dbl})  [unwired: 1 in]
          }
          frame 650 {
            # "MCU RL"
            n1090 = Index Array(array=w1958, index=5) -> (element=w1975:u8)
            n1091 = Index Array(array=w1958, index=4) -> (element=w1974:u8)
            n1092 = Index Array(array=w1958, index=7) -> (element=w1980:u8)
            n1093 = Index Array(array=w1958, index=6) -> (element=w1979:u8)
            n1094 = Index Array(array=w1958, index=9) -> (element=w1962:u8)
            n1095 = Index Array(array=w1958, index=8) -> (element=w1961:u8)
            n1096 = Index Array(array=w1958, index=3) -> (element=w1989:u8)
            n1097 = Index Array(array=w1958, index=2) -> (element=w1988:u8)
            n1098 = Join Numbers(hi=w1975, lo=w1974) -> ((hi.lo)=w1973:u16)
            n1099 = Join Numbers(hi=w1980, lo=w1979) -> ((hi.lo)=w1966:u16)
            n1100 = Join Numbers(hi=w1962, lo=w1961) -> ((hi.lo)=w1960:u16)
            n1101 = Join Numbers(hi=w1989, lo=w1988) -> ((hi.lo)=w1978:u16)
            n1102 = To Word Integer(number=w1973) -> (16bit integer=w1968:i16)
            n1103 = To Unsigned Word Integer(number=w1966) -> (unsigned 16bit integer=→"Error Info RL":u16)
            n1104 = To Word Integer(number=w1978) -> (16bit integer=w1971:i16)
            n1105 = Divide(x=w1960, y=10.0) -> (x/y=→"IGBT RL TEMP":dbl)
            n1106 = Divide(x=w1968, y=10.0) -> (x/y=→"T Inv. RL [°C]":dbl)
            n1107 = Divide(x=w1971, y=10.0) -> (x/y=→"T Motor RL [°C]":dbl)
          }
          frame 651 {
            # "MCU RR"
            n1108 = Index Array(array=w1993, index=5) -> (element=w2010:u8)
            n1109 = Index Array(array=w1993, index=4) -> (element=w2009:u8)
            n1110 = Index Array(array=w1993, index=7) -> (element=w2015:u8)
            n1111 = Index Array(array=w1993, index=6) -> (element=w2014:u8)
            n1112 = Index Array(array=w1993, index=9) -> (element=w1997:u8)
            n1113 = Index Array(array=w1993, index=8) -> (element=w1996:u8)
            n1114 = Index Array(array=w1993, index=3) -> (element=w2024:u8)
            n1115 = Index Array(array=w1993, index=2) -> (element=w2023:u8)
            n1116 = Join Numbers(hi=w2010, lo=w2009) -> ((hi.lo)=w2008:u16)
            n1117 = Join Numbers(hi=w2015, lo=w2014) -> ((hi.lo)=w2001:u16)
            n1118 = Join Numbers(hi=w1997, lo=w1996) -> ((hi.lo)=w1995:u16)
            n1119 = Join Numbers(hi=w2024, lo=w2023) -> ((hi.lo)=w2013:u16)
            n1120 = To Word Integer(number=w2008) -> (16bit integer=w2003:i16)
            n1121 = To Unsigned Word Integer(number=w2001) -> (unsigned 16bit integer=→"Error Info RR":u16)
            n1122 = To Word Integer(number=w2013) -> (16bit integer=w2006:i16)
            n1123 = Divide(x=w1995, y=10.0) -> (x/y=→"IGBT RR TEMP":dbl)
            n1124 = Divide(x=w2003, y=10.0) -> (x/y=→"T Inv. RR [°C]":dbl)
            n1125 = Divide(x=w2006, y=10.0) -> (x/y=→"T Motor RR [°C]":dbl)
          }
          frame 656 {
            n1126 = Index Array(array=w2064, index=5) -> (element=w2057:u8)
            n1127 = Index Array(array=w2064, index=4) -> (element=w2055:u8)
            n1128 = Index Array(array=w2064, index=3) -> (element=w2048:u8)
            n1129 = And(x=w2057, y=u8 15) -> (x .and. y?=→"Dial 5":u8)
            n1130 = And(x=w2048, y=u8 15) -> (x .and. y?=→"Dial":u8)
            n1131 = And(x=w2057, y=u8 240) -> (x .and. y?=w2052:u8)
            n1132 = And(x=w2055, y=u8 240) -> (x .and. y?=w2054:u8)
            n1133 = And(x=w2048, y=u8 240) -> (x .and. y?=w2047:u8)
            n1134 = And(x=w2055, y=u8 15) -> (x .and. y?=w2030:u8)
            "Dial 3" <- w2030
            n1135 = Logical Shift(y=i16 -4, x=w2052) -> (x << y=→"Dial 4":u8)
            n1136 = Logical Shift(y=i16 -4, x=w2047) -> (x << y=w2042:u8)
            n1137 = Logical Shift(y=i16 -4, x=w2054) -> (x << y=w2027:u8)
            "Dial 2" <- w2027
            n1138 = Multiply(x=4.16666, y=w2030) -> (x*y=→"Slope":dbl)
            n1139 = Number To Boolean Array(number=w2042) -> (Boolean array=w2041:bool[])
            n1140 = formula code="if(in1==1) out1=1;\nif(in1==2) out1=0.95;\nif(in1==3) out1=0.9;\nif(in1==4) out1=0.85;\nif(in1==5) out1=0.8;\nif(in1==6) out1=0.75;\nif(in1==7) out1=0.7;\nif(in1==8) out1=0.65;\nif(in1==9) out1=0.6;\nif(in1==10) out1=0.55;\nif(in1==11) out1=0.5;\nif(in1==12) out1=0.4;"("in1"=w2027) -> ()  [unwired: 1 out]
            n1141 = Index Array(array=w2041, index #1=0 ("index"), index #2=1 ("index"), index #3=2 ("index"), index #4=3 ("index")) -> (element #1=→"Boolean":bool, element #2=→"Boolean 2":bool, element #3=→"Boolean 3":bool, element #4=→"Boolean 4":bool)
          }
          frame 657 {
            n1142 = Index Array(array=w2073, index=3) -> (element=w2069:u8)
            n1143 = Index Array(array=w2073, index=2) -> (element=w2070:u8)
            n1144 = Join Numbers(hi=w2070, lo=w2069) -> ((hi.lo)=→"Brake Force" →"Brake Force":u16)
          }
          frame 642 {
            n1145 = Index Array(array=w2084, index=3) -> (element=w2128:u8)
            n1146 = Index Array(array=w2084, index #1=4 ("index"), index #2=5 ("index"), index #3=6 ("index"), index #4=7 ("index")) -> (element #1=w2097:u8, element #2=w2093:u8, element #3=w2092:u8, element #4=w2091:u8)
            n1147 = Index Array(array=w2084, index=2) -> (element=w2129:u8)
            n1148 = Number To Boolean Array(number=w2129) -> (Boolean array=w2127:bool[])
            n1149 = Number To Boolean Array(number=w2128) -> (Boolean array=w2110:bool[])
            n1150 = Join Numbers(hi=w2093, lo=w2097) -> ((hi.lo)=w2090:u16)
            n1151 = Join Numbers(hi=w2091, lo=w2092) -> ((hi.lo)=w2089:u16)
            n1152 = Join Numbers(hi=w2089, lo=w2090) -> ((hi.lo)=w2088:u32)
            n1153 = To Long Integer(number=w2088) -> (32bit integer=w2087:i32)
            n1154 = Divide(x=w2087, y=ext 1098.0) -> (x/y=→"Actual pos [°] Maxon":ext)
            n1155 = Index Array(array=w2127, index #1=0 ("index"), index #2=1 ("index"), index #3=2 ("index"), index #4=3 ("index"), index #5=4 ("index"), index #6=5 ("index"), index #7=6 ("index"), index #8=7 ("index")) -> (element #1=→"Ready to switch on":bool, element #2=→"Switched on":bool, element #3=→"Operation enable":bool, element #4=→"Fault present":bool, element #5=→"Voltage enabled":bool, element #7=→"Switch on disabled":bool, element #8=→"Warning present":bool)  [unwired: 1 out]
            n1156 = Index Array(array=w2110, index #1=0 ("index"), index #2=1 ("index"), index #3=2 ("index"), index #4=3 ("index"), index #5=4 ("index"), index #6=5 ("index"), index #7=6 ("index"), index #8=7 ("index")) -> (element #2=→"In operational NMT state":bool, element #3=→"Target reached":bool, element #5=→"Setpoint ack":bool, element #6=→"Following error":bool, element #8=→"Position referenced to home position":bool)  [unwired: 3 out]
          }
          frame 770 {
            n1157 = Index Array(array=w2145, index #1=4 ("index"), index #2=5 ("index"), index #3=6 ("index"), index #4=7 ("index")) -> (element #1=w2157:u8, element #2=w2153:u8, element #3=w2152:u8, element #4=w2151:u8)
            n1158 = Join Numbers(hi=w2153, lo=w2157) -> ((hi.lo)=w2150:u16)
            n1159 = Join Numbers(hi=w2151, lo=w2152) -> ((hi.lo)=w2149:u16)
            n1160 = Join Numbers(hi=w2149, lo=w2150) -> ((hi.lo)=w2148:u32)
            n1161 = To Long Integer(number=w2148) -> (32bit integer=w2146:i32)
            n1162 = Divide(x=w2146, y=ext 1098.0) -> (x/y=w2134:ext)
            n1163 = Equal To 0?(x=w2134) -> (x = 0?=w2136:bool)
            n1164 = local read "Actual pos [°] Maxon"() -> (w2137:ext)
            n1165 = feedback-in #32(w2134) -> ()
            n1166 = feedback #32() -> (w2135:ext)  [unwired: 1 in]
            n1167 = Select(t=w2135, s=w2136, f=w2134) -> (s? t:f=w2133:ext)
            "Target pos [°]" <- w2133
            n1168 = local read "Steering Angle"() -> (w2138:dbl)
            "Actual pos [°]" <- w2138
            n1169 = Bundle(w2133, "Steering Angle"=w2138, "Actual pos [°] Maxon"=w2137) -> (→"Steering Angle":T11)  [unwired: 1 in]
          }
          frame 787 {
            # "HV Critical Cell Values"
            n1170 = Index Array(array=w2162, index=4) -> (element=w2166:u8)
            n1171 = Index Array(array=w2162, index=3) -> (element=w2165:u8)
            n1172 = Index Array(array=w2162, index=5) -> (element=w2161:u8)
            n1173 = Index Array(array=w2162, index=6) -> (element=w2160:u8)
            n1174 = Join Numbers(hi=w2166, lo=w2165) -> ((hi.lo)=w2167:u16)
            n1175 = Join Numbers(hi=w2161, lo=w2160) -> ((hi.lo)=→"Temp Max 2":u16)
            n1176 = To Unsigned Word Integer(number=w2167) -> (unsigned 16bit integer=→"Cell Min 2":u16)
          }
          frame 800 {
            # "MCU Support Status kesz"
            n1177 = Index Array(array=w2181, index=3) -> (element=w2215:u8)
            n1178 = Index Array(array=w2181, index=5) -> (element=w2200:u8)
            n1179 = Index Array(array=w2181, index=6) -> (element=w2179:u8)
            n1180 = Index Array(array=w2181, index=4) -> (element=w2202:u8)
            n1181 = Number To Boolean Array(number=w2215) -> (Boolean array=w2224:bool[])
            n1182 = Number To Boolean Array(number=w2200) -> (Boolean array=w2199:bool[])
            n1183 = To Unsigned Word Integer(number=w2179) -> (unsigned 16bit integer=w2178:u16)
            "MCU S SC Endl" <- w2178
            n1184 = Number To Boolean Array(number=w2202) -> (Boolean array=w2203:bool[])
            n1185 = Greater?(x=w2178, y=5) -> ()  [unwired: 1 out]
            n1186 = Index Array(array=w2224, index #1=7 ("index"), index #2=6 ("index"), index #3=5 ("index"), index #4=4 ("index"), index #5=3 ("index"), index #6=2 ("index"), index #7=1 ("index"), index #8=0 ("index")) -> (element #1=→"Brake Light":bool, element #2=→"MCU EF":bool, element #3=→"MCU RF":bool, element #4=→"RTDS":bool, element #5=→"TCU Power":bool, element #6=→"24V front DC/DC":bool, element #7=→"24V rear DC/DC":bool, element #8=→"LKS & RKS" →"LKS & RKS" →"SC RKS" →"SC LKS":bool)
            n1187 = Index Array(array=w2203, index #1=7 ("index"), index #2=6 ("index"), index #3=5 ("index"), index #4=4 ("index"), index #5=3 ("index"), index #6=2 ("index"), index #7=1 ("index"), index #8=0 ("index")) -> (element #1=→"MCU Interlocks" →"MCU Interlock" →"SC Motor 4" →"SC Motor 1" →"SC Motor 3" →"SC MCU" →"SC Motor 2" →"Motor1 Interlock" →"Motor2 Interlock" →"Motor3 Interlock" →"Motor4 Interlock" →"HVD Interlock":bool, element #2=→"ON" →"ON":bool, element #3=→"START" →"START":bool, element #4=→"OFF" →"OFF":bool, element #5=→"Logging":bool, element #6=→"XBee CS":bool, element #7=→"Radio CS":bool, element #8=→"SD CS":bool)
            n1188 = Index Array(array=w2199, index=7) -> (element=→"TSAL":bool)
          }
          frame 816 {
            # "5db 12V"
            # "3db 48V"
            # "LV Sys Status"
            n1189 = Index Array(array=w2249, index=7) -> (element=w2277:u8)
            n1190 = Index Array(array=w2249, index=6) -> (element=w2317:u8)
            n1191 = Index Array(array=w2249, index=3) -> (element=w2334:u8)
            n1192 = Index Array(array=w2249, index=8) -> (element=w2247:u8)
            n1193 = Index Array(array=w2249, index=4) -> (element=w2291:u8)
            n1194 = Index Array(array=w2249, index=5) -> (element=w2288:u8)
            n1195 = Logical Shift(y=i16 -4, x=w2288) -> (x << y=w2306:u8)
            n1196 = Number To Boolean Array(number=w2277) -> (Boolean array=w2276:bool[])
            n1197 = Number To Boolean Array(number=w2317) -> (Boolean array=w2316:bool[])
            n1198 = Number To Boolean Array(number=w2334) -> (Boolean array=w2333:bool[])
            n1199 = Number To Boolean Array(number=w2247) -> (Boolean array=w2246:bool[])
            n1200 = Number To Boolean Array(number=w2291) -> (Boolean array=w2324:bool[])
            n1201 = Number To Boolean Array(number=w2288) -> (Boolean array=w2287:bool[])
            n1202 = Index Array(array=w2287, index #1=3, index #2=2, index #3=1, index #4=0) -> (element #1=→"Battery Full" →"Battery Full 2":bool, element #2=→"Overtemp. 3" →"Overtemp. 4":bool, element #3=→"Undervoltage 3" →"Undervoltage 4":bool, element #4=→"Battery Low" →"Battery Low 2":bool)
            n1203 = Index Array(array=w2324, index #1=7 ("index"), index #2=6 ("index"), index #3=5 ("index"), index #4=4 ("index"), index #5=3 ("index")) -> (element #1=→"48V Out 1" →"48V Out 1 2":bool, element #2=→"48V Out 2" →"48V Out 2 2":bool, element #3=→"48V Out 3" →"48V Out 3 2":bool, element #4=→"48V Out 4" →"48V Out 4 2":bool)  [unwired: 3 in, 4 out]
            n1204 = Index Array(array=w2276, index #1=7 ("index"), index #2=6 ("index"), index #3=5 ("index"), index #4=4 ("index"), index #5=3 ("index"), index #6=2 ("index"), index #7=1 ("index"), index #8=0 ("index")) -> (element #1=w2257:bool, element #2=w2256:bool, element #3=w2255:bool, element #4=w2252:bool, element #5=w2254:bool, element #6=w2251:bool, element #7=w2253:bool, element #8=w2250:bool)
            n1205 = Index Array(array=w2316, index #1=7 ("index"), index #2=6 ("index"), index #3=5 ("index"), index #4=4 ("index"), index #5=3 ("index"), index #6=2 ("index"), index #7=1 ("index"), index #8=0 ("index")) -> (element #1=w2265:bool, element #2=w2261:bool, element #3=w2264:bool, element #4=w2260:bool, element #5=w2263:bool, element #6=w2259:bool, element #7=w2262:bool, element #8=w2258:bool)
            n1206 = Index Array(array=w2246, index #1=7 ("index"), index #2=6 ("index"), index #3=5 ("index"), index #4=4 ("index"), index #5=3 ("index"), index #6=2 ("index"), index #7=1 ("index"), index #8=0 ("index")) -> (element #1=w2237:bool, element #2=w2236:bool, element #3=→"BMS IC Wake" →"BMS IC Awake":bool, element #4=→"BMS IC Fault" →"BMS IC Error":bool, element #5=→"Radio CS" →"Radio CS":bool, element #6=→"Logging Status" →"Logging Status" →"Logging":bool, element #7=→"Overvoltage":bool)  [unwired: 1 out]
            n1207 = And(x=w2306, y=u8 15) -> (x .and. y?=→"Undervoltage Errrors":u8)
            n1208 = Index Array(array=w2333, index #1=7 ("index"), index #2=6 ("index"), index #3=5 ("index"), index #4=4 ("index"), index #5=3 ("index"), index #6=2 ("index"), index #7=1 ("index"), index #8=0 ("index")) -> (element #1=→"Main Switch" →"Main Switch 2":bool, element #2=→"MP Switch" →"MP Switch 2":bool, element #3=→"SC BOTS &\nINS & CKS" →"SC State" →"SC State 2":bool, element #4=→"12V Out 1" →"12V Out 1 2":bool, element #5=→"12V Out 2" →"12V Out 2 2" →"Radiator Cooling":bool, element #6=→"12V Out 3" →"12V Out 3 2":bool, element #7=→"12V Out 4" →"12V Out 4 2":bool, element #8=→"12V Out 5" →"12V Out 5 2":bool)
            n1209 = And(x=w2291, y=15) -> (x .and. y?=→"Overtemp Errors":i32)
            n1210 = Build Array(w2237, w2253, w2254, w2255, w2257, w2265, w2264, w2263, w2262) -> (→"Status LEDs Green":bool[])
            n1211 = Build Array(w2236, w2250, w2251, w2252, w2256, w2261, w2260, w2259, w2258) -> (→"Status LEDs Red":bool[])
          }
          frame 817 {
            # "Offset error"
            # "PDM Status"
            n1212 = Index Array(array=w2355, index=2) -> (element=w2367:u8)
            n1213 = Index Array(array=w2355, index=3) -> (element=w2368:u8)
            n1214 = Index Array(array=w2355, index=4) -> (element=w2375:u8)
            n1215 = Index Array(array=w2355, index=5) -> (element=w2376:u8)
            n1216 = Index Array(array=w2355, index=6) -> (element=w2371:u8)
            n1217 = Index Array(array=w2355, index=7) -> (element=w2372:u8)
            n1218 = Join Numbers(hi=w2367, lo=w2368) -> ((hi.lo)=w2345:u16)
            n1219 = Join Numbers(hi=w2375, lo=w2376) -> ((hi.lo)=w2352:u16)
            n1220 = Join Numbers(hi=w2371, lo=w2372) -> ((hi.lo)=w2344:u16)
            n1221 = To Unsigned Word Integer(number=w2345) -> (unsigned 16bit integer=w2346:u16)
            n1222 = To Word Integer(number=w2352) -> (16bit integer=w2351:i16)
            n1223 = To Unsigned Word Integer(number=w2344) -> (unsigned 16bit integer=w2343:u16)
            n1224 = feedback #33() -> (w2354:dbl)  [unwired: 1 in]
            n1225 = feedback #34() -> (w2364:dbl)  [unwired: 1 in]
            n1226 = To Double Precision Float(number=w2346) -> (double precision float=w2353:dbl)
            n1227 = feedback #35() -> (w2366:dbl)  [unwired: 1 in]
            n1228 = To Double Precision Float(number=w2351) -> (double precision float=w2350:dbl)
            n1229 = To Double Precision Float(number=w2343) -> (double precision float=w2362:dbl)
            n1230 = formula code="y_=a*x+(1-a)*y;"("x"=w2353, "y"=w2354, "a"=0.1 ("input variable")) -> ("y_"=w2347:dbl)
            n1231 = feedback-in #33(w2347) -> ()
            n1232 = formula code="y_=a*x+(1-a)*y;"("x"=w2350, "y"=w2366, "a"=0.1 ("input variable")) -> ("y_"=w2342:dbl)
            "48V Current [mA]" <- w2342
            n1233 = feedback-in #35(w2342) -> ()
            n1234 = formula code="y_=a*x+(1-a)*y;"("x"=w2362, "y"=w2364, "a"=0.1 ("input variable")) -> ("y_"=w2341:dbl)
            "12V Current [mA]" <- w2341
            n1235 = feedback-in #34(w2341) -> ()
            n1236 = Divide(x=w2347, y=1000.0) -> (x/y=→"LV Voltage [V]":dbl)
            n1237 = Divide(x=w2342, y=1000.0) -> (x/y=→"48V Current [A]":dbl)
            n1238 = Bundle("y_"=w2342, "y_"=w2341) -> (→"LV Current":cluster{"y_":dbl, "y_":dbl})  [unwired: 1 in]
            n1239 = Divide(x=w2341, y=1000.0) -> (x/y=→"12V Current [A]":dbl)
          }
          frame 819 {
            n1240 = Index Array(array=w2389, index=2) -> (element=w2391:u8)
            n1241 = Index Array(array=string[] ["nothing", "Init", "Ready", "Manual", "Autocharge", "Comm. error", "Error"], index=w2391) -> (element=→"Charger state":string)
          }
          frame 832 {
            # "MCU Power ECU Status"
            n1242 = Index Array(array=w2400, index=3) -> (element=w2452:u8)
            n1243 = Index Array(array=w2400, index=5) -> (element=w2422:u8)
            n1244 = Index Array(array=w2400, index=6) -> (element=w2399:u8)
            n1245 = Index Array(array=w2400, index=7) -> (element=w2398:u8)
            n1246 = Index Array(array=w2400, index=4) -> (element=w2441:u8)
            n1247 = Index Array(array=w2400, index=8) -> (element=w2397:u8)
            n1248 = Index Array(array=w2400, index=9) -> (element=w2396:u8)
            n1249 = Join Numbers(hi=w2399, lo=w2398) -> ((hi.lo)=→"Power A Current":u16)
            n1250 = Join Numbers(hi=w2397, lo=w2396) -> ((hi.lo)=→"Power B Current":u16)
            n1251 = Number To Boolean Array(number=w2452) -> (Boolean array=w2451:bool[])
            n1252 = Number To Boolean Array(number=w2422) -> (Boolean array=w2421:bool[])
            n1253 = Number To Boolean Array(number=w2441) -> (Boolean array=w2440:bool[])
            n1254 = Index Array(array=w2451, index #1=7 ("index"), index #2=6 ("index"), index #3=5 ("index"), index #4=4 ("index"), index #5=3 ("index"), index #6=2 ("index"), index #7=1 ("index")) -> (element #7=→"24V Power B":bool)  [unwired: 6 out]
            n1255 = Index Array(array=w2421, index #1=7 ("index"), index #2=6 ("index"), index #3=5 ("index"), index #4=4 ("index"), index #5=3 ("index"), index #6=2 ("index"), index #7=1 ("index"), index #8=0 ("index")) -> (element #2=→"MCU FL 2":bool, element #3=→"MCU FL 3":bool, element #4=→"MCU FL 4":bool, element #5=→"MCU SC Endline" →"MCU SC Endline 2":bool, element #6=→"MCU TSAL":bool, element #7=→"CAN1 Term.":bool, element #8=→"CAN2 Term.":bool)  [unwired: 1 out]
            n1256 = Index Array(array=w2440, index #1=7 ("index"), index #2=6 ("index"), index #3=5 ("index"), index #4=4 ("index"), index #5=3 ("index"), index #6=2 ("index"), index #7=1 ("index"), index #8=0 ("index")) -> (element #1=→"MCU EF A":bool, element #2=→"MCU EF B":bool, element #3=→"MCU EF2 A":bool, element #4=→"MCU EF2 B":bool, element #5=→"MCU RF 1":bool, element #6=→"MCU RF 2":bool, element #7=→"MCU RF 3":bool, element #8=→"MCU RF 4":bool)
          }
          frame 896 {
            w2485 = 4 ("index")
            w2469 = u8 128 ("y")
            # "TCU Status"
            n1257 = Index Array(array=w2488, index=2) -> (element=w2468:u8)
            n1258 = Index Array(array=w2488, index=6) -> (element=w2496:u8)
            n1259 = Index Array(array=w2488, index=9) -> (element=w2465:u8)
            n1260 = Index Array(array=w2488, index=4) -> (element=w2479:u8)
            n1261 = Index Array(array=w2488, index=5) -> (element=w2505:u8)
            n1262 = Index Array(array=w2488, index=8) -> (element=w2461:u8)
            n1263 = Index Array(array=w2488, index=3) -> (element=→"Torque %":u8)
            n1264 = Index Array(array=w2488, index=7) -> (element=w2493:u8)
            n1265 = Greater Or Equal?(x=w2461, y=u8 100) -> (x >= y?=w2460:bool)
            n1266 = case shown="False" w2460 {
              tunnel: [w2514 w2517] -> w2462
              tunnel: w2461 -> [w2510 w2517]
              tunnel: [w2512 FALSE] -> w2458
              tunnel: [FALSE TRUE] -> w2459
              frame False {
                n1267 = Greater Than 0?(x=w2510) -> (x > 0?=w2512:bool)
                n1268 = Multiply(x=w2510, y=u8 2) -> (x*y=w2514:u8)
              }
              frame True {
              }
            }
            "Regen %" <- w2462
            "Force based" <- w2458
            "Pressure based" <- w2459
            n1269 = Join Numbers(hi=w2479, lo=w2505) -> ((hi.lo)=w2476:u16)
            n1270 = And(x=w2479, y=w2469) -> (x .and. y?=w2473:u8)
            n1271 = To Unsigned Byte Integer(number=w2468) -> (unsigned 8bit integer=w2486:u8)
            n1272 = And(x=w2468, y=u8 15) -> (x .and. y?=→"Selector":u8)
            n1273 = Divide(x=w2493, y=u8 100) -> (x/y=→"LR Bias":dbl)
            n1274 = Divide(x=w2496, y=u8 2) -> (x/y=w2480:dbl)
            "Front" <- w2480
            n1275 = Divide(x=w2465, y=u8 2) -> (x/y=w2471:dbl)
            "Rear 2" <- w2471
            n1276 = formula code="if(in1==0) out1=0;\nif(in1==244) out1=5;\nif(in1==232) out1=10;\nif(in1==220) out1=15;\nif(in1==208) out1=20;\nif(in1==196) out1=25;\nif(in1==184) out1=30;\nif(in1==172) out1=35;\nif(in1==160) out1=40;\nif(in1==148) out1=45;\nif(in1==136) out1=50;\nif(in1==124) out1=55;"("in1"=w2461) -> ("out1"=→"BreakPoint":dbl)
            n1277 = And(x=w2476, y=u16 32767) -> (x .and. y?=w2475:u16)
            n1278 = Divide(x=w2473, y=w2469) -> (x/y=→"BTC":dbl)
            n1279 = Number To Boolean Array(number=w2486) -> (Boolean array=w2487:bool[])
            n1280 = Array Subset(array=w2487, index=w2485, length=w2485) -> (w2484:bool[])
            n1281 = Subtract(x=100.0, y=w2480) -> (x-y=→"Rear":dbl)
            n1282 = Subtract(x=100.0, y=w2471) -> (x-y=→"Front 2":dbl)
            n1283 = To Word Integer(number=w2475) -> (16bit integer=→"Speed RPM":i16)
            n1284 = Reverse 1D Array(array=w2484) -> (reversed array=→"Derate":bool[])
          }
          frame 897 {
            w2530 = 0.6 ("x")
            w2531 = 0.6 ("y")
            # "Acceleration X & Roll"
            n1285 = local read "Acc Z offset"() -> (w2549:dbl)
            n1286 = local read "Acc Y offset"() -> (w2518:dbl)
            n1287 = local read "AccelYRaw"() -> (w2591:dbl)
            n1288 = local read "AccelXRaw"() -> (w2595:dbl)
            n1289 = local read "AccelXRaw"() -> (w2520:dbl)
            n1290 = local read "Acc X 2"() -> (w2547:dbl)
            n1291 = local read "Acc Y 2"() -> (w2537:dbl)
            n1292 = Add(x=w2531, y=w2530) -> (x+y=w2532:dbl)
            n1293 = Index Array(array=w2576, index=5) -> (element=w2585:u8)
            n1294 = Index Array(array=w2576, index=2) -> (element=w2588:u8)
            n1295 = Index Array(array=w2576, index=3) -> (element=w2587:u8)
            n1296 = Index Array(array=w2576, index=6) -> (element=w2583:u8)
            n1297 = Index Array(array=w2576, index=7) -> (element=w2581:u8)
            n1298 = Index Array(array=w2576, index=8) -> (element=w2579:u8)
            n1299 = Index Array(array=w2576, index=9) -> (element=w2577:u8)
            n1300 = Index Array(array=w2576, index=4) -> (element=w2586:u8)
            n1301 = Subtract(x=w2537, y=w2518) -> (x-y=w2539:dbl)
            n1302 = feedback #36() -> (w2593:dbl)  [unwired: 1 in]
            n1303 = formula code="y_=a*x+(1-a)*y;"("x"=w2591, "y"=w2593, "a"=0.1 ("input variable")) -> ("y_"=w2590:dbl)
            n1304 = feedback-in #36(w2590) -> ()
            n1305 = feedback #37() -> (w2610:dbl[])  [unwired: 1 in]
            n1306 = feedback #38() -> (w2596:dbl)  [unwired: 1 in]
            n1307 = formula code="y_=a*x+(1-a)*y;"("x"=w2595, "y"=w2596, "a"=0.1 ("input variable")) -> ("y_"=w2589:dbl)
            n1308 = feedback-in #38(w2589) -> ()
            n1309 = feedback #39() -> (w2603:dbl[])  [unwired: 1 in]
            n1310 = To Byte Integer(number=w2585) -> (8bit integer=w2568:i8)
            n1311 = To Double Precision Float(number=w2588) -> (double precision float=w2615:dbl)
            n1312 = To Byte Integer(number=w2587) -> (8bit integer=w2573:i8)
            n1313 = To Byte Integer(number=w2583) -> (8bit integer=w2559:i8)
            n1314 = To Byte Integer(number=w2581) -> (8bit integer=w2558:i8)
            n1315 = To Byte Integer(number=w2579) -> (8bit integer=w2557:i8)
            n1316 = To Byte Integer(number=w2577) -> (8bit integer=w2556:i8)
            n1317 = To Byte Integer(number=w2586) -> (8bit integer=w2572:i8)
            n1318 = local read "Acc X offset 2"() -> (w2548:dbl)
            n1319 = local read "Acc Z"() -> (w2550:dbl)
            n1320 = local read "Acc Y"() -> (w2536:dbl)
            n1321 = Subtract(x=w2550, y=w2549) -> (x-y=w2546:dbl)
            n1322 = Subtract(x=w2547, y=w2548) -> (x-y=w2545:dbl)
            n1323 = Subtract(x=w2536, y=w2518) -> (x-y=w2538:dbl)
            n1324 = Multiply(x=w2530, y=w2539) -> (x*y=w2534:dbl)
            n1325 = To Double Precision Float(number=w2568) -> (double precision float=w2569:dbl)
            n1326 = To Double Precision Float(number=w2573) -> (double precision float=w2574:dbl)
            n1327 = To Double Precision Float(number=w2559) -> (double precision float=w2567:dbl)
            n1328 = To Double Precision Float(number=w2558) -> (double precision float=w2564:dbl)
            n1329 = To Double Precision Float(number=w2557) -> (double precision float=w2563:dbl)
            n1330 = To Double Precision Float(number=w2556) -> (double precision float=w2560:dbl)
            n1331 = To Double Precision Float(number=w2572) -> (double precision float=w2614:dbl)
            n1332 = Divide(x=w2615, y=2.0) -> (x/y=→"TCU_v":dbl)
            n1333 = Multiply(x=w2538, y=w2531) -> (x*y=w2535:dbl)
            n1334 = Build Array (concatenate)(w2603, w2589) -> (w2604:dbl[])
            n1335 = Negate(x=w2546) -> (-x=w2524:dbl)
            n1336 = Build Array (concatenate)(w2610, w2590) -> (w2608:dbl[])
            n1337 = Divide(x=w2569, y=20.0) -> (x/y=→"TCU_yaw":dbl)
            n1338 = Divide(x=w2614, y=50.0) -> (x/y=→"TCU_ay":dbl)
            n1339 = Build Array(w2590) -> (w2601:dbl[])
            n1340 = Build Array(w2589) -> (w2600:dbl[])
            n1341 = Divide(x=w2574, y=50.0) -> (x/y=w2521:dbl)
            "TCU_ax" <- w2521
            n1342 = Divide(x=w2567, y=127.0) -> (x/y=w2555:dbl)
            "TCU_slipFL" <- w2555
            n1343 = Divide(x=w2564, y=127.0) -> (x/y=w2554:dbl)
            "TCU_slipFR" <- w2554
            n1344 = Divide(x=w2563, y=127.0) -> (x/y=w2553:dbl)
            "TCU_slipRL" <- w2553
            n1345 = Divide(x=w2560, y=127.0) -> (x/y=w2552:dbl)
            "TCU_slipRR" <- w2552
            n1346 = Add(x=w2524, y=w2545) -> (x+y=w2544:dbl)
            n1347 = Add(x=w2535, y=w2534) -> (x+y=w2533:dbl)
            n1348 = Array Size(array=w2608) -> (size(s)=w2607:i32)
            n1349 = Bundle(w2601, w2600) -> (w2597:cluster{dbl[], dbl[]})  [unwired: 1 in]
            n1350 = Bundle(w2555, w2554, w2553, w2552) -> (→"Slip_TCU":cluster{dbl, dbl, dbl, dbl})  [unwired: 1 in]
            n1351 = Negate(x=w2544) -> (-x=w2543:dbl)
            n1352 = Negate(x=w2533) -> (-x=w2540:dbl)
            n1353 = Subtract(x=w2521, y=w2520) -> (x-y=w2519:dbl)
            "Numeric" <- w2519
            n1354 = Less?(x=w2607, y=1000) -> (x < y?=w2605:bool)
            n1355 = Divide(x=w2540, y=w2532) -> (x/y=w2529:dbl)
            n1356 = Divide(x=w2543, y=2.0) -> (x/y=w2541:dbl)
            n1357 = case shown="True" w2605 {
              tunnel: [w2625 w2634] -> w2602
              tunnel: w2604 -> [w2626 w2634]
              tunnel: [w2629 w2633] -> w2609
              tunnel: w2608 -> [w2632 w2633]
              frame False {
                n1358 = Delete From Array(array=w2632, length=1, index=0) -> (array with subset deleted=w2629:dbl[])  [unwired: 1 out]
                n1359 = Delete From Array(array=w2626, length=1, index=0) -> (array with subset deleted=w2625:dbl[])  [unwired: 1 out]
              }
              frame True {
              }
            }
            n1360 = feedback-in #37(w2609) -> ()
            n1361 = feedback-in #39(w2602) -> ()
            n1362 = Bundle(w2521, "AccelXRaw"=w2520, w2519) -> (→"TCU speed":cluster{dbl, "AccelXRaw":dbl, dbl})  [unwired: 1 in]
            n1363 = Multiply(x=9.81, y=w2541) -> (x*y=→"AccelXRaw":dbl)
            n1364 = Multiply(x=w2529, y=9.81) -> (x*y=→"AccelYRaw":dbl)
            n1365 = Bundle(w2609, w2602) -> (w2598:cluster{dbl[], dbl[]})  [unwired: 1 in]
            n1366 = Build Array(w2597, w2598) -> (→"TCU_acc":cluster{dbl[], dbl[]}[])
          }
          frame 1028 {
            # "Pedalbox Status"
            # "Pedalbox Sensor Check"
            n1367 = Index Array(array=w2642, index=3) -> (element=w2654:u8)
            n1368 = Index Array(array=w2642, index=4) -> (element=w2653:u8)
            n1369 = Index Array(array=w2642, index=4) -> (element=w2637:u8)
            n1370 = Index Array(array=w2642, index=4) -> (element=→"PD Error Info":u8)
            n1371 = Index Array(array=w2642, index=6) -> (element=w2657:u8)
            n1372 = Index Array(array=w2642, index=3) -> (element=w2646:u8)
            n1373 = Index Array(array=w2642, index=5) -> (element=w2661:u8)
            n1374 = Join Numbers(hi=w2654, lo=w2653) -> ((hi.lo)=w2652:u16)
            n1375 = Logical Shift(y=i16 -6, x=w2637) -> (x << y=w2636:u8)
            n1376 = Divide(x=w2657, y=10.0) -> (x/y=→"K_Brake":dbl)
            n1377 = Divide(x=w2661, y=10.0) -> (x/y=→"K_Throttle":dbl)
            n1378 = Number To Boolean Array(number=w2646) -> (Boolean array=w2645:bool[])
            n1379 = Index Array(array=w2645, index=7) -> (element=→"BOTS & INS & CKS":bool)
            n1380 = Logical Shift(y=i16 -7, x=w2652) -> (x << y=w2650:u16)
            n1381 = And(x=w2636, y=u8 1) -> (x .and. y?=w2635:u8)
            n1382 = Add(x=w2635, y=u16 2016) -> (x+y=→"TCU Version":u16)
            n1383 = And(x=w2650, y=u8 255) -> (x .and. y?=w2648:u16)
            n1384 = To Unsigned Byte Integer(number=w2648) -> (unsigned 8bit integer=w2647:u8)
            n1385 = Number To Boolean Array(number=w2647) -> ()  [unwired: 1 out]
          }
          frame 1029 {
            # "Throttle EEPROM"
            n1386 = Index Array(array=w2678, index=2) -> (element=w2690:u8)
            n1387 = Index Array(array=w2678, index=3) -> (element=w2689:u8)
            n1388 = Index Array(array=w2678, index=4) -> (element=w2688:u8)
            n1389 = Index Array(array=w2678, index=5) -> (element=w2687:u8)
            n1390 = Index Array(array=w2678, index=6) -> (element=w2682:u8)
            n1391 = Index Array(array=w2678, index=7) -> (element=w2681:u8)
            n1392 = Index Array(array=w2678, index=8) -> (element=w2680:u8)
            n1393 = Index Array(array=w2678, index=9) -> (element=w2679:u8)
            n1394 = Join Numbers(hi=w2690, lo=w2689) -> ((hi.lo)=→"APPS1 ADC Min":u16)
            n1395 = Join Numbers(hi=w2688, lo=w2687) -> ((hi.lo)=→"APPS1 ADC Max":u16)
            n1396 = Join Numbers(hi=w2682, lo=w2681) -> ((hi.lo)=→"APPS2 ADC Min":u16)
            n1397 = Join Numbers(hi=w2680, lo=w2679) -> ((hi.lo)=→"APPS2 ADC Max":u16)
          }
          frame 1030 {
            # "Steering EEPROM"
            n1398 = Index Array(array=w2702, index=2) -> (element=w2709:u8)
            n1399 = Index Array(array=w2702, index=3) -> (element=w2708:u8)
            n1400 = Index Array(array=w2702, index=6) -> (element=w2705:u8)
            n1401 = Index Array(array=w2702, index=7) -> (element=w2704:u8)
            n1402 = Join Numbers(hi=w2709, lo=w2708) -> ((hi.lo)=→"STA1 ADC 90":u16)
            n1403 = Join Numbers(hi=w2705, lo=w2704) -> ((hi.lo)=→"STA2 ADC 90":u16)
          }
          frame 1031 {
            # "Brake EEPROM"
            n1404 = Index Array(array=w2720, index=2) -> (element=w2737:u8)
            n1405 = Index Array(array=w2720, index=3) -> (element=w2736:u8)
            n1406 = Index Array(array=w2720, index=4) -> (element=w2735:u8)
            n1407 = Index Array(array=w2720, index=5) -> (element=w2734:u8)
            n1408 = Index Array(array=w2720, index=6) -> (element=w2729:u8)
            n1409 = Index Array(array=w2720, index=7) -> (element=w2728:u8)
            n1410 = Index Array(array=w2720, index=8) -> (element=w2727:u8)
            n1411 = Index Array(array=w2720, index=9) -> (element=w2726:u8)
            n1412 = Join Numbers(hi=w2737, lo=w2736) -> ((hi.lo)=→"BSE1 ADC Min":u16)
            n1413 = Join Numbers(hi=w2735, lo=w2734) -> ((hi.lo)=→"BSE1 ADC Max":u16)
            n1414 = Join Numbers(hi=w2729, lo=w2728) -> ((hi.lo)=→"BSE2 ADC Max":u16)
            n1415 = Join Numbers(hi=w2727, lo=w2726) -> ((hi.lo)=→"BSE2 ADC Min":u16)
          }
          frame 1032 {
            # "Steering Middle EEPROM"
            n1416 = Index Array(array=w2744, index=2) -> (element=w2753:u8)
            n1417 = Index Array(array=w2744, index=3) -> (element=w2752:u8)
            n1418 = Index Array(array=w2744, index=4) -> (element=w2751:u8)
            n1419 = Index Array(array=w2744, index=5) -> (element=w2750:u8)
            n1420 = Join Numbers(hi=w2753, lo=w2752) -> ((hi.lo)=→"STA1 ADC Null":u16)
            n1421 = Join Numbers(hi=w2751, lo=w2750) -> ((hi.lo)=→"STA2 ADC Null":u16)
          }
          frame 1057 {
            w2781 = 0.1 ("input variable")
            # "Right in and out are permuted"
            # "Left in and out are permuted"
            # "Left in and out are permuted"
            # "Right in and out are permuted"
            n1422 = Index Array(array=w2799, index=4) -> (element=w2806:u8)
            n1423 = Index Array(array=w2799, index=5) -> (element=w2807:u8)
            n1424 = Index Array(array=w2799, index=2) -> (element=w2809:u8)
            n1425 = Index Array(array=w2799, index=3) -> (element=w2808:u8)
            n1426 = Index Array(array=w2799, index=8) -> (element=w2796:u8)
            n1427 = Index Array(array=w2799, index=9) -> (element=w2795:u8)
            n1428 = Index Array(array=w2799, index=6) -> (element=w2801:u8)
            n1429 = Index Array(array=w2799, index=7) -> (element=w2800:u8)
            n1430 = Join Numbers(hi=w2806, lo=w2807) -> ((hi.lo)=w2791:u16)
            n1431 = Join Numbers(hi=w2809, lo=w2808) -> ((hi.lo)=w2794:u16)
            n1432 = Join Numbers(hi=w2796, lo=w2795) -> ((hi.lo)=w2788:u16)
            n1433 = Join Numbers(hi=w2801, lo=w2800) -> ((hi.lo)=w2787:u16)
            n1434 = feedback #40() -> (w2784:dbl)  [unwired: 1 in]
            n1435 = feedback #41() -> (w2785:dbl)  [unwired: 1 in]
            n1436 = feedback #42() -> (w2782:dbl)  [unwired: 1 in]
            n1437 = feedback #43() -> (w2783:dbl)  [unwired: 1 in]
            n1438 = local read "T Motor RR [°C]"() -> (w2776:dbl)
            n1439 = local read "T Motor FL [°C]"() -> (w2779:dbl)
            n1440 = local read "T Motor FR [°C]"() -> (w2778:dbl)
            n1441 = local read "T Motor RL [°C]"() -> (w2777:dbl)
            n1442 = local read "IGBT RR TEMP"() -> (w2759:dbl)
            n1443 = local read "IGBT FL TEMP"() -> (w2762:i16)
            n1444 = local read "IGBT FR TEMP"() -> (w2761:dbl)
            n1445 = local read "IGBT RL TEMP"() -> (w2760:dbl)
            n1446 = local read "T Inv. RR [°C]"() -> (w2775:dbl)
            n1447 = local read "T Inv. FL [°C]"() -> (w2772:dbl)
            n1448 = local read "T Inv. FR [°C]"() -> (w2773:dbl)
            n1449 = local read "T Inv. RL [°C]"() -> (w2774:dbl)
            n1450 = Bundle("IGBT FL TEMP"=w2762, "IGBT FR TEMP"=w2761, "IGBT RL TEMP"=w2760, "IGBT RR TEMP"=w2759) -> (→"IGBT Temperature":T2)  [unwired: 1 in]
            n1451 = Bundle("T Motor FL [°C]"=w2779, "T Motor FR [°C]"=w2778, "T Motor RL [°C]"=w2777, "T Motor RR [°C]"=w2776) -> (→"Motor Temperature":T19)  [unwired: 1 in]
            n1452 = Bundle("T Inv. FL [°C]"=w2772, "T Inv. FR [°C]"=w2773, "T Inv. RL [°C]"=w2774, "T Inv. RR [°C]"=w2775) -> (→"Inverter Temperature":T20)  [unwired: 1 in]
            n1453 = Divide(x=w2791, y=10.0) -> (x/y=w2765:dbl)
            "Radiator Left IN" <- w2765
            n1454 = Divide(x=w2794, y=10.0) -> (x/y=w2766:dbl)
            "Radiator Left OUT" <- w2766
            n1455 = Divide(x=w2788, y=10.0) -> (x/y=w2763:dbl)
            "Radiator Right IN" <- w2763
            n1456 = Divide(x=w2787, y=10.0) -> (x/y=w2764:dbl)
            "Radiator Right OUT" <- w2764
            n1457 = formula code="y_=a*x+(1-a)*y;"("x"=w2766, "y"=w2785, "a"=w2781) -> ("y_"=w2770:dbl)
            n1458 = feedback-in #41(w2770) -> ()
            n1459 = formula code="y_=a*x+(1-a)*y;"("x"=w2765, "y"=w2784, "a"=w2781) -> ("y_"=w2769:dbl)
            n1460 = feedback-in #40(w2769) -> ()
            n1461 = formula code="y_=a*x+(1-a)*y;"("x"=w2763, "y"=w2782, "a"=w2781) -> ("y_"=w2767:dbl)
            n1462 = feedback-in #42(w2767) -> ()
            n1463 = formula code="y_=a*x+(1-a)*y;"("x"=w2764, "y"=w2783, "a"=w2781) -> ("y_"=w2768:dbl)
            n1464 = feedback-in #43(w2768) -> ()
            n1465 = Bundle("y_"=w2769, "y_"=w2770, "y_"=w2767, "y_"=w2768) -> (→"Radiator Temperature":cluster{"y_":dbl, "y_":dbl, "y_":dbl, "y_":dbl})  [unwired: 1 in]
          }
          frame 1058 {
            w2850 = 0.1 ("input variable")
            n1466 = Index Array(array=w2855, index=2) -> (element=w2861:u8)
            n1467 = Index Array(array=w2855, index=3) -> (element=w2860:u8)
            n1468 = Index Array(array=w2855, index=4) -> (element=w2858:u8)
            n1469 = Index Array(array=w2855, index=5) -> (element=w2859:u8)
            n1470 = feedback #44() -> (w2851:dbl)  [unwired: 1 in]
            n1471 = feedback #45() -> (w2853:dbl)  [unwired: 1 in]
            n1472 = feedback #46() -> (w2854:dbl)  [unwired: 1 in]
            n1473 = feedback #47() -> (w2852:dbl)  [unwired: 1 in]
            n1474 = local read "Wheel Travel FR"() -> (w2822:u16)
            n1475 = local read "Wheel Travel FL"() -> (w2818:u16)
            n1476 = Join Numbers(hi=w2861, lo=w2860) -> ((hi.lo)=w2844:u16)
            "Wheel Travel RL" <- w2844
            n1477 = Join Numbers(hi=w2858, lo=w2859) -> ((hi.lo)=w2817:u16)
            "Wheel Travel RR" <- w2817
            n1478 = Subtract(x=w2818, y="Wheel Travel FL Offset") -> (x-y=w2831:dbl)
            n1479 = Subtract(x=w2844, y="Wheel Travel RL Offset") -> (x-y=w2842:dbl)
            n1480 = Subtract(x=w2817, y="Wheel Travel RR Offset") -> (x-y=w2836:dbl)
            n1481 = Subtract(x=w2822, y="Wheel Travel FR") -> (x-y=w2826:dbl)
            n1482 = formula code="y_=a*x+(1-a)*y;"("x"=w2822, "y"=w2851, "a"=w2850) -> ("y_"=w2848:dbl)
            n1483 = feedback-in #44(w2848) -> ()
            n1484 = formula code="y_=a*x+(1-a)*y;"("x"=w2844, "y"=w2854, "a"=w2850) -> ("y_"=w2847:dbl)
            n1485 = feedback-in #46(w2847) -> ()
            n1486 = formula code="y_=a*x+(1-a)*y;"("x"=w2818, "y"=w2852, "a"=w2850) -> ("y_"=w2849:dbl)
            n1487 = feedback-in #47(w2849) -> ()
            n1488 = formula code="y_=a*x+(1-a)*y;"("x"=w2817, "y"=w2853, "a"=w2850) -> ("y_"=w2846:dbl)
            n1489 = feedback-in #45(w2846) -> ()
            n1490 = Bundle("y_"=w2849, "y_"=w2848, "y_"=w2847, "y_"=w2846) -> (→"Wheel Travel":cluster{"y_":dbl, "y_":dbl, "y_":dbl, "y_":dbl})  [unwired: 1 in]
            n1491 = Multiply(x=w2831, y=75.0) -> (x*y=w2829:dbl)
            n1492 = Multiply(x=w2842, y=75.0) -> (x*y=w2840:dbl)
            n1493 = Multiply(x=w2836, y=75.0) -> (x*y=w2834:dbl)
            n1494 = Multiply(x=w2826, y=75.0) -> (x*y=w2824:dbl)
            n1495 = Divide(x=w2829, y=4095.0) -> (x/y=→"Damper Travel FL [mm]":dbl)
            n1496 = Divide(x=w2840, y=4095.0) -> (x/y=→"Damper Travel RL [mm]":dbl)
            n1497 = Divide(x=w2834, y=4095.0) -> (x/y=→"Damper Travel RR [mm]":dbl)
            n1498 = Divide(x=w2824, y=4095.0) -> (x/y=→"Damper Travel FR [mm]":dbl)
          }
          frame 1074 {
            w2897 = u8 127 ("y")
            # "PDM LV Cell Values"
            n1499 = Index Array(array=w2878, index=5) -> (element=w2902:u8)
            n1500 = Index Array(array=w2878, index=6) -> (element=w2901:u8)
            n1501 = Index Array(array=w2878, index=2) -> (element=w2906:u8)
            n1502 = Index Array(array=w2878, index=3) -> (element=w2898:u8)
            n1503 = Index Array(array=w2878, index=4) -> (element=w2907:u8)
            n1504 = Join Numbers(hi=w2902, lo=w2901) -> ((hi.lo)=w2900:u16)
            n1505 = Greater?(x=w2898, y=w2897) -> (0:w2894:bool)
            n1506 = And(x=w2898, y=w2897) -> (x .and. y?=w2899:u8)
            n1507 = Decrement(x=w2906) -> (x-1=w2893:u8)
            n1508 = Join Numbers(hi=w2899, lo=w2907) -> ((hi.lo)=w2905:u16)
            n1509 = Replace Array Subset(array=w2889, new element=w2900, index=w2893) -> (w2886:dbl[])
            n1510 = Replace Array Subset(array=w2892, new element=w2894, index=w2893) -> (w2890:bool[])
            "Discharge" <- w2890
            n1511 = Replace Array Subset(array=w2896, new element=w2905, index=w2893) -> (w2880:u16[])
            n1512 = Divide(x=w2886, y=10.0) -> (x/y=w2884:dbl[])
            "LV Temp" <- w2884
            n1513 = for {
              tunnel: [w2912] -> w2891 mode=indexing
              tunnel: w2880 -> [w2911] mode=indexing
              n1514 = Bundle(w2911, w2911) -> (w2912:cluster{u16, u16})  [unwired: 1 in]
            }
            "LV Battery" <- w2891
            n1515 = Array Subset(array=w2880, index=0, length=12) -> (w2883:u16[])
            n1516 = Array To Cluster(array=w2880) -> (cluster=→"LV Cell Voltages":T4)
            n1517 = Array Max & Min(array=w2884) -> (max value=→"LV Temp":dbl)  [unwired: 3 out]
            n1518 = Array Max & Min(array=w2883) -> (max value=w2871:u16, min value=w2870:u16)  [unwired: 2 out]
            "LV Min" <- w2870
            "LV Max" <- w2871
            n1519 = Greater?(x=w2871, y="LV Max Limit") -> (0:w2876:bool)
            n1520 = Greater?(x="LV Min Limit", y=w2870) -> (0:w2874:bool)
            n1521 = Or(x=w2876, y=w2874) -> (x .or. y?=w2873:bool)
            n1522 = And(x=w2873, y="Enable LV alert") -> (x .and. y?=w2869:bool)
            n1523 = call "alert.vi"("Turn on"=w2869) -> ()  [unwired: 3 in, 1 out]
          }
          frame 1075 {
            n1524 = Index Array(array=w2919, index=2) -> (element=→"ASMS":u8)
          }
          frame 1377 {
            n1525 = Index Array(array=w2926, index=2) -> (element=→"Pedal Heartbeat":u8)
          }
          frame 1378 {
            # "Dashboard GPIO States"
            n1526 = Index Array(array=w2930, index=2) -> (element=→"Dash Heartbeat":u8)
            n1527 = Index Array(array=w2930, index=4) -> (element=w2947:u8)
            n1528 = Number To Boolean Array(number=w2947) -> (Boolean array=w2946:bool[])
            n1529 = Index Array(array=w2946, index #1=7 ("index"), index #2=6 ("index"), index #3=5 ("index"), index #4=4 ("index"), index #5=3 ("index"), index #6=2 ("index"), index #7=1 ("index"), index #8=0 ("index")) -> (element #3=→"OFF Button":bool, element #4=→"START Button":bool, element #5=→"ON Button":bool, element #6=→"BLANK":bool, element #7=→"XLAT":bool, element #8=→"MODE":bool)  [unwired: 2 out]
          }
          frame 1105 {
            n1530 = Index Array(array=w2956, index=2) -> (element=w2962:u8)
            n1531 = Index Array(array=w2956, index=3) -> (element=w2961:u8)
            n1532 = Index Array(array=w2956, index=4) -> (element=w2959:u8)
            n1533 = Index Array(array=w2956, index=5) -> (element=w2960:u8)
            n1534 = Join Numbers(hi=w2962, lo=w2961) -> ((hi.lo)=→"Wheel Travel FL":u16)
            n1535 = Join Numbers(hi=w2959, lo=w2960) -> ((hi.lo)=→"Wheel Travel FR":u16)
          }
          frame 1152 {
            n1536 = Array Subset(array=w2973, index=2, length=8) -> (→"CAN Missing Message":u8[])
          }
          frame 1153 {
            # "TCU Status 2"
            n1537 = Index Array(array=w3007, index=8) -> (element=w3004:u8)
            n1538 = Index Array(array=w3007, index=9) -> (element=w2982:u8)
            n1539 = Index Array(array=w3007, index=6) -> (element=w2992:u8)
            n1540 = Index Array(array=w3007, index=7) -> (element=w2988:u8)
            n1541 = Index Array(array=w3007, index=5) -> (element=w3015:u8)
            n1542 = Index Array(array=w3007, index=4) -> (element=→"Drop":u8)
            n1543 = Index Array(array=w3007, index=2) -> (element=→"Max Power":u8)
            n1544 = Index Array(array=w3007, index=3) -> (element=w3025:u8)
            n1545 = To Double Precision Float(number=100 ("index")) -> (double precision float=w2995:dbl)
            n1546 = And(x=u8 127 ("y"), y=w2982) -> (x .and. y?=w2986:u8)
            n1547 = Greater?(x=w2982, y=u8 127) -> (0:→"LaunchControl_Active":bool)
            n1548 = To Double Precision Float(number=w2986) -> (double precision float=w2984:dbl)
            n1549 = Divide(x=w2984, y=10.0) -> (x/y=→"LaunchControl_Mu":dbl)
            n1550 = To Double Precision Float(number=w2992) -> (double precision float=w2993:dbl)
            n1551 = To Long Integer(number=w2988) -> (32bit integer=w2989:i32)
            n1552 = And(x=w3004, y=u8 248) -> (x .and. y?=w3002:u8)
            n1553 = And(x=w3015, y=u8 240) -> (x .and. y?=w3021:u8)
            n1554 = Number To Boolean Array(number=w3015) -> (Boolean array=w3014:bool[])
            n1555 = Number To Boolean Array(number=w3025) -> (Boolean array=w3042:bool[])
            n1556 = Index Array(array=w3014, index #1=3 ("index"), index #2=2 ("index"), index #3=1 ("index")) -> (element #1=→"AMK_AV":bool, element #2=→"Torque 2":bool, element #3=→"Hardcoremode ON":bool)
            n1557 = Index Array(array=w3042, index #1=7 ("index"), index #2=6 ("index"), index #3=5 ("index"), index #4=4 ("index"), index #5=3 ("index"), index #6=2 ("index"), index #7=1 ("index"), index #8=0 ("index")) -> (element #1=→"Safety Mode Enabled":bool, element #2=→"Power Limiter Enabled":bool, element #3=→"Keylock Enable":bool, element #4=→"Throttle_Constant":bool, element #5=→"SlipControl_Enabled":bool, element #6=→"Torque_Coeff":bool, element #7=→"Torque_Derate":bool, element #8=→"Smooth_Transition_Enabled":bool)
            n1558 = Divide(x=w2993, y=w2995) -> (x/y=→"GasPedal Heartbeat":dbl)
            n1559 = To Double Precision Float(number=w3002) -> (double precision float=w3001:dbl)
            n1560 = To Double Precision Float(number=w3021) -> (double precision float=w3020:dbl)
            n1561 = Multiply(x=w2989, y=10 ("index")) -> (x*y=→"M_COG":i32)
            n1562 = Divide(x=w3001, y=8.0) -> (x/y=w2999:dbl)
            n1563 = Divide(x=w3020, y=16.0) -> (x/y=→"Characteristics Approx":dbl)
            n1564 = Multiply(x=w2999, y=1000.0) -> (x*y=→"PowerLimiter Approx":dbl)
          }
          frame 1154 {
            n1565 = Index Array(array=w3155, index=2) -> (element=w3152:u8)
            n1566 = Index Array(array=w3155, index=6) -> (element=w3052:u8)
            n1567 = Index Array(array=w3155, index=9) -> (element=w3081:u8)
            n1568 = Index Array(array=w3155, index=4) -> (element=w3148:u8)
            n1569 = Index Array(array=w3155, index=8) -> (element=w3069:u8)
            n1570 = Index Array(array=w3155, index=3) -> (element=w3130:u8)
            n1571 = Index Array(array=w3155, index=5) -> (element=w3113:u8)
            n1572 = Index Array(array=w3155, index=7) -> (element=w3096:u8)
            n1573 = To Unsigned Byte Integer(number=w3152) -> (unsigned 8bit integer=w3154:u8)
            n1574 = To Unsigned Byte Integer(number=w3148) -> (unsigned 8bit integer=w3150:u8)
            n1575 = Number To Boolean Array(number=w3052) -> (Boolean array=w3054:bool[])
            n1576 = Number To Boolean Array(number=w3081) -> (Boolean array=w3095:bool[])
            n1577 = Number To Boolean Array(number=w3069) -> (Boolean array=w3072:bool[])
            n1578 = Number To Boolean Array(number=w3130) -> (Boolean array=w3146:bool[])
            n1579 = Number To Boolean Array(number=w3113) -> (Boolean array=w3129:bool[])
            n1580 = Number To Boolean Array(number=w3096) -> (Boolean array=w3112:bool[])
            n1581 = Index Array(array=w3054, index #1=7 ("index"), index #2=6 ("index"), index #3=5 ("index"), index #4=4 ("index"), index #5=3 ("index"), index #6=2 ("index"), index #7=1 ("index"), index #8=0 ("index")) -> (element #1=→"Error_BrakeValidity_1_raw":bool, element #2=→"Error_BrakeValidity_2_raw":bool, element #3=→"Error_ThrottleValidity_1_raw":bool, element #4=→"Error_ThrottleValidity_2_raw":bool, element #5=→"Error_SteeringAngleValidity_1_raw":bool, element #6=→"Error_SteeringAngleValidity_2_raw":bool, element #7=→"Error_Pedalbox_Heartbeat_raw":bool, element #8=→"Error_SteeringControl_Heartbeat_raw":bool)
            n1582 = Index Array(array=w3095, index #1=7 ("index"), index #2=6 ("index"), index #3=5 ("index"), index #4=4 ("index"), index #5=3 ("index"), index #6=2 ("index"), index #7=1 ("index"), index #8=0 ("index")) -> (element #4=→"Error HV Accu. Voltage":bool, element #5=→"Error HV Accu. Current":bool, element #6=→"Error Cell Voltage":bool, element #7=→"Error Cell Voltage Sensor":bool, element #8=→"Error Cell Temperature":bool)  [unwired: 3 out]
            n1583 = Index Array(array=w3072, index #1=7 ("index"), index #2=6 ("index"), index #3=5 ("index"), index #4=4 ("index"), index #5=3 ("index"), index #6=2 ("index"), index #7=1 ("index"), index #8=0 ("index")) -> (element #7=→"Error_LVCellVoltage":bool, element #8=→"Error_LVCellTemperature":bool)  [unwired: 6 out]
            n1584 = Index Array(array=w3146, index #1=7 ("index"), index #2=6 ("index"), index #3=5 ("index"), index #4=4 ("index"), index #5=3 ("index"), index #6=2 ("index"), index #7=1 ("index"), index #8=0 ("index")) -> (element #2=→"Error_ThrottleValidity_1_raw 2":bool, element #3=→"Error_ThrottleValidity_2_raw 2":bool, element #4=→"Error Throttle Position 1":bool, element #5=→"Error Throttle Position 2":bool, element #6=→"Error Throttle Validity 1":bool, element #7=→"Error Throttle Validity 2":bool, element #8=→"Error Throttle Plausability":bool)  [unwired: 1 out]
            n1585 = Index Array(array=w3129, index #1=7 ("index"), index #2=6 ("index"), index #3=5 ("index"), index #4=4 ("index"), index #5=3 ("index"), index #6=2 ("index"), index #7=1 ("index"), index #8=0 ("index")) -> (element #2=→"Error_BrakeValidity_1_raw  2":bool, element #3=→"Error_BrakeValidity_2_raw 2":bool, element #4=→"Error Brake Position 1":bool, element #5=→"Error Brake Position 2":bool, element #6=→"Error Brake Validity  1":bool, element #7=→"Error Brake Validity 2":bool, element #8=→"Error Brake Plausability":bool)  [unwired: 1 out]
            n1586 = Index Array(array=w3112, index #1=7 ("index"), index #2=6 ("index"), index #3=5 ("index"), index #4=4 ("index"), index #5=3 ("index"), index #6=2 ("index"), index #7=1 ("index"), index #8=0 ("index")) -> (element #2=→"Error_SteeringAngleValidity_1_raw 2":bool, element #3=→"Error_SteeringAngleValidity_2_raw 2":bool, element #4=→"Error Steering Angle 1":bool, element #5=→"Error Steering Angle 2":bool, element #6=→"Error Steering Validity 1":bool, element #7=→"Error Steering Validity 2":bool, element #8=→"Error Steering Plausability":bool)  [unwired: 1 out]
            n1587 = Equal?(x=u8 1, y=w3154) -> (x = y?=→"Message Arrived":bool)
            n1588 = Equal?(x=u8 2, y=w3150) -> (x = y?=→"Message Arrived 2":bool)
          }
          frame 1155 {
            n1589 = Index Array(array=w3173, index=2) -> (element=w3186:u8)
            n1590 = Index Array(array=w3173, index=3) -> (element=w3247:u8)
            n1591 = Index Array(array=w3173, index=4) -> (element=w3182:u8)
            n1592 = Index Array(array=w3173, index=5) -> (element=w3236:u8)
            n1593 = Index Array(array=w3173, index=8) -> (element=w3174:u8)
            n1594 = Index Array(array=w3173, index=6) -> (element=w3178:u8)
            n1595 = Index Array(array=w3173, index=9) -> (element=w3190:u8)
            n1596 = Index Array(array=w3173, index=7) -> (element=w3225:u8)
            n1597 = To Unsigned Byte Integer(number=w3186) -> (unsigned 8bit integer=w3189:u8)
            n1598 = To Unsigned Byte Integer(number=w3182) -> (unsigned 8bit integer=w3185:u8)
            n1599 = To Unsigned Byte Integer(number=w3174) -> (unsigned 8bit integer=w3177:u8)
            n1600 = To Unsigned Byte Integer(number=w3178) -> (unsigned 8bit integer=w3181:u8)
            n1601 = Number To Boolean Array(number=w3247) -> (Boolean array=w3256:bool[])
            n1602 = Number To Boolean Array(number=w3236) -> (Boolean array=w3245:bool[])
            n1603 = Number To Boolean Array(number=w3190) -> (Boolean array=w3223:bool[])
            n1604 = Number To Boolean Array(number=w3225) -> (Boolean array=w3234:bool[])
            n1605 = Index Array(array=w3256, index #1=7 ("index"), index #2=6 ("index"), index #3=5 ("index"), index #4=4 ("index"), index #5=3 ("index"), index #6=2 ("index"), index #7=1 ("index"), index #8=0 ("index")) -> (element #3=→"FL TargetVelo OverTresh":bool, element #4=→"FL TargetVelo UnderTresh":bool, element #5=→"FL TorqueLimPos OverTresh":bool, element #6=→"FL TorqueLimPos UnderTresh":bool, element #7=→"FL TorqueLimNeg OverTresh":bool, element #8=→"FL TorqueLimNeg UnderTresh":bool)  [unwired: 2 out]
            n1606 = Index Array(array=w3245, index #1=7 ("index"), index #2=6 ("index"), index #3=5 ("index"), index #4=4 ("index"), index #5=3 ("index"), index #6=2 ("index"), index #7=1 ("index"), index #8=0 ("index")) -> (element #3=→"FR TargetVelo OverTresh":bool, element #4=→"FR TargetVelo UnderTresh":bool, element #5=→"FR TorqueLimPos OverTresh":bool, element #6=→"FR TorqueLimPos UnderTresh":bool, element #7=→"FR TorqueLimNeg OverTresh":bool, element #8=→"FR TorqueLimNeg UnderTresh":bool)  [unwired: 2 out]
            n1607 = Index Array(array=w3223, index #1=7 ("index"), index #2=6 ("index"), index #3=5 ("index"), index #4=4 ("index"), index #5=3 ("index"), index #6=2 ("index"), index #7=1 ("index"), index #8=0 ("index")) -> (element #3=→"RR TargetVelo OverTresh":bool, element #4=→"RR TargetVelo UnderTresh":bool, element #5=→"RR TorqueLimPos OverTresh":bool, element #6=→"RR TorqueLimPos UnderTresh":bool, element #7=→"RR TorqueLimNeg OverTresh":bool, element #8=→"RR TorqueLimNeg UnderTresh":bool)  [unwired: 2 out]
            n1608 = Index Array(array=w3234, index #1=7 ("index"), index #2=6 ("index"), index #3=5 ("index"), index #4=4 ("index"), index #5=3 ("index"), index #6=2 ("index"), index #7=1 ("index"), index #8=0 ("index")) -> (element #3=→"RL TargetVelo OverTresh":bool, element #4=→"RL TargetVelo UnderTresh":bool, element #5=→"RL TorqueLimPos OverTresh":bool, element #6=→"RL TorqueLimPos UnderTresh":bool, element #7=→"RL TorqueLimNeg OverTresh":bool, element #8=→"RL TorqueLimNeg UnderTresh":bool)  [unwired: 2 out]
            n1609 = Equal?(x=u8 13, y=w3189) -> (x = y?=→"Message Arrived 11":bool)
            n1610 = Equal?(x=u8 14, y=w3185) -> (x = y?=→"Message Arrived 12":bool)
            n1611 = Equal?(x=u8 16, y=w3177) -> (x = y?=→"Message Arrived 14":bool)
            n1612 = Equal?(x=u8 15, y=w3181) -> (x = y?=→"Message Arrived 13":bool)
          }
          frame 1156 {
            n1613 = Index Array(array=w3278, index=3) -> (element=w3281:u8)
            n1614 = Index Array(array=w3278, index=7) -> (element=w3328:u8)
            n1615 = Index Array(array=w3278, index=5) -> (element=w3283:u8)
            n1616 = Index Array(array=w3278, index=8) -> (element=w3329:u8)
            n1617 = Index Array(array=w3278, index=2) -> (element=w3280:u8)
            n1618 = Index Array(array=w3278, index=9) -> (element=w3277:u8)
            n1619 = Index Array(array=w3278, index=6) -> (element=w3332:u8)
            n1620 = Index Array(array=w3278, index=4) -> (element=w3282:u8)
            n1621 = To Unsigned Byte Integer(number=w3277) -> (unsigned 8bit integer=w3274:u8)
            n1622 = Number To Boolean Array(number=w3281) -> (Boolean array=w3317:bool[])
            n1623 = Number To Boolean Array(number=w3328) -> (Boolean array=w3359:bool[])
            n1624 = Number To Boolean Array(number=w3283) -> (Boolean array=w3297:bool[])
            n1625 = Number To Boolean Array(number=w3329) -> (Boolean array=w3350:bool[])
            n1626 = Number To Boolean Array(number=w3280) -> (Boolean array=w3327:bool[])
            n1627 = Number To Boolean Array(number=w3332) -> (Boolean array=w3373:bool[])
            n1628 = Number To Boolean Array(number=w3282) -> (Boolean array=w3307:bool[])
            n1629 = Index Array(array=w3317, index #1=7 ("index"), index #2=6 ("index"), index #3=5 ("index"), index #4=4 ("index"), index #5=3 ("index"), index #6=2 ("index"), index #7=1 ("index"), index #8=0 ("index")) -> (element #8=→"Error Actual Velocity FR":bool)  [unwired: 7 out]
            n1630 = Index Array(array=w3359, index #1=7 ("index"), index #2=6 ("index"), index #3=5 ("index"), index #4=4 ("index"), index #5=3 ("index"), index #6=2 ("index"), index #7=1 ("index"), index #8=0 ("index")) -> (element #1=→"Error BrPressure Front Validity":bool, element #2=→"Error BrPressure Rear Validity":bool, element #3=→"Error BrPressure Front":bool, element #4=→"Error BrPressure Rear 2":bool, element #5=→"Error BrPressure Front Validity_raw":bool, element #6=→"Error BrPressure Rear Validity_raw":bool, element #7=→"Error Steering Heartbeat":bool, element #8=→"Error Pedalbox Heartbeat":bool)
            n1631 = Index Array(array=w3297, index #1=7 ("index"), index #2=6 ("index"), index #3=5 ("index"), index #4=4 ("index"), index #5=3 ("index"), index #6=2 ("index"), index #7=1 ("index"), index #8=0 ("index")) -> (element #8=→"Error Actual Velocity RR":bool)  [unwired: 7 out]
            n1632 = Index Array(array=w3350, index #1=7 ("index"), index #2=6 ("index"), index #3=5 ("index"), index #4=4 ("index"), index #5=3 ("index"), index #6=2 ("index"), index #7=1 ("index"), index #8=0 ("index")) -> (element #3=→"CriticalHVCell Heartbeat raw":bool, element #4=→"CriticalHVCell Heartbeat":bool, element #5=→"Error_Button_4":bool, element #6=→"Error_Button_3":bool, element #7=→"Error_Button_2":bool, element #8=→"Error_Button_1":bool)  [unwired: 2 out]
            n1633 = Index Array(array=w3327, index #1=7 ("index"), index #2=6 ("index"), index #3=5 ("index"), index #4=4 ("index"), index #5=3 ("index"), index #6=2 ("index"), index #7=1 ("index"), index #8=0 ("index")) -> (element #8=→"Error Actual Velocity FL":bool)  [unwired: 7 out]
            n1634 = Index Array(array=w3373, index #1=7 ("index"), index #2=6 ("index"), index #3=5 ("index"), index #4=4 ("index"), index #5=3 ("index"), index #6=2 ("index"), index #7=1 ("index"), index #8=0 ("index")) -> (element #4=→"Error Rot Switch 1":bool, element #5=→"Error Rot Switch 2":bool, element #6=→"Error Rot Switch 3":bool, element #7=→"Error Rot Switch 4":bool, element #8=→"Error Rot Switch 5":bool)  [unwired: 3 out]
            n1635 = Index Array(array=w3307, index #1=7 ("index"), index #2=6 ("index"), index #3=5 ("index"), index #4=4 ("index"), index #5=3 ("index"), index #6=2 ("index"), index #7=1 ("index"), index #8=0 ("index")) -> (element #8=→"Error Actual Velocity RL":bool)  [unwired: 7 out]
            n1636 = Equal?(x=17 ("index"), y=w3274) -> (x = y?=→"Other messages arrived":bool)
          }
          frame 1157 {
            n1637 = Index Array(array=w3393, index=2) -> (element=w3389:u8)
            n1638 = Index Array(array=w3393, index=3) -> (element=w3418:u8)
            n1639 = Index Array(array=w3393, index=4) -> (element=w3417:u8)
            n1640 = Index Array(array=w3393, index=5) -> (element=w3414:u8)
            n1641 = Index Array(array=w3393, index=6) -> (element=w3409:u8)
            n1642 = Index Array(array=w3393, index=7) -> (element=w3404:u8)
            n1643 = Index Array(array=w3393, index=8) -> (element=w3399:u8)
            n1644 = Index Array(array=w3393, index=9) -> (element=w3394:u8)
            n1645 = To Double Precision Float(number=128 ("index")) -> (double precision float=w3425:dbl)
            n1646 = To Long Integer(number=w3418) -> (32bit integer=w3472:i32)
            n1647 = To Double Precision Float(number=w3418) -> (double precision float=w3471:dbl)
            n1648 = To Double Precision Float(number=w3418) -> (double precision float=w3461:dbl)
            n1649 = To Double Precision Float(number=w3418) -> (double precision float=w3453:dbl)
            n1650 = To Double Precision Float(number=w3418) -> (double precision float=w3444:dbl)
            n1651 = To Double Precision Float(number=w3418) -> (double precision float=w3435:dbl)
            n1652 = To Double Precision Float(number=w3418) -> (double precision float=w3426:dbl)
            n1653 = To Double Precision Float(number=w3417) -> (double precision float=w3416:dbl)
            n1654 = To Double Precision Float(number=w3414) -> (double precision float=w3415:dbl)
            n1655 = To Long Integer(number=w3409) -> (32bit integer=w3410:i32)
            n1656 = To Long Integer(number=w3404) -> (32bit integer=w3405:i32)
            n1657 = To Long Integer(number=w3399) -> (32bit integer=w3400:i32)
            n1658 = To Long Integer(number=w3394) -> (32bit integer=w3395:i32)
            n1659 = To Long Integer(number=w3389) -> (32bit integer=w3380:i32)
            n1660 = Divide(x=w3426, y=w3425) -> (x/y=w3422:dbl)
            n1661 = And(x=w3380, y=7 ("index")) -> (x .and. y?=→"YawControlSelector":i32)
            n1662 = And(x=w3472, y=3 ("index")) -> (x .and. y?=→"Weight":i32)
            n1663 = Multiply(x=w3410, y=10 ("index")) -> (x*y=→"Fz_FL":i32)
            n1664 = Multiply(x=w3405, y=10 ("index")) -> (x*y=→"Fz_FR":i32)
            n1665 = Multiply(x=w3400, y=10 ("index")) -> (x*y=→"Fz_RL":i32)
            n1666 = Multiply(x=w3395, y=10 ("index")) -> (x*y=→"Fz_RR":i32)
            n1667 = And(x=w3380, y=248 ("index")) -> (x .and. y?=w3379:i32)
            n1668 = Divide(x=w3416, y=100.0 ("index")) -> (x/y=→"Tune":dbl)
            n1669 = Multiply(x=w3415, y=100.0 ("index")) -> (x*y=→"P tag":dbl)
            n1670 = To Double Precision Float(number=4 ("index")) -> (double precision float=w3470:dbl)
            n1671 = To Double Precision Float(number=8 ("index")) -> (double precision float=w3460:dbl)
            n1672 = To Double Precision Float(number=16 ("index")) -> (double precision float=w3452:dbl)
            n1673 = To Double Precision Float(number=32 ("index")) -> (double precision float=w3443:dbl)
            n1674 = To Double Precision Float(number=64 ("index")) -> (double precision float=w3434:dbl)
            n1675 = Divide(x=w3471, y=w3470) -> (x/y=w3467:dbl)
            n1676 = Divide(x=w3461, y=w3460) -> (x/y=w3388:dbl)
            n1677 = Divide(x=w3453, y=w3452) -> (x/y=w3449:dbl)
            n1678 = Divide(x=w3444, y=w3443) -> (x/y=w3440:dbl)
            n1679 = Divide(x=w3435, y=w3434) -> (x/y=w3431:dbl)
            n1680 = To Double Precision Float(number=w3379) -> (double precision float=w3378:dbl)
            n1681 = Round Toward -Infinity(1:w3422) -> (0:w3383:dbl)
            n1682 = Round Toward -Infinity(1:w3467) -> (0:w3382:dbl)
            n1683 = Round Toward -Infinity(1:w3388) -> (0:w3387:dbl)
            n1684 = Round Toward -Infinity(1:w3449) -> (0:w3386:dbl)
            n1685 = Round Toward -Infinity(1:w3440) -> (0:w3385:dbl)
            n1686 = Round Toward -Infinity(1:w3431) -> (0:w3384:dbl)
            n1687 = To Long Integer(number=w3383) -> (32bit integer=w3423:i32)
            n1688 = Divide(x=w3378, y=8.0) -> (x/y=w3375:dbl)
            n1689 = To Long Integer(number=w3382) -> (32bit integer=w3468:i32)
            n1690 = To Long Integer(number=w3387) -> (32bit integer=w3458:i32)
            n1691 = To Long Integer(number=w3386) -> (32bit integer=w3450:i32)
            n1692 = To Long Integer(number=w3385) -> (32bit integer=w3441:i32)
            n1693 = To Long Integer(number=w3384) -> (32bit integer=w3432:i32)
            n1694 = And(x=w3423, y=1 ("index")) -> (x .and. y?=w3420:i32)
            n1695 = Multiply(x=100.0, y=w3375) -> (x*y=→"M_COG_Limit":dbl)
            n1696 = Equal?(x=w3420, y=1 ("index")) -> (x = y?=→"SensorBox_Front_RangeCheck":bool)
            n1697 = And(x=w3468, y=1 ("index")) -> (x .and. y?=w3464:i32)
            n1698 = And(x=w3458, y=1 ("index")) -> (x .and. y?=w3456:i32)
            n1699 = And(x=w3450, y=1 ("index")) -> (x .and. y?=w3447:i32)
            n1700 = And(x=w3441, y=1 ("index")) -> (x .and. y?=w3438:i32)
            n1701 = And(x=w3432, y=1 ("index")) -> (x .and. y?=w3429:i32)
            n1702 = Equal?(x=w3464, y=1 ("index")) -> (x = y?=→"Power_Control":bool)
            n1703 = Equal?(x=w3456, y=1 ("index")) -> (x = y?=→"Fx_Divide_ON":bool)
            n1704 = Equal?(x=w3447, y=1 ("index")) -> (x = y?=→"Yaw_Control_ON":bool)
            n1705 = Equal?(x=w3438, y=1 ("index")) -> (x = y?=→"Sensorbox_Plausibility_Check":bool)
            n1706 = Equal?(x=w3429, y=1 ("index")) -> (x = y?=→"SensorBox_Rear_RangeCheck":bool)
            "Array" <- w3393
          }
          frame 1158 {
            n1707 = Index Array(array=w3487, index=2) -> (element=→"Brake_Threshold":u8)
            n1708 = Index Array(array=w3487, index=3) -> (element=→"TC_Param":u8)
            n1709 = Index Array(array=w3487, index=4) -> (element=→"Fx_Bias":u8)
            n1710 = Index Array(array=w3487, index=5) -> (element=→"Rear_Reduction":u8)
            n1711 = Index Array(array=w3487, index=7) -> (element=→"Negative Torque Demand":u8)
            n1712 = Index Array(array=w3487, index=6) -> (element=→"BrakeForce":u8)
            n1713 = Index Array(array=w3487, index=8) -> (element=→"Raw Negative Torque":u8)
          }
          frame 1184 {
            # "Charger Status"
            n1714 = Index Array(array=w3515, index=3) -> (element=w3516:u8)
            n1715 = Number To Boolean Array(number=w3516) -> (Boolean array=w3514:bool[])
            n1716 = Index Array(array=w3514, index #1=7 ("index"), index #2=6 ("index"), index #3=5 ("index"), index #4=4 ("index"), index #5=3 ("index"), index #6=2 ("index"), index #7=1 ("index")) -> ()  [unwired: 7 out]
          }
          frame 1185 {
            # "Charger Status 2"
            n1717 = Index Array(array=w3539, index=8) -> (element=w3541:u8)
            n1718 = Index Array(array=w3539, index=9) -> (element=w3540:u8)
            n1719 = Index Array(array=w3539, index=2) -> (element=w3558:u8)
            n1720 = Index Array(array=w3539, index=3) -> (element=w3557:u8)
            n1721 = Index Array(array=w3539, index=6) -> (element=w3545:u8)
            n1722 = Index Array(array=w3539, index=7) -> (element=w3544:u8)
            n1723 = Index Array(array=w3539, index=4) -> (element=w3549:u8)
            n1724 = Index Array(array=w3539, index=5) -> (element=w3548:u8)
            n1725 = Join Numbers(hi=w3541, lo=w3540) -> ((hi.lo)=w3527:u16)
            n1726 = Join Numbers(hi=w3558, lo=w3557) -> ((hi.lo)=w3536:u16)
            n1727 = Join Numbers(hi=w3545, lo=w3544) -> ((hi.lo)=w3530:u16)
            n1728 = Join Numbers(hi=w3549, lo=w3548) -> ((hi.lo)=w3533:u16)
            n1729 = To Double Precision Float(number=w3527) -> (double precision float=w3528:dbl)
            n1730 = To Double Precision Float(number=w3536) -> (double precision float=w3537:dbl)
            n1731 = To Double Precision Float(number=w3530) -> (double precision float=w3531:dbl)
            n1732 = To Double Precision Float(number=w3533) -> (double precision float=w3534:dbl)
            n1733 = Divide(x=w3528, y=10.0) -> (x/y=→"Voltage Limit":dbl)
            n1734 = Divide(x=w3531, y=10.0) -> (x/y=→"Charge Voltage":dbl)
            n1735 = Divide(x=w3537, y=100.0) -> (x/y=→"Charge Curr":dbl)
            n1736 = Divide(x=w3534, y=100.0) -> (x/y=→"Current Limit":dbl)
          }
          frame 1638 {
            n1737 = Index Array(array=w3566, index=4) -> (element=w3572:u8)
            n1738 = Index Array(array=w3566, index=5) -> (element=w3571:u8)
            n1739 = Index Array(array=w3566, index=2) -> (element=w3576:u8)
            n1740 = Index Array(array=w3566, index=3) -> (element=w3575:u8)
            n1741 = Join Numbers(hi=w3572, lo=w3571) -> ((hi.lo)=w3569:u16)
            n1742 = Join Numbers(hi=w3576, lo=w3575) -> ((hi.lo)=w3570:u16)
            n1743 = To Word Integer(number=w3569) -> (16bit integer=→"PPS1":i16)
            n1744 = To Word Integer(number=w3570) -> (16bit integer=→"PPS2":i16)
          }
          frame 1639 {
            n1745 = Index Array(array=w3587, index=2) -> (element=w3599:u8)
            n1746 = Number To Boolean Array(number=w3599) -> (Boolean array=w3609:bool[])
            n1747 = Index Array(array=w3609, index #1=0 ("index"), index #2=1 ("index"), index #3=2 ("index"), index #4=3 ("index"), index #5=4 ("index"), index #6=5 ("index"), index #7=6 ("index"), index #8=7 ("index")) -> (element #1=w3598:bool, element #2=w3597:bool, element #3=w3596:bool, element #4=w3593:bool, element #5=w3592:bool, element #6=w3590:bool, element #7=w3589:bool, element #8=w3588:bool)
            n1748 = Build Array(w3598, w3597, w3596) -> (w3595:bool[])
            n1749 = Build Array(w3590, w3589, w3588) -> (w3591:bool[])
            n1750 = Build Array(w3593, w3592) -> (w3594:bool[])
            n1751 = Boolean Array To Number(Boolean array=w3595) -> (number=→"ASSI":u32)
            n1752 = Boolean Array To Number(Boolean array=w3594) -> (number=→"EBS":u32)
            n1753 = Boolean Array To Number(Boolean array=w3591) -> (number=→"AMI":u32)
          }
        }
      }
      n1754 = Empty Array?(array=w131) -> (empty?=w125:bool)
      n1755 = feedback-in #48(w125) -> ()
      n1756 = feedback #48(TRUE ("empty?")) -> (w127:bool)
      n1757 = Not(x=w127) -> (.not. x?=w129:bool)
      n1758 = And(x=w129, y=w125) -> (x .and. y?=w130:bool)
      n1759 = Not(x=w125) -> (.not. x?=w126:bool)
      n1760 = And(x=w127, y=w126) -> (x .and. y?=w128:bool)
      n1761 = case shown="True" w130 {
        frame False {
        }
        frame True {
          n1762 = property on="Tab Control" class="TabCtl (strict)"("FG Color"=u32 16711680 ("Colors:FG Color")) -> ()  [unwired: 2 in, 2 out]
        }
      }
      n1763 = case shown="True" w128 {
        frame False {
        }
        frame True {
          n1764 = property on="Tab Control" class="TabCtl (strict)"("FG Color"=u32 11776947 ("Colors:FG Color")) -> ()  [unwired: 2 in, 2 out]
        }
      }
      n1765 = flat-sequence {
        tunnel: w140 -> [w289]
        tunnel: w131 -> [w290]
        frame #0 {
          "CAN ID" <- w289
          "CAN Message" <- w290
          "CAN ID 2" <- w289
          "CAN Message 2" <- w290
          "CAN ID 3" <- w289
          "CAN Message 3" <- w290
        }
      }
      n1766 = property on="T Motor FR [°C]" class="DigNum (strict)"() -> ("Value"=w108:dbl)  [unwired: 2 in, 2 out]
      n1767 = property on="T Inv. RR [°C]" class="DigNum (strict)"() -> ("Value"=w102:dbl)  [unwired: 2 in, 2 out]
      n1768 = property on="T Motor RL [°C]" class="DigNum (strict)"() -> ("Value"=w107:dbl)  [unwired: 2 in, 2 out]
      n1769 = property on="T Motor RR [°C]" class="DigNum (strict)"() -> ("Value"=w106:dbl)  [unwired: 2 in, 2 out]
      n1770 = property on="T Inv. FR [°C]" class="DigNum (strict)"() -> ("Value"=w104:dbl)  [unwired: 2 in, 2 out]
      n1771 = property on="T Inv. FL [°C]" class="DigNum (strict)"() -> ("Value"=w105:dbl)  [unwired: 2 in, 2 out]
      n1772 = property on="T Inv. RL [°C]" class="DigNum (strict)"() -> ("Value"=w103:dbl)  [unwired: 2 in, 2 out]
      n1773 = property on="T Motor FL [°C]" class="DigNum (strict)"() -> ("Value"=w109:dbl)  [unwired: 2 in, 2 out]
      n1774 = property on="HV Current" class="DigNum (strict)"() -> ("Value"=w100:dbl)  [unwired: 2 in, 2 out]
      n1775 = Build Array(w109, w108, w107, w106) -> (w110:dbl[])
      n1776 = Build Array(w105, w104, w103, w102) -> (w111:dbl[])
      n1777 = property on="SoC [mAh]" class="DigNum (strict)"() -> ("Value"=w101:dbl)  [unwired: 2 in, 2 out]
      n1778 = call "lapdata.vi"("Reset"="Reset", "Laptrigger"="Laptrigger", "InverterTemps"=w111, "MotorTemps"=w110, "Current"=w100, "SoC"=w101) -> ("Inverter Temp"=→"Inverter Temp":cluster{i32[], dbl[]}[], "Motor Temp"=→"Motor Temp":cluster{i32[], dbl[]}[], "Lap                    Laptime                        SoC                 Current Avg |                             Motor Temperatures                          |                               Inverter Temperatures"=→"Lap                    Laptime                        SoC                 Current Avg |                             Motor Temperatures                            |                            Inverter Temperatures":T12)  [unwired: 3 in]
    }
    n1779 = local read "Exit"() -> (w8:bool)
  }
  n1780 = control-ref of="This VI"() -> (w4:refnum<vi>)
  n1781 = node-c288(i64 100 ("Period")) -> (w3:T21)  [unwired: 3 in]
  n1782 = invoke class="VI" method="Default Vals.Reinit All"(reference=w4) -> ()  [unwired: 2 in, 3 out]
  n1783 = timed-loop {
    timing: w3 -> [_]
    timing-out: [_] -> w2
    stop <- _ stop-if-true
    w3618 = dbl[] []
    w3620 = 0.03
    n1784 = node-c288() -> ()  [unwired: 1 in, 1 out]
    n1785 = local read "Cones1 2"() -> (w3616:T1)
    n1786 = local read "Cones2 2"() -> (w3614:T1)
    n1787 = local read "Cones3 2"() -> (w3615:T1)
    n1788 = Build Array (concatenate)(w3616, w3614, w3615) -> (w3617:T1)
    n1789 = for {
      tunnel: w3617 -> [w3642] mode=indexing
      shift-right: [w3654] -> w3634
      shift-left: w3618 -> [w3648]
      shift-right: [w3653] -> w3632
      shift-left: w3618 -> [w3647]
      shift-right: [w3652] -> w3630
      shift-left: w3618 -> [w3646]
      shift-right: [w3650] -> w3628
      shift-left: w3618 -> [w3645]
      shift-right: [w3651] -> w3626
      shift-left: w3618 -> [w3644]
      shift-right: [w3649] -> w3624
      shift-left: w3618 -> [w3643]
      n1790 = Unbundle By Name(w3642) -> ("Cluster.Col"=w3655:dbl, "Cluster.X"=w3641:dbl, "Cluster.Y"=w3640:dbl)
      n1791 = To Unsigned Byte Integer(number=w3655) -> (unsigned 8bit integer=w3656:u8)
      n1792 = To Unsigned Long Integer(number=w3641) -> (unsigned 32bit integer=w3639:u32)
      n1793 = To Unsigned Long Integer(number=w3640) -> (unsigned 32bit integer=w3638:u32)
      n1794 = Not Equal To 0?(x=w3639) -> (x != 0?=w3636:bool)
      n1795 = Not Equal To 0?(x=w3638) -> (x != 0?=w3637:bool)
      n1796 = Or(x=w3636, y=w3637) -> (x .or. y?=w3635:bool)
      n1797 = case shown="True" w3635 {
        tunnel: w3656 -> [_ w3677]
        tunnel: w3641 -> [_ w3676]
        tunnel: w3640 -> [_ w3675]
        tunnel: [w3662 w3674] -> w3654
        tunnel: [w3661 w3673] -> w3653
        tunnel: [w3660 w3672] -> w3652
        tunnel: [w3658 w3671] -> w3651
        tunnel: [w3659 w3670] -> w3650
        tunnel: [w3657 w3669] -> w3649
        tunnel: w3648 -> [w3662 w3668]
        tunnel: w3647 -> [w3661 w3667]
        tunnel: w3646 -> [w3660 w3666]
        tunnel: w3645 -> [w3659 w3665]
        tunnel: w3644 -> [w3658 w3664]
        tunnel: w3643 -> [w3657 w3663]
        frame False {
        }
        frame True {
          n1798 = case shown="0" w3677 {
            tunnel: w3676 -> [_ w3691 w3701 w3711]
            tunnel: w3675 -> [_ w3690 w3700 w3710]
            tunnel: [w3683 w3693 w3697 w3707] -> w3674
            tunnel: [w3681 w3686 w3696 w3713] -> w3672
            tunnel: [w3682 w3687 w3703 w3706] -> w3673
            tunnel: [w3680 w3692 w3695 w3705] -> w3670
            tunnel: [w3678 w3684 w3694 w3712] -> w3669
            tunnel: [w3679 w3685 w3702 w3704] -> w3671
            tunnel: w3668 -> [w3683 w3689 w3697 w3707]
            tunnel: w3667 -> [w3682 w3687 w3699 w3706]
            tunnel: w3666 -> [w3681 w3686 w3696 w3709]
            tunnel: w3665 -> [w3680 w3688 w3695 w3705]
            tunnel: w3664 -> [w3679 w3685 w3698 w3704]
            tunnel: w3663 -> [w3678 w3684 w3694 w3708]
            frame 5, Default {
            }
            frame 1 {
              n1799 = Build Array (concatenate)(w3690, w3688) -> (w3692:dbl[])
              n1800 = Build Array (concatenate)(w3691, w3689) -> (w3693:dbl[])
            }
            frame 0 {
              n1801 = Build Array (concatenate)(w3700, w3698) -> (w3702:dbl[])
              n1802 = Build Array (concatenate)(w3701, w3699) -> (w3703:dbl[])
            }
            frame 2, 3 {
              n1803 = Build Array (concatenate)(w3710, w3708) -> (w3712:dbl[])
              n1804 = Build Array (concatenate)(w3711, w3709) -> (w3713:dbl[])
            }
          }
        }
      }
    }
    n1805 = call "Convert to Dynamic Data4"("Array"=w3628) -> ("Dynamic Data Type"=w3627:dynamicdata)  [unwired: 3 in]
    n1806 = call "Convert to Dynamic Data5"("Array"=w3626) -> ("Dynamic Data Type"=w3625:dynamicdata)  [unwired: 3 in]
    n1807 = call "Convert to Dynamic Data6"("Array"=w3624) -> ("Dynamic Data Type"=w3623:dynamicdata)  [unwired: 3 in]
    n1808 = call "Convert to Dynamic Data"("Array"=w3634) -> ("Dynamic Data Type"=w3633:dynamicdata)  [unwired: 3 in]
    n1809 = call "Convert to Dynamic Data2"("Array"=w3632) -> ("Dynamic Data Type"=w3631:dynamicdata)  [unwired: 3 in]
    n1810 = call "Convert to Dynamic Data3"("Array"=w3630) -> ("Dynamic Data Type"=w3629:dynamicdata)  [unwired: 3 in]
    n1811 = Merge Signals(w3627, w3625, w3623) -> (w3621:dynamicdata)
    n1812 = Merge Signals(w3633, w3631, w3629) -> (w3622:dynamicdata)
    n1813 = Multiply(x=w3620, y=w3621) -> (x*y=w3619:dynamicdata)
    n1814 = Multiply(x=w3622, y=w3620) -> (x*y=w3613:dynamicdata)
    n1815 = Decrement(x=w3613) -> (x-1=w3612:dynamicdata)
    n1816 = Decrement(x=w3612) -> (x-1=w3611:dynamicdata)
    n1817 = Decrement(x=w3611) -> (x-1=w3610:dynamicdata)
    n1818 = call "Build XY Graph"("Y Input"=w3610, "X Input"=w3619) -> ()  [unwired: 8 in, 2 out]
    n1819 = node-c288() -> ()  [unwired: 1 in, 1 out]
  }
  n1820 = node-c288(w2) -> ()  [unwired: 1 out]
